vi "Teperature and FIeld Sweep_1022D.vi"() -> ()   [LabVIEW 2022 SP3]
uses:
  <vilib>/Analysis/baseanly.llb/Mean (DBL).vi
  <vilib>/Utility/file.llb/Write Delimited Spreadsheet (DBL).vi
  <vilib>/Analysis/NI_AALBase.lvlib
panel:
  out "Ri_2 phase":cluster{dbl[], dbl[]}(graph)={[0.09999999999999998, 0.12, 0.14, 0.16000000000000003, 0.17999999999999994, 0.19999999999999996, 0.21999999999999997, 0.24, 0.26, 0.28, 0.29999999999999993, 0.31999999999999995, 0.33999999999999997, 0.36, 0.38, 0.4, 0.42000000000000004, 0.43999999999999995, 0.45999999999999996, 0.48, 0.5, 0.52, 0.54, 0.56, 0.5800000000000001, 0.6, 0.62, 0.64, 0.6599999999999999, 0.6799999999999999, 0.7, 0.72, 0.74, 0.76, 0.78, 0.8, 0.8200000000000001, 0.84, 0.86, 0.88, 0.9, 0.92, 0.94, 0.96, 0.98, 1.0, 0.98, 0.96, 0.94, 0.92, 0.9, 0.88, 0.86, 0.84, 0.82, 0.8, 0.78, 0.76, 0.74, 0.72, 0.7, 0.6799999999999999, 0.66, 0.64, 0.62, 0.6, 0.58, 0.56, 0.54, 0.52, 0.5, 0.48, 0.45999999999999996, 0.44000000000000006, 0.42000000000000004, 0.4, 0.38, 0.36, 0.33999999999999997, 0.32, 0.30000000000000004, 0.28, 0.26, 0.24000000000000002, 0.22, 0.2, 0.18, 0.16, 0.14, 0.12000000000000001, 0.1, 0.09999999999999998, 0.12, 0.14, 0.16000000000000003, 0.17999999999999994, 0.19999999999999996, 0.21999999999999997, 0.24, 0.26, 0.28, 0.29999999999999993, 0.31999999999999995, 0.33999999999999997, 0.36, 0.38, 0.4, 0.42000000000000004, 0.43999999999999995, 0.45999999999999996, 0.48, 0.5, 0.52, 0.54, 0.56, 0.5800000000000001, 0.6, 0.62, 0.64, 0.6599999999999999, 0.6799999999999999, 0.7, 0.72, 0.74, 0.76, 0.78, 0.8, 0.8200000000000001, 0.84, 0.86, 0.88, 0.9, 0.92, 0.94, 0.96, 0.98, 1.0, 0.98, 0.96, 0.94, 0.92, 0.9, 0.88, 0.86, 0.84, 0.82, 0.8, 0.78, 0.76, 0.74, 0.72, 0.7, 0.6799999999999999, 0.66, 0.64, 0.62, 0.6, 0.58, 0.56, 0.54, 0.52, 0.5, 0.48, 0.45999999999999996, 0.44000000000000006, 0.42000000000000004, 0.4, 0.38, 0.36, 0.33999999999999997, 0.32, 0.30000000000000004, 0.28, 0.26, 0.24000000000000002, 0.22, 0.2, 0.18, 0.16, 0.14, 0.12000000000000001, 0.1], [117.62016846841588, 117.96664882272376, 118.35478696482726, 118.61912016643541, 118.76956664586604, 118.95054910823121, 119.01498123375443, 119.16872489157113, 119.24431424706378, 119.34190104277982, 119.41733225392822, 119.45140264855945, 119.53984114559682, 119.55691764422741, 119.59487520871042, 119.6750795139146, 119.68579169001923, 119.73065237331134, 119.74423324815396, 119.7661994334273, 119.80750346193834, 119.83623494650696, 119.82452268397942, 119.85627567058157, 119.86835371539776, 119.89360726965279, 119.90311700886441, 119.93603473890582, 119.94528450180692, 119.95000862999613, 119.95960465948625, 119.9830178122235, 119.97849406894788, 119.98959200475136, 119.99632464219606, 119.98257095958301, 120.01347012367368, 120.03103870555512, 120.04478039338926, 120.06360222149044, 120.05061637114048, 120.06363439063853, 120.07171311867637, 120.0757793318229, 120.09113199025303, 120.10726896331157, 120.06234962658894, 120.07718932923174, 120.09075423852748, 120.08476253619433, 120.05873660804704, 120.07529089338618, 120.07073006886651, 120.06602997484751, 120.06644594382928, 120.05437893498467, 120.0559832066358, 120.05241197254445, 120.03496471192462, 120.04190874507303, 120.04592984925304, 120.02590122679835, 120.02106762290221, 120.0170754772018, 120.01717601945583, 119.99024830583144, 119.98050754517847, 119.98548510957906, 119.96626810243879, 119.94421874372571, 119.91496186190318, 119.90254071057821, 119.89802448935203, 119.86225587700838, 119.84782030921231, 119.76071599522875, 119.78171218684165, 119.52712081973637, 119.68947818038498, 119.64888776868774, 119.54538024283588, 119.49187757183782, 119.40373568864177, 119.34094898550048, 119.25703379849283, 119.03268380413638, 118.93848534047406, 118.66368000738926, 118.3703709122756, 118.00894457485364, 117.8022869674905, 117.83191820734878, 118.35839994290589, 118.74306406859516, 118.97978381368443, 119.0832443256442, 119.22408053378842, 119.3756798875886, 119.42654507577663, 119.54312088447948, 119.65528936579355, 119.68067384348709, 119.73888591320637, 119.7746550722424, 119.83575660206921, 119.87436287491752, 119.92090575023776, 119.96360858392154, 119.97618916031327, 120.0270490763764, 120.03660757353578, 120.04594971613244, 120.07374861282088, 120.08502945701846, 120.11904718233538, 120.12373738373853, 120.13187955586031, 120.15078785675374, 120.16051712055169, 120.18138633972099, 120.18855573342282, 120.20283710115059, 120.21752926335739, 120.2286670939815, 120.25005622275296, 120.26083012867937, 120.26435687292016, 120.25219743715516, 120.27247788976976, 120.27728128431886, 120.30980987455453, 120.3013104315504, 120.30956542774932, 120.32575192936613, 120.32481345899741, 120.34376176879596, 120.32045496743885, 120.31980339045367, 120.31350527912403, 120.31252525198906, 120.3242014431218, 120.34462619894298, 120.32098729633576, 120.3242809008918, 120.31759933903815, 120.34279447419958, 120.29133105012681, 120.2971043007052, 120.2915107827317, 120.30887402170481, 120.3132908103599, 120.29180381456831, 120.29677581115975, 120.25488350003204, 120.25012405536286, 120.24749071884021, 120.20434065293489, 120.23689420155657, 120.20258149493482, 120.19465503125453, 120.16140368284456, 120.17158365673114, 120.12877813062116, 120.10707856478476, 120.07296661494834, 120.03335070293379, 120.02574871514983, 119.97110769112416, 120.18824358128647, 119.87610802993717, 119.85772779265321, 119.77209829112437, 119.73583766352138, 119.65849570448214, 119.57056721383769, 119.43100181965622, 119.2628284467831, 119.0562851102115, 118.80762144883226, 118.56712932086603, 117.71722366335914, 116.41351313841975, 116.41351313841975]}
  out "Ri_1 phase":cluster{dbl[], dbl[]}(graph)={[0.09999999999999998, 0.12, 0.14, 0.16000000000000003, 0.17999999999999994, 0.19999999999999996, 0.21999999999999997, 0.24, 0.26, 0.28, 0.29999999999999993, 0.31999999999999995, 0.33999999999999997, 0.36, 0.38, 0.4, 0.42000000000000004, 0.43999999999999995, 0.45999999999999996, 0.48, 0.5, 0.52, 0.54, 0.56, 0.5800000000000001, 0.6, 0.62, 0.64, 0.6599999999999999, 0.6799999999999999, 0.7, 0.72, 0.74, 0.76, 0.78, 0.8, 0.8200000000000001, 0.84, 0.86, 0.88, 0.9, 0.92, 0.94, 0.96, 0.98, 1.0, 0.98, 0.96, 0.94, 0.92, 0.9, 0.88, 0.86, 0.84, 0.82, 0.8, 0.78, 0.76, 0.74, 0.72, 0.7, 0.6799999999999999, 0.66, 0.64, 0.62, 0.6, 0.58, 0.56, 0.54, 0.52, 0.5, 0.48, 0.45999999999999996, 0.44000000000000006, 0.42000000000000004, 0.4, 0.38, 0.36, 0.33999999999999997, 0.32, 0.30000000000000004, 0.28, 0.26, 0.24000000000000002, 0.22, 0.2, 0.18, 0.16, 0.14, 0.12000000000000001, 0.1, 0.09999999999999998, 0.12, 0.14, 0.16000000000000003, 0.17999999999999994, 0.19999999999999996, 0.21999999999999997, 0.24, 0.26, 0.28, 0.29999999999999993, 0.31999999999999995, 0.33999999999999997, 0.36, 0.38, 0.4, 0.42000000000000004, 0.43999999999999995, 0.45999999999999996, 0.48, 0.5, 0.52, 0.54, 0.56, 0.5800000000000001, 0.6, 0.62, 0.64, 0.6599999999999999, 0.6799999999999999, 0.7, 0.72, 0.74, 0.76, 0.78, 0.8, 0.8200000000000001, 0.84, 0.86, 0.88, 0.9, 0.92, 0.94, 0.96, 0.98, 1.0, 0.98, 0.96, 0.94, 0.92, 0.9, 0.88, 0.86, 0.84, 0.82, 0.8, 0.78, 0.76, 0.74, 0.72, 0.7, 0.6799999999999999, 0.66, 0.64, 0.62, 0.6, 0.58, 0.56, 0.54, 0.52, 0.5, 0.48, 0.45999999999999996, 0.44000000000000006, 0.42000000000000004, 0.4, 0.38, 0.36, 0.33999999999999997, 0.32, 0.30000000000000004, 0.28, 0.26, 0.24000000000000002, 0.22, 0.2, 0.18, 0.16, 0.14, 0.12000000000000001, 0.1], [-151.82022434949218, -151.31250474861076, -150.934829382567, -150.48587961112963, -150.35129794100732, -150.20108675684463, -150.07301012387398, -149.85371662190408, -149.80643007097768, -149.6778115966004, -149.70631232196195, -149.3427081876464, -144.00790971737905, -149.75303510022803, -149.67465048111166, -149.61059645892314, -149.5755216627079, -149.56032591732512, -149.56777135196236, -149.53038555798872, -149.4837567137922, -149.46653630858634, -149.4555130589029, -149.44977309701568, -149.46602213201024, -149.42050625632652, -149.44267585686146, -149.44000832559337, -149.42583379539636, -149.39692572431568, -149.40442155131146, -149.40915566881102, -149.38050614114596, -149.38240574949845, -149.3953243906204, -149.3899047221218, -149.38685008550175, -149.37072119411883, -149.37324923858517, -149.36914979835484, -149.37390639605138, -149.3980165878626, -149.38623806135408, -149.35518531108906, -149.37819742529774, -149.37025076997705, -149.37797439572273, -149.4274062049048, -149.39553532551332, -149.39989159256442, -149.40788326839706, -149.4035269042052, -149.42173829217444, -149.42516481564763, -149.4219167404996, -149.46356168834444, -149.4516805103338, -149.45047160544362, -149.45716135037998, -149.47450752769095, -149.4832252279336, -149.49183740199788, -149.51226639630787, -149.525555046651, -149.5573781565128, -149.5590093788641, -149.5858478680793, -149.5557150450339, -149.61888489114702, -149.65084954099694, -149.65437010384474, -149.69488018826033, -149.69116543387327, -149.7564704385459, -149.77576215560174, -149.78827998741025, -150.21783070990878, -156.94726445856756, -149.75208834187845, -149.79358735688876, -149.81920487838278, -149.97644416993913, -150.0531791626578, -150.16748042818656, -150.30076394633943, -150.44483707228213, -150.66626270081673, -151.04929447184827, -151.43411807203063, -151.97278023054187, -152.18821211537258, -152.14623356637654, -151.4719825276092, -150.96302427747355, -150.84756504567386, -150.5037700822142, -150.3245640418613, -150.17713325364664, -150.1036649225191, -149.99036753477975, -149.85697295444248, -149.8501754093205, -149.56080314237312, -146.67158122655187, -149.96749106410877, -149.93190810259412, -149.9232306144384, -149.8834345316244, -149.82170489643204, -149.7789775276986, -149.77872756893103, -149.7707527140453, -149.75157225999848, -149.7012296966859, -149.71638923850873, -149.69938903054089, -149.67312320269653, -149.69041977164406, -149.6838198853977, -149.66161778220618, -149.6546278866485, -149.640923821836, -149.6728863842432, -149.66791865505627, -149.62858582517933, -149.64183587402476, -149.6484558455101, -149.6427424788427, -149.6296817347956, -149.63395082883616, -149.62713187401155, -149.6182616601406, -149.65041315650092, -149.62494744989198, -149.61909696518853, -149.6175044512262, -149.6371509732279, -149.66137383135944, -149.63515614075328, -149.6451064613961, -149.65811060587708, -149.64909805431552, -149.6696824809014, -149.66829454461902, -149.65211834334818, -149.6792564836343, -149.69346020858046, -149.7169451406854, -149.71160254963883, -149.72665337378038, -149.73853617494782, -149.73020826238755, -149.75385526179556, -149.7724664962522, -149.77034769159013, -149.80481526391884, -149.81816596924764, -149.87205062927146, -149.86012342940273, -149.90891882509268, -149.92420949696478, -149.94160073513336, -149.98031714888242, -149.98297286567293, -150.01739729399605, -150.0978801191893, -150.09675943096, -149.9722562160305, -148.8947110005267, -150.0746278787694, -150.12829367372765, -150.21097166683603, -150.2349660580826, -150.3575760488762, -150.49529547074826, -150.72432289368865, -150.81632873807234, -151.05780214090098, -151.3722097867961, -151.68469888569936, -152.04933901054727, -152.04933901054727]}
  out "Ri_2":cluster{dbl[], dbl[]}(graph)={[0.09999999999999998, 0.12, 0.14, 0.16000000000000003, 0.17999999999999994, 0.19999999999999996, 0.21999999999999997, 0.24, 0.26, 0.28, 0.29999999999999993, 0.31999999999999995, 0.33999999999999997, 0.36, 0.38, 0.4, 0.42000000000000004, 0.43999999999999995, 0.45999999999999996, 0.48, 0.5, 0.52, 0.54, 0.56, 0.5800000000000001, 0.6, 0.62, 0.64, 0.6599999999999999, 0.6799999999999999, 0.7, 0.72, 0.74, 0.76, 0.78, 0.8, 0.8200000000000001, 0.84, 0.86, 0.88, 0.9, 0.92, 0.94, 0.96, 0.98, 1.0, 0.98, 0.96, 0.94, 0.92, 0.9, 0.88, 0.86, 0.84, 0.82, 0.8, 0.78, 0.76, 0.74, 0.72, 0.7, 0.6799999999999999, 0.66, 0.64, 0.62, 0.6, 0.58, 0.56, 0.54, 0.52, 0.5, 0.48, 0.45999999999999996, 0.44000000000000006, 0.42000000000000004, 0.4, 0.38, 0.36, 0.33999999999999997, 0.32, 0.30000000000000004, 0.28, 0.26, 0.24000000000000002, 0.22, 0.2, 0.18, 0.16, 0.14, 0.12000000000000001, 0.1, 0.09999999999999998, 0.12, 0.14, 0.16000000000000003, 0.17999999999999994, 0.19999999999999996, 0.21999999999999997, 0.24, 0.26, 0.28, 0.29999999999999993, 0.31999999999999995, 0.33999999999999997, 0.36, 0.38, 0.4, 0.42000000000000004, 0.43999999999999995, 0.45999999999999996, 0.48, 0.5, 0.52, 0.54, 0.56, 0.5800000000000001, 0.6, 0.62, 0.64, 0.6599999999999999, 0.6799999999999999, 0.7, 0.72, 0.74, 0.76, 0.78, 0.8, 0.8200000000000001, 0.84, 0.86, 0.88, 0.9, 0.92, 0.94, 0.96, 0.98, 1.0, 0.98, 0.96, 0.94, 0.92, 0.9, 0.88, 0.86, 0.84, 0.82, 0.8, 0.78, 0.76, 0.74, 0.72, 0.7, 0.6799999999999999, 0.66, 0.64, 0.62, 0.6, 0.58, 0.56, 0.54, 0.52, 0.5, 0.48, 0.45999999999999996, 0.44000000000000006, 0.42000000000000004, 0.4, 0.38, 0.36, 0.33999999999999997, 0.32, 0.30000000000000004, 0.28, 0.26, 0.24000000000000002, 0.22, 0.2, 0.18, 0.16, 0.14, 0.12000000000000001, 0.1], [12.205176752147196, 12.33738736524411, 12.436814472113113, 12.543061919618381, 12.591177109870843, 12.63204488402351, 12.633074379656962, 12.678587031476285, 12.702366812156168, 12.734766256641889, 12.764822745445459, 12.798115074151369, 12.56005416503157, 12.811022273559901, 12.805614848037402, 12.822742652741233, 12.833360063934796, 12.844414076677566, 12.853037374725659, 12.863749846343488, 12.873727971040198, 12.87545677652524, 12.884395543563812, 12.901595012846315, 12.91020558633629, 12.91700210310611, 12.916182386400777, 12.932745625307929, 12.929132177243485, 12.939245398543807, 12.945904132779514, 12.979271768015096, 12.951619927398129, 12.963100847085817, 12.961454764152798, 12.968676853276186, 13.035314574413999, 12.968769140450755, 12.976857768700619, 12.982937075765706, 12.987156955464599, 12.987225357622929, 12.990469558247861, 13.001074140628084, 13.015805070701896, 13.213316441028162, 13.212674850256546, 13.214497097772925, 13.213097914485022, 13.212520778890907, 13.217287379489568, 13.224571659209413, 13.221461422183241, 13.21249046212996, 13.231625931101464, 13.219596872719654, 13.230780717880945, 13.231496283261466, 13.228879184378412, 13.236537684484286, 13.2442021665191, 13.245327395573094, 13.239075527873267, 13.250459225400578, 13.254010022147359, 13.263592058540043, 13.278201777756056, 13.271280645160415, 13.28286228675346, 13.287261154844275, 13.290082368268422, 13.30492697157085, 13.325287026560359, 13.337097306813405, 13.334459335710374, 13.36121908059594, 13.349781951942722, 13.590657500379482, 13.420711749521754, 13.427055186068772, 13.476488972924022, 13.504746276159453, 13.521802810703734, 13.585085247505193, 13.63738342595085, 13.703337851038048, 13.791442558469074, 13.849252925446702, 13.98837153260088, 14.058767459755813, 13.057484778983863, 12.424975150602982, 12.341214474536581, 12.597671651852279, 12.547100753140823, 12.603242737801498, 12.610091337495355, 12.662729976248402, 12.683644441406994, 12.707706571670649, 12.74751634316906, 12.764099115085513, 12.803871979165852, 12.693242845243883, 12.809727121728208, 12.817180050708686, 12.831651755770647, 12.839364718018068, 12.860298160932963, 12.896827552552299, 12.864701328486037, 12.883685199780242, 12.884793998467885, 12.902011985965638, 12.898401964032054, 12.906219259474547, 12.914228868687658, 12.911587003388147, 12.958793693981802, 12.933506906195795, 12.933859306721546, 12.94206688909155, 12.946106387292451, 12.954120795402451, 12.95420497189929, 12.961692049093307, 12.970243175218398, 12.966251377610806, 12.971030269555348, 12.980713661496962, 12.983816343381182, 12.98792173316417, 12.995117688102317, 13.000724459135895, 13.003773018187172, 13.013804312695264, 13.221409487304983, 13.213732944734987, 13.219930146403511, 13.2160660705417, 13.220288758106749, 13.225356431589839, 13.221627768983318, 13.192042140412925, 13.225457206093656, 13.224404733921627, 13.226943621029603, 13.22188486286242, 13.239906219746997, 13.23627215525837, 13.23780083001927, 13.24191338088606, 13.243188029364342, 13.248586751116793, 13.24553444444596, 13.263702564618967, 13.263180218458823, 13.265510887371871, 13.27580985473867, 13.285902114226138, 13.285290341366075, 13.292004389335341, 13.320520276023231, 13.32468083832859, 13.320587416172566, 13.3596713753944, 13.351640175534053, 13.311511157505569, 13.749204463952886, 13.417895997650705, 13.439008654275602, 13.464312581366862, 13.491545253041302, 13.546146393015691, 13.560171412898399, 13.584913714835219, 13.647701856221694, 13.605003489243288, 13.892818025978201, 13.94644999851722, 14.42599048649726, 102.36268705136854, 102.36268705136854]}
  out "Ri_1":cluster{dbl[], dbl[]}(graph)={[0.09999999999999998, 0.12, 0.14, 0.16000000000000003, 0.17999999999999994, 0.19999999999999996, 0.21999999999999997, 0.24, 0.26, 0.28, 0.29999999999999993, 0.31999999999999995, 0.33999999999999997, 0.36, 0.38, 0.4, 0.42000000000000004, 0.43999999999999995, 0.45999999999999996, 0.48, 0.5, 0.52, 0.54, 0.56, 0.5800000000000001, 0.6, 0.62, 0.64, 0.6599999999999999, 0.6799999999999999, 0.7, 0.72, 0.74, 0.76, 0.78, 0.8, 0.8200000000000001, 0.84, 0.86, 0.88, 0.9, 0.92, 0.94, 0.96, 0.98, 1.0, 0.98, 0.96, 0.94, 0.92, 0.9, 0.88, 0.86, 0.84, 0.82, 0.8, 0.78, 0.76, 0.74, 0.72, 0.7, 0.6799999999999999, 0.66, 0.64, 0.62, 0.6, 0.58, 0.56, 0.54, 0.52, 0.5, 0.48, 0.45999999999999996, 0.44000000000000006, 0.42000000000000004, 0.4, 0.38, 0.36, 0.33999999999999997, 0.32, 0.30000000000000004, 0.28, 0.26, 0.24000000000000002, 0.22, 0.2, 0.18, 0.16, 0.14, 0.12000000000000001, 0.1, 0.09999999999999998, 0.12, 0.14, 0.16000000000000003, 0.17999999999999994, 0.19999999999999996, 0.21999999999999997, 0.24, 0.26, 0.28, 0.29999999999999993, 0.31999999999999995, 0.33999999999999997, 0.36, 0.38, 0.4, 0.42000000000000004, 0.43999999999999995, 0.45999999999999996, 0.48, 0.5, 0.52, 0.54, 0.56, 0.5800000000000001, 0.6, 0.62, 0.64, 0.6599999999999999, 0.6799999999999999, 0.7, 0.72, 0.74, 0.76, 0.78, 0.8, 0.8200000000000001, 0.84, 0.86, 0.88, 0.9, 0.92, 0.94, 0.96, 0.98, 1.0, 0.98, 0.96, 0.94, 0.92, 0.9, 0.88, 0.86, 0.84, 0.82, 0.8, 0.78, 0.76, 0.74, 0.72, 0.7, 0.6799999999999999, 0.66, 0.64, 0.62, 0.6, 0.58, 0.56, 0.54, 0.52, 0.5, 0.48, 0.45999999999999996, 0.44000000000000006, 0.42000000000000004, 0.4, 0.38, 0.36, 0.33999999999999997, 0.32, 0.30000000000000004, 0.28, 0.26, 0.24000000000000002, 0.22, 0.2, 0.18, 0.16, 0.14, 0.12000000000000001, 0.1], [2087.542522514706, 2143.3806726181297, 2192.1505680332307, 2224.5398110134415, 2254.2076727564463, 2283.219391571736, 2295.5351896243988, 2312.274969759326, 2321.1906487058636, 2258.618428233254, 2439.815278150036, 2363.114732601407, 2569.2987357483867, 2366.69462809311, 2370.3526096767628, 2370.7532832147513, 2369.446453774161, 2372.3479615014453, 2373.7967150363133, 2373.3912011059742, 2374.3898629584414, 2373.19922105906, 2374.08711510194, 2374.3447992304204, 2372.719181172187, 2372.5831623830313, 2368.606666524962, 2368.1271954116123, 2368.1587157781582, 2368.364263936688, 2363.1239774166042, 2363.4322755470225, 2359.5286066627255, 2362.2730811990377, 2355.540999658394, 2354.6901938211345, 2338.3987997031136, 2348.956030561271, 2348.6720464600826, 2345.47931492513, 2343.641628918994, 2322.579102266805, 2357.7528780540633, 2337.9624461876765, 2337.035655864342, 2390.13340514578, 2393.333076080936, 2397.194891434832, 2400.4646152722025, 2404.1840381335187, 2406.4647119031993, 2411.655350773428, 2414.452737749684, 2416.491207784975, 2422.152414810807, 2426.43445652573, 2430.4661399145198, 2472.9095612064084, 2401.2074203638863, 2442.381915486605, 2447.39053615182, 2448.9505311169605, 2454.873847352734, 2458.903517524707, 2461.995925756737, 2467.061840825975, 2470.520942891029, 2474.931087852616, 2483.997180170197, 2486.4806066909064, 2489.8094006815363, 2495.4829515630936, 2496.5109281850623, 2499.717712613259, 2508.0628602511415, 2587.583625405099, 2446.457085912187, 2744.1467541037973, 2527.145831911331, 2528.3781519262234, 2531.0945072462814, 2536.7135748602786, 2544.038687449601, 2544.827299932163, 2546.39588450735, 2552.3831526464273, 2560.7487646591876, 2557.6068386083666, 2541.8036010528517, 2556.5211525031086, 2275.4515181505535, 2236.3211050589766, 2137.0989873521185, 2148.4934229155265, 2226.3795783020046, 2259.8236048661397, 2277.518588977397, 2298.2309636749364, 2311.745843167506, 2328.4510173480307, 2336.560722824512, 2344.24126014681, 2362.7311144000346, 2627.003456834187, 2364.144130172327, 2369.8717620699094, 2373.0451002371196, 2373.971931289017, 2377.1037991880976, 2381.4533155017552, 2376.2465418035545, 2376.4643282086604, 2373.1094722464964, 2373.683408097068, 2373.6902390420423, 2372.436584742077, 2372.7068819175765, 2370.444178339574, 2369.7303118006134, 2368.9013786355426, 2364.66910807676, 2363.1277468576277, 2362.1693752579, 2359.8572707523836, 2358.3637082703754, 2356.2088803095526, 2354.2381091107436, 2352.2504633571566, 2349.807036392201, 2348.000550307495, 2345.2605399911095, 2343.048947126772, 2342.138893566093, 2338.647207375316, 2337.823575605664, 2336.4325858086618, 2391.3050818760403, 2393.854078139158, 2397.3144621611436, 2400.183701016868, 2404.559873121706, 2408.113986664911, 2411.3881576090257, 2422.2503149813315, 2418.4477629937755, 2423.424584031643, 2427.359469208306, 2429.5536317154106, 2435.189541439222, 2439.3273653599067, 2443.6532125172207, 2446.4799477219917, 2450.5183688798943, 2455.1086830020786, 2469.17017360265, 2463.7910814680667, 2466.142256138314, 2475.164122601692, 2480.58039686262, 2485.3434347885513, 2489.254932267259, 2490.995762828881, 2496.288772114335, 2501.89872487851, 2502.665922214194, 2507.8176213420734, 2510.8951882690485, 2514.6646388029453, 2515.90870103181, 2526.343933365244, 2527.8233287119538, 2535.9588766433053, 2534.614384395244, 2541.4565246972834, 2550.357749348691, 2549.473660870641, 2558.3365999756966, 2604.730472408435, 2561.1991565610233, 2554.929997465301, 2611.611284193903, 2611.611284193903]}
  out "Ri_2(Ohm)":dbl=12.205176752147196
  out "Ri_1(Ohm)":dbl=2087.542522514706
  in  "R2 Sensitivity":u16(ring)=26 items=["1 nV/fA", "2 nV/fA", "5 nV/fA", "10 nV/fA", "20 nV/fA", "50 nV/fA", "100 nV/fA", "200 nV/fA", "500 nV/fA", "1 uV/pA", "2 uV/pA", "5 uV/pA", "10 uV/pA", "20 uV/pA", "50 uV/pA", "100 uV/pA", "200 uV/pA", "500 uV/pA", "1 mV/nA", "2 mV/nA", "5 mV/nA", "10 mV/nA", "20 mV/nA", "50 mV/nA", "100 mV/nA", "200 mV/nA", "500 mV/nA", "1 V/uA"]
  in  "R2 Current T Constant":u8(ring)=9 items=["10 us", "30 us", "100 us", "300 us", "1 ms", "3 ms", "10 ms", "30 ms", "100 ms", "300 ms", "1 s", "3 s", "10 s", "30 s", "100 s", "300 s", "1 ks", "3 ks"]
  in  "R1 Current T Constant":u8(ring)=9 items=["10 us", "30 us", "100 us", "300 us", "1 ms", "3 ms", "10 ms", "30 ms", "100 ms", "300 ms", "1 s", "3 s", "10 s", "30 s", "100 s", "300 s", "1 ks", "3 ks"]
  in  "R1 Current sensitivity":u16(ring)=26 items=["1 nV/fA", "2 nV/fA", "5 nV/fA", "10 nV/fA", "20 nV/fA", "50 nV/fA", "100 nV/fA", "200 nV/fA", "500 nV/fA", "1 uV/pA", "2 uV/pA", "5 uV/pA", "10 uV/pA", "20 uV/pA", "50 uV/pA", "100 uV/pA", "200 uV/pA", "500 uV/pA", "1 mV/nA", "2 mV/nA", "5 mV/nA", "10 mV/nA", "20 mV/nA", "50 mV/nA", "100 mV/nA", "200 mV/nA", "500 mV/nA", "1 V/uA"]
  in  "LOCKIN3 address":refnum<visa-resource-name>="COM5"
  in  "Current measurement?":bool=TRUE
  in  "R2(Kohm)":dbl=1.9997 format="%#_13g"
  in  "R1(Kohm)":dbl=2.0265 format="%#_13g"
  out "Device 1 phase":dbl=-151.82022434949218 format="%.3p"
  out "Device 2 phase":dbl=117.62016846841588 format="%.3p"
  out "Device1 Current(mA)":dbl=0.0003122594054162884
  out "Device2 Current(mA)":dbl=0.015138421665849215
  in  "Sine Output Amplitude (V)":sgl=0.5
  out "Vab_1_F 2w":cluster{dbl[], dbl[]}(graph)
  out "Phase Vab_1_F 2w":cluster{dbl[], dbl[]}(graph)
  out "Vab_1_F (uV) 2w":dbl format="%.3p"
  out "Phase Vab_1_F 2w":dbl format="%.3p"
  in  "Phase 1B 3":u16(ring)=9 items=["X", "Y", "R", "Theta", "Frequency", "Noise", "Xh1", "Yh1", "Rh1", "Theta h1", "Xh2", "Yh2", "Rh2", "Theta h2"]
  in  "Parameter 1B 3":u16(ring)=8 items=["X", "Y", "R", "Theta", "Frequency", "Noise", "Xh1", "Yh1", "Rh1", "Theta h1", "Xh2", "Yh2", "Rh2", "Theta h2"]
  out "Vab_2_F  2w":cluster{dbl[], dbl[]}(graph)
  out "Phase Vab_2_F 2w":cluster{dbl[], dbl[]}(graph)
  out "Vab_2_F (uV) 2w":dbl format="%.3p"
  out "Phase Vab_2_F 2w":dbl format="%.6g"
  in  "Phase 2B 3":u16(ring)=9 items=["X", "Y", "R", "Theta", "Frequency", "Noise", "Xh1", "Yh1", "Rh1", "Theta h1", "Xh2", "Yh2", "Rh2", "Theta h2"]
  in  "Parameter 2B 3":u16(ring)=8 items=["X", "Y", "R", "Theta", "Frequency", "Noise", "Xh1", "Yh1", "Rh1", "Theta h1", "Xh2", "Yh2", "Rh2", "Theta h2"]
  in  "Starting Point (Oe)":dbl
  out "phase Vaa_2_F":cluster{dbl[], dbl[]}(graph)={[0.1], [0.0]}
  out "Vaa_2_F":cluster{dbl[], dbl[]}(graph)={[0.1], [0.0]}
  out "phase Vab_2_F 1w":cluster{dbl[], dbl[]}(graph)
  out "Vab_2_F 1w":cluster{dbl[], dbl[]}(graph)={[0.1], [0.0]}
  out "phase Vab_2_F 1w":dbl
  in  "Phase 2B 2":u16(ring)=3 items=["X", "Y", "R", "Theta", "Frequency", "Noise", "Xh1", "Yh1", "Rh1", "Theta h1", "Xh2", "Yh2", "Rh2", "Theta h2"]
  out "phase Vaa_2_F":dbl
  in  "Phase 2A  2":u16(ring)=3 items=["X", "Y", "R", "Theta", "Frequency", "Noise", "Xh1", "Yh1", "Rh1", "Theta h1", "Xh2", "Yh2", "Rh2", "Theta h2"]
  out "Vaa_2_F (mV)":dbl
  in  "F Clear Plot 2A":bool
  in  "Parameter 2A 2":u16(ring)=2 items=["X", "Y", "R", "Theta", "Frequency", "Noise", "Xh1", "Yh1", "Rh1", "Theta h1", "Xh2", "Yh2", "Rh2", "Theta h2"]
  out "Vab_2_F (uV) 1w":dbl
  in  "F Clear Plot 2B":bool
  in  "Parameter 2B 2":u16(ring)=2 items=["X", "Y", "R", "Theta", "Frequency", "Noise", "Xh1", "Yh1", "Rh1", "Theta h1", "Xh2", "Yh2", "Rh2", "Theta h2"]
  in  "path2 (folder + filename)":string="G:\\My Drive\\Opticool\\Measurement\\TF dependence\\TaI28_A1215_B1211"
  out "XY Graph 8":cluster{dbl[], dbl[]}(graph)={[0.1], [0.0]}
  out "XY Graph 7":cluster{dbl[], dbl[]}(graph)={[0.1], [0.0]}
  out "XY Graph 6":cluster{dbl[], dbl[]}(graph)
  out "XY Graph 5":cluster{dbl[], dbl[]}(graph)={[0.1], [0.0]}
  out "phase 2B":dbl
  in  "Phase 2B":u16(ring)=3 items=["X", "Y", "R", "Theta", "Frequency", "Noise", "Xh1", "Yh1", "Rh1", "Theta h1", "Xh2", "Yh2", "Rh2", "Theta h2"]
  out "phase 2A":dbl
  in  "Phase 2A":u16(ring)=3 items=["X", "Y", "R", "Theta", "Frequency", "Noise", "Xh1", "Yh1", "Rh1", "Theta h1", "Xh2", "Yh2", "Rh2", "Theta h2"]
  out "para2A Measurement":dbl
  in  "T Clear Plot 2A":bool
  in  "Parameter 2A":u16(ring)=2 items=["X", "Y", "R", "Theta", "Frequency", "Noise", "Xh1", "Yh1", "Rh1", "Theta h1", "Xh2", "Yh2", "Rh2", "Theta h2"]
  out "para2B Measurement":dbl
  in  "T Clear Plot 2B":bool
  in  "Parameter 2B":u16(ring)=2 items=["X", "Y", "R", "Theta", "Frequency", "Noise", "Xh1", "Yh1", "Rh1", "Theta h1", "Xh2", "Yh2", "Rh2", "Theta h2"]
  in  "2B frequency 2":dbl=17.7 format="%#_13g"
  in  "2B Input Connection (0: Single-Ended)":u16(ring)=1 items=["Single-Ended Voltage", "Differential Voltage", "1 MOhm Current Gain", "100 MOhm Current Gain"]
  in  "2B harmonic 1":u8=2
  in  "2B harmonic 2":u8=3
  in  "2B reference Manual Phase":dbl
  in  "auto phase 2B":bool=TRUE
  in  "2B Sample time (s)":dbl=0.001 min=0.001 max=100.0 step=0.001
  in  "2B Sensitivity":u16(ring)=26 items=["1 nV/fA", "2 nV/fA", "5 nV/fA", "10 nV/fA", "20 nV/fA", "50 nV/fA", "100 nV/fA", "200 nV/fA", "500 nV/fA", "1 uV/pA", "2 uV/pA", "5 uV/pA", "10 uV/pA", "20 uV/pA", "50 uV/pA", "100 uV/pA", "200 uV/pA", "500 uV/pA", "1 mV/nA", "2 mV/nA", "5 mV/nA", "10 mV/nA", "20 mV/nA", "50 mV/nA", "100 mV/nA", "200 mV/nA", "500 mV/nA", "1 V/uA"]
  in  "Enable Sync Filter 2B (when f<200Hz)":bool
  in  "2B Time Constant":u8(ring)=9 items=["10 us", "30 us", "100 us", "300 us", "1 ms", "3 ms", "10 ms", "30 ms", "100 ms", "300 ms", "1 s", "3 s", "10 s", "30 s", "100 s", "300 s", "1 ks", "3 ks"]
  in  "2B Reference Source":u8(ring) items=["External", "Internal", "Internal Sweep", "Channel-A"]
  in  "2B Low Pass Filter Slope":u8(ring)=2 items=["6 dB/oct", "12 dB/oct", "18 db/oct", "24 dB/oct"]
  in  "2A frequency":dbl=17.7 format="%#_13g"
  in  "2A Input Connection (0: Single-Ended)":u16(ring)=1 items=["Single-Ended Voltage", "Differential Voltage", "1 MOhm Current Gain", "100 MOhm Current Gain"]
  in  "2A harmonic 2":u8=2
  in  "2A harmonic":u8=3
  in  "2A reference Manual Phase":dbl
  in  "auto phase 2A":bool=TRUE
  in  "2A Reference Source":u8(ring) items=["External", "Internal", "Internal Sweep"]
  in  "2A Sample time (s)":dbl=0.001 min=0.001 max=100.0 step=0.001
  in  "2A Time Constant":u8(ring)=9 items=["10 us", "30 us", "100 us", "300 us", "1 ms", "3 ms", "10 ms", "30 ms", "100 ms", "300 ms", "1 s", "3 s", "10 s", "30 s", "100 s", "300 s", "1 ks", "3 ks"]
  in  "Enable Sync Filter 2A (when f<200Hz)":bool
  in  "2A Sensitivity":u16(ring)=26 items=["1 nV/fA", "2 nV/fA", "5 nV/fA", "10 nV/fA", "20 nV/fA", "50 nV/fA", "100 nV/fA", "200 nV/fA", "500 nV/fA", "1 uV/pA", "2 uV/pA", "5 uV/pA", "10 uV/pA", "20 uV/pA", "50 uV/pA", "100 uV/pA", "200 uV/pA", "500 uV/pA", "1 mV/nA", "2 mV/nA", "5 mV/nA", "10 mV/nA", "20 mV/nA", "50 mV/nA", "100 mV/nA", "200 mV/nA", "500 mV/nA", "1 V/uA"]
  in  "2A Low Pass Filter Slope":u8(ring)=2 items=["6 dB/oct", "12 dB/oct", "18 db/oct", "24 dB/oct"]
  in  "Two Lock-in ?":bool=TRUE
  in  "LOCKIN2 address":refnum<visa-resource-name>="COM4"
  in  "?":bool
  out "Temperature Status":i32(ring)=1 items=["TemperatureUnknown"=0, "Stable"=1, "Tracking"=2, "Near"=5, "Chasing"=6, "Filling"=7, "Standby"=10, "Disabled"=13, "ImpedanceNotFunction"=14, "TempFailure"=15]
  out "Field Status":i32(ring)=4 items=["MagnetUnknown"=0, "StablePersistent"=1, "WarmingSwitch"=2, "CoolingSwitch"=3, "StableDriven"=4, "Iterating"=5, "Charging"=6, "Discharging"=7, "CurrentError"=8, "MagnetFailure"=15]
  out "Field":dbl=0.10076643899083138
  out "Temperature":dbl=2.0469605207443236
  in  "Initialize":bool
  in  "System Stablization (s)":dbl=0.5 format="%#_13g"
  in  "Low Value (Oe)":dbl=-66000.0
  in  "High Value (Oe)":dbl=66000.0
  in  "Sweep Field Approach":i32(ring) items=["Linear", "NoOvershoot", "Oscillate"]
  in  "Sweep F Rate (Oe/s)":dbl=200.0 format="%#_13g"
  in  "Sweep F mode":i32(ring) items=["Persistent", "Driven"]
  in  "Set Fixed T":dbl=2.0
  in  "Fixed Temp Approach":i32(ring)=1 items=["FastSettle", "NoOvershoot"]
  in  "FIxed T  Rate (K/min)":dbl=20.0
  out "phase Vaa_1_F":cluster{dbl[], dbl[]}(graph)
  out "Vaa_1_F":cluster{dbl[], dbl[]}(graph)
  out "phase Vab_1_F 1w":cluster{dbl[], dbl[]}(graph)
  out "Vab_1_F 1w":cluster{dbl[], dbl[]}(graph)
  out "phase Vab_1_F 1w":dbl
  in  "Phase 1B 2":u16(ring)=3 items=["X", "Y", "R", "Theta", "Frequency", "Noise", "Xh1", "Yh1", "Rh1", "Theta h1", "Xh2", "Yh2", "Rh2", "Theta h2"]
  out "phase Vaa_1_F":dbl
  in  "Phase 1A 2":u16(ring)=3 items=["X", "Y", "R", "Theta", "Frequency", "Noise", "Xh1", "Yh1", "Rh1", "Theta h1", "Xh2", "Yh2", "Rh2", "Theta h2"]
  out "Vaa_1_F (mV)":dbl=1.49013e-07
  in  "F Clear Plot 1A":bool
  in  "Parameter 1A 2":u16(ring)=2 items=["X", "Y", "R", "Theta", "Frequency", "Noise", "Xh1", "Yh1", "Rh1", "Theta h1", "Xh2", "Yh2", "Rh2", "Theta h2"]
  out "Vab_1_F (uV) 1w":dbl=1.49013e-07
  in  "F Clear Plot 1B":bool
  in  "Parameter 1B 2":u16(ring)=2 items=["X", "Y", "R", "Theta", "Frequency", "Noise", "Xh1", "Yh1", "Rh1", "Theta h1", "Xh2", "Yh2", "Rh2", "Theta h2"]
  out "Field Setting":dbl format="%#_13g"
  out "Fixed Temp":dbl
  out "Measured Field":dbl
  out "Field Status":i32(ring) items=["MagnetUnknown"=0, "StablePersistent"=1, "WarmingSwitch"=2, "CoolingSwitch"=3, "StableDriven"=4, "Iterating"=5, "Charging"=6, "Discharging"=7, "CurrentError"=8, "MagnetFailure"=15]
  out "Temp Status":i32(ring) items=["TemperatureUnknown"=0, "Stable"=1, "Tracking"=2, "Near"=5, "Chasing"=6, "Filling"=7, "Standby"=10, "Disabled"=13, "ImpedanceNotFunction"=14, "TempFailure"=15]
  out "Measuring F":bool
  in  "Step(Oe)":i32=2000
  out "F loop run":i32=1
  out "Temp Status":i32(ring) items=["TemperatureUnknown"=0, "Stable"=1, "Tracking"=2, "Near"=5, "Chasing"=6, "Filling"=7, "Standby"=10, "Disabled"=13, "ImpedanceNotFunction"=14, "TempFailure"=15]
  out "Field Status":i32(ring) items=["MagnetUnknown"=0, "StablePersistent"=1, "WarmingSwitch"=2, "CoolingSwitch"=3, "StableDriven"=4, "Iterating"=5, "Charging"=6, "Discharging"=7, "CurrentError"=8, "MagnetFailure"=15]
  out "Fixed Field":dbl
  out "Measured Temp":dbl
  in  "Delay(T/F)":dbl=5.0
  in  "Set FIxed F (Oe)":dbl format="%#_13g"
  in  "Fixed Field Approach":i32(ring) items=["Linear", "NoOvershoot", "Oscillate"]
  in  "FIxed F Rate (Oe/s)":dbl=100.0 format="%#_13g"
  in  "Fixed F mode":i32(ring) items=["Persistent", "Driven"]
  in  "Sweep Temperature Approach":i32(ring)=1 items=["FastSettle", "NoOvershoot"]
  in  "Sweep T  Rate (K/min)":dbl=10.0
  in  "Sweep T/F":bool
  in  "Remote":bool=TRUE
  in  "IP Address":string="169.254.170.239"
  out "Measuring T":bool
  in  "path1 (folder + filename)":string="G:\\My Drive\\Opticool\\Measurement\\TF dependence\\TaI27_A34_B38"
  in  "LOCKIN1 address":refnum<visa-resource-name>="COM3"
  out "Phase1A-T":cluster{dbl[], dbl[]}(graph)
  out "P1A-T":cluster{dbl[], dbl[]}(graph)
  out "Phase1B-T":cluster{dbl[], dbl[]}(graph)
  out "P1B-T":cluster{dbl[], dbl[]}(graph)
  out "phase 1B":dbl
  in  "Phase 1B":u16(ring)=3 items=["X", "Y", "R", "Theta", "Frequency", "Noise", "Xh1", "Yh1", "Rh1", "Theta h1", "Xh2", "Yh2", "Rh2", "Theta h2"]
  out "phase 1A":dbl
  in  "Phase 1A":u16(ring)=3 items=["X", "Y", "R", "Theta", "Frequency", "Noise", "Xh1", "Yh1", "Rh1", "Theta h1", "Xh2", "Yh2", "Rh2", "Theta h2"]
  out "para1A Measurement (mV)":dbl=1.49013e-07
  in  "T Clear Plot 1A":bool
  in  "Parameter 1A":u16(ring)=2 items=["X", "Y", "R", "Theta", "Frequency", "Noise", "Xh1", "Yh1", "Rh1", "Theta h1", "Xh2", "Yh2", "Rh2", "Theta h2"]
  out "para1B Measurement (uV)":dbl=1.49013e-07
  in  "T Clear Plot 1B":bool
  in  "Parameter 1B":u16(ring)=2 items=["X", "Y", "R", "Theta", "Frequency", "Noise", "Xh1", "Yh1", "Rh1", "Theta h1", "Xh2", "Yh2", "Rh2", "Theta h2"]
  out "Temp Setting":dbl format="%#_13g"
  in  "Save data or not":bool=TRUE
  in  "Step(K)":i32=10
  out "T loop run":i32
  in  "1B frequency":dbl=17.7 format="%#_13g"
  in  "1B Input Connection (0: Single-Ended)":u16(ring)=1 items=["Single-Ended Voltage", "Differential Voltage", "1 MOhm Current Gain", "100 MOhm Current Gain"]
  in  "1B harmonic 1":u8=2
  in  "1B harmonic 2":u8=3
  in  "1B reference Manual Phase":dbl
  in  "auto phase B":bool=TRUE
  in  "1B Sample time (s)":dbl=0.001 min=0.001 max=100.0 step=0.001
  in  "1B Sensitivity":u16(ring)=26 items=["1 nV/fA", "2 nV/fA", "5 nV/fA", "10 nV/fA", "20 nV/fA", "50 nV/fA", "100 nV/fA", "200 nV/fA", "500 nV/fA", "1 uV/pA", "2 uV/pA", "5 uV/pA", "10 uV/pA", "20 uV/pA", "50 uV/pA", "100 uV/pA", "200 uV/pA", "500 uV/pA", "1 mV/nA", "2 mV/nA", "5 mV/nA", "10 mV/nA", "20 mV/nA", "50 mV/nA", "100 mV/nA", "200 mV/nA", "500 mV/nA", "1 V/uA"]
  in  "Enable Sync Filter 1B (when f<200Hz)":bool
  in  "1B Time Constant":u8(ring)=9 items=["10 us", "30 us", "100 us", "300 us", "1 ms", "3 ms", "10 ms", "30 ms", "100 ms", "300 ms", "1 s", "3 s", "10 s", "30 s", "100 s", "300 s", "1 ks", "3 ks"]
  in  "1B Reference Source":u8(ring)=3 items=["External", "Internal", "Internal Sweep", "Channel-A"]
  in  "1B Low Pass Filter Slope":u8(ring)=2 items=["6 dB/oct", "12 dB/oct", "18 db/oct", "24 dB/oct"]
  in  "1A frequency":dbl=17.7 format="%#_13g"
  in  "1A Input Connection (0: Single-Ended)":u16(ring)=1 items=["Single-Ended Voltage", "Differential Voltage", "1 MOhm Current Gain", "100 MOhm Current Gain"]
  in  "1A harmonic 1":u8=2
  in  "1A harmonic 2":u8=3
  in  "1A reference Manual Phase":dbl
  in  "auto phase 1A":bool=TRUE
  in  "1A Reference Source":u8(ring)=1 items=["External", "Internal", "Internal Sweep"]
  in  "1A Sample time (s)":dbl=0.001 min=0.001 max=100.0 step=0.001
  in  "1A Time Constant":u8(ring)=9 items=["10 us", "30 us", "100 us", "300 us", "1 ms", "3 ms", "10 ms", "30 ms", "100 ms", "300 ms", "1 s", "3 s", "10 s", "30 s", "100 s", "300 s", "1 ks", "3 ks"]
  in  "Enable Sync Filter 1A (when f<200Hz)":bool
  in  "1A Sensitivity":u16(ring)=26 items=["1 nV/fA", "2 nV/fA", "5 nV/fA", "10 nV/fA", "20 nV/fA", "50 nV/fA", "100 nV/fA", "200 nV/fA", "500 nV/fA", "1 uV/pA", "2 uV/pA", "5 uV/pA", "10 uV/pA", "20 uV/pA", "50 uV/pA", "100 uV/pA", "200 uV/pA", "500 uV/pA", "1 mV/nA", "2 mV/nA", "5 mV/nA", "10 mV/nA", "20 mV/nA", "50 mV/nA", "100 mV/nA", "200 mV/nA", "500 mV/nA", "1 V/uA"]
  in  "1A Low Pass Filter Slope":u8(ring)=2 items=["6 dB/oct", "12 dB/oct", "18 db/oct", "24 dB/oct"]
  in  "High Value (K)":dbl=300.0
  in  "Low Value (K)":dbl=2.0
  in  "loop #":i32=1
  # "Mesurement 1T"
  # "Mesurement 1F"
  # "Lock-in 1 Setting"
  # "Lock-in 2 Setting"
  # "Statue"
  # "Channel 1A"
  # "Channel 2A"
  # "Current Measurement"
  # "Channel 2B"
  # "Channel 1B"
  # "Mesurement 2T"
  # "Mesurement 2F"
  # "Sweep F Mesurement 1"
  # "Temprature and Field Setting"
  # "Sweep T Mesurement 1"
  # "Sweep F"
  # "Sweep T"
  # "Sweep T Mesurement 2"
  # "Sweep F Mesurement 2"
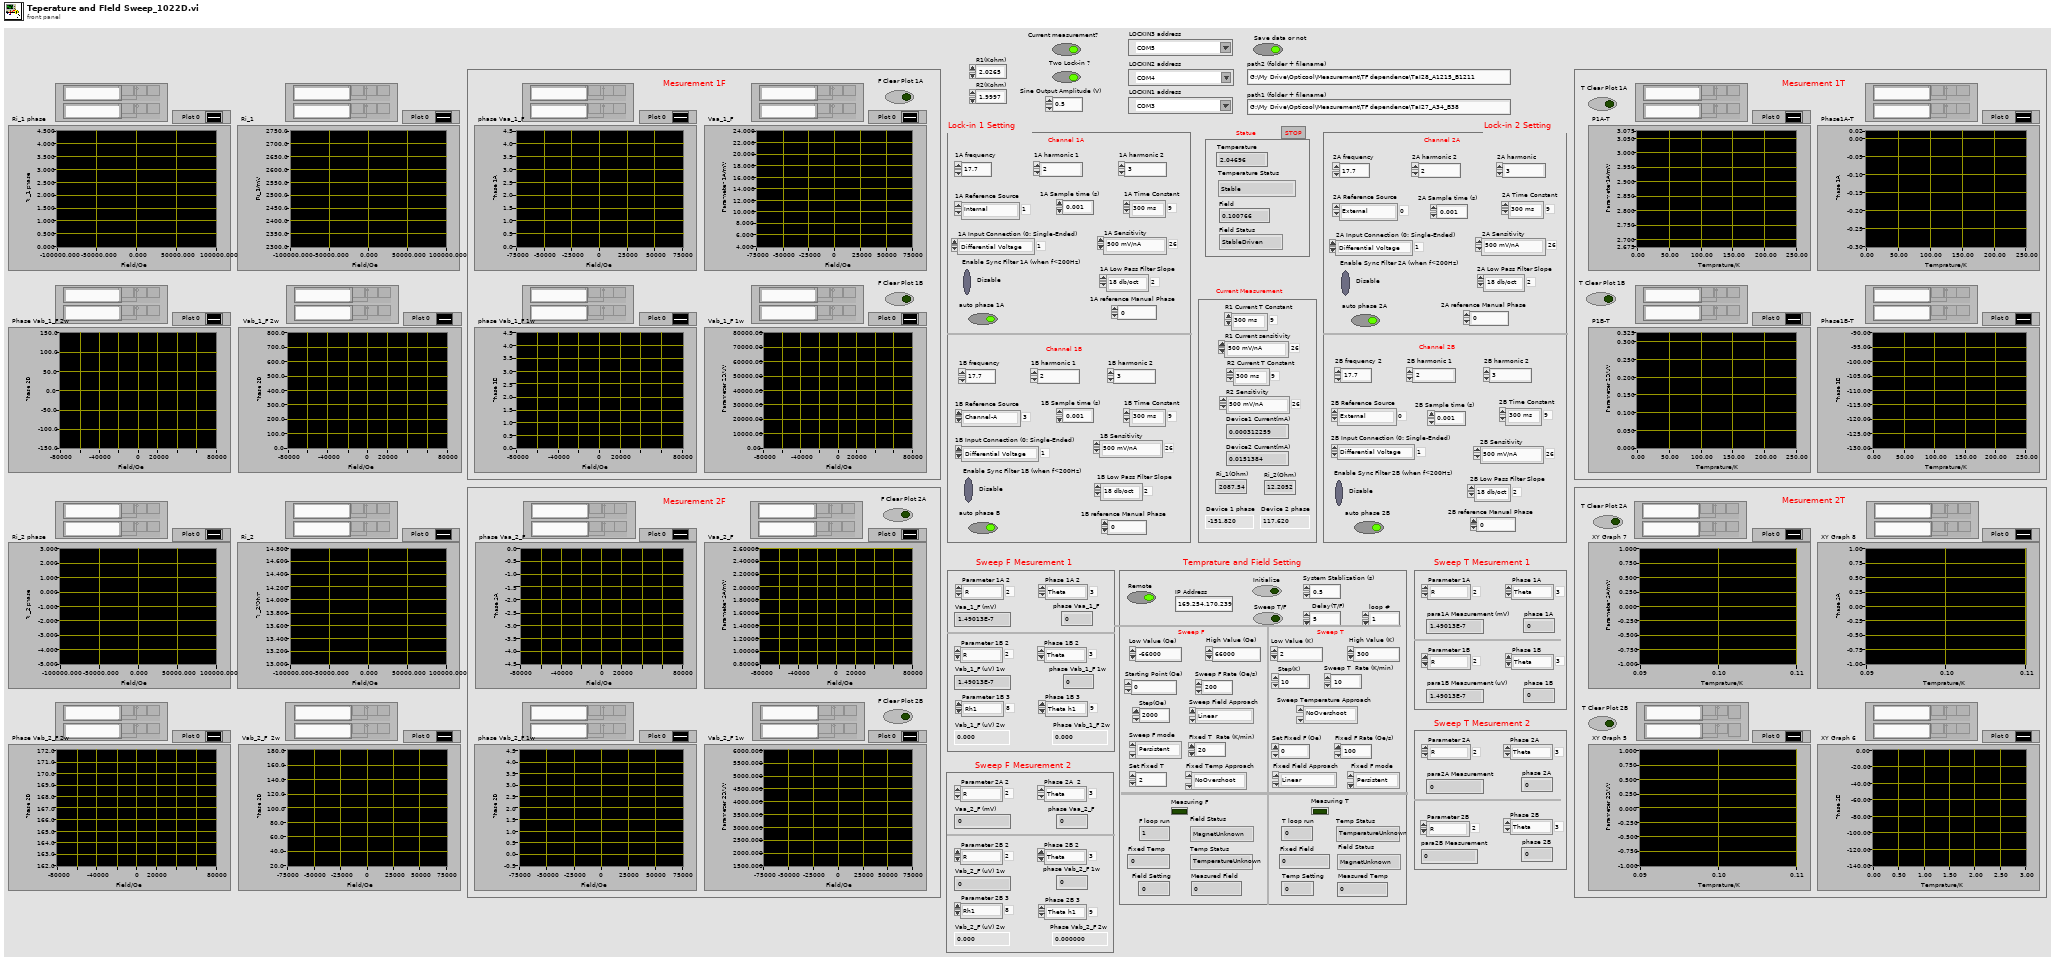
[diagram p1: front panel]
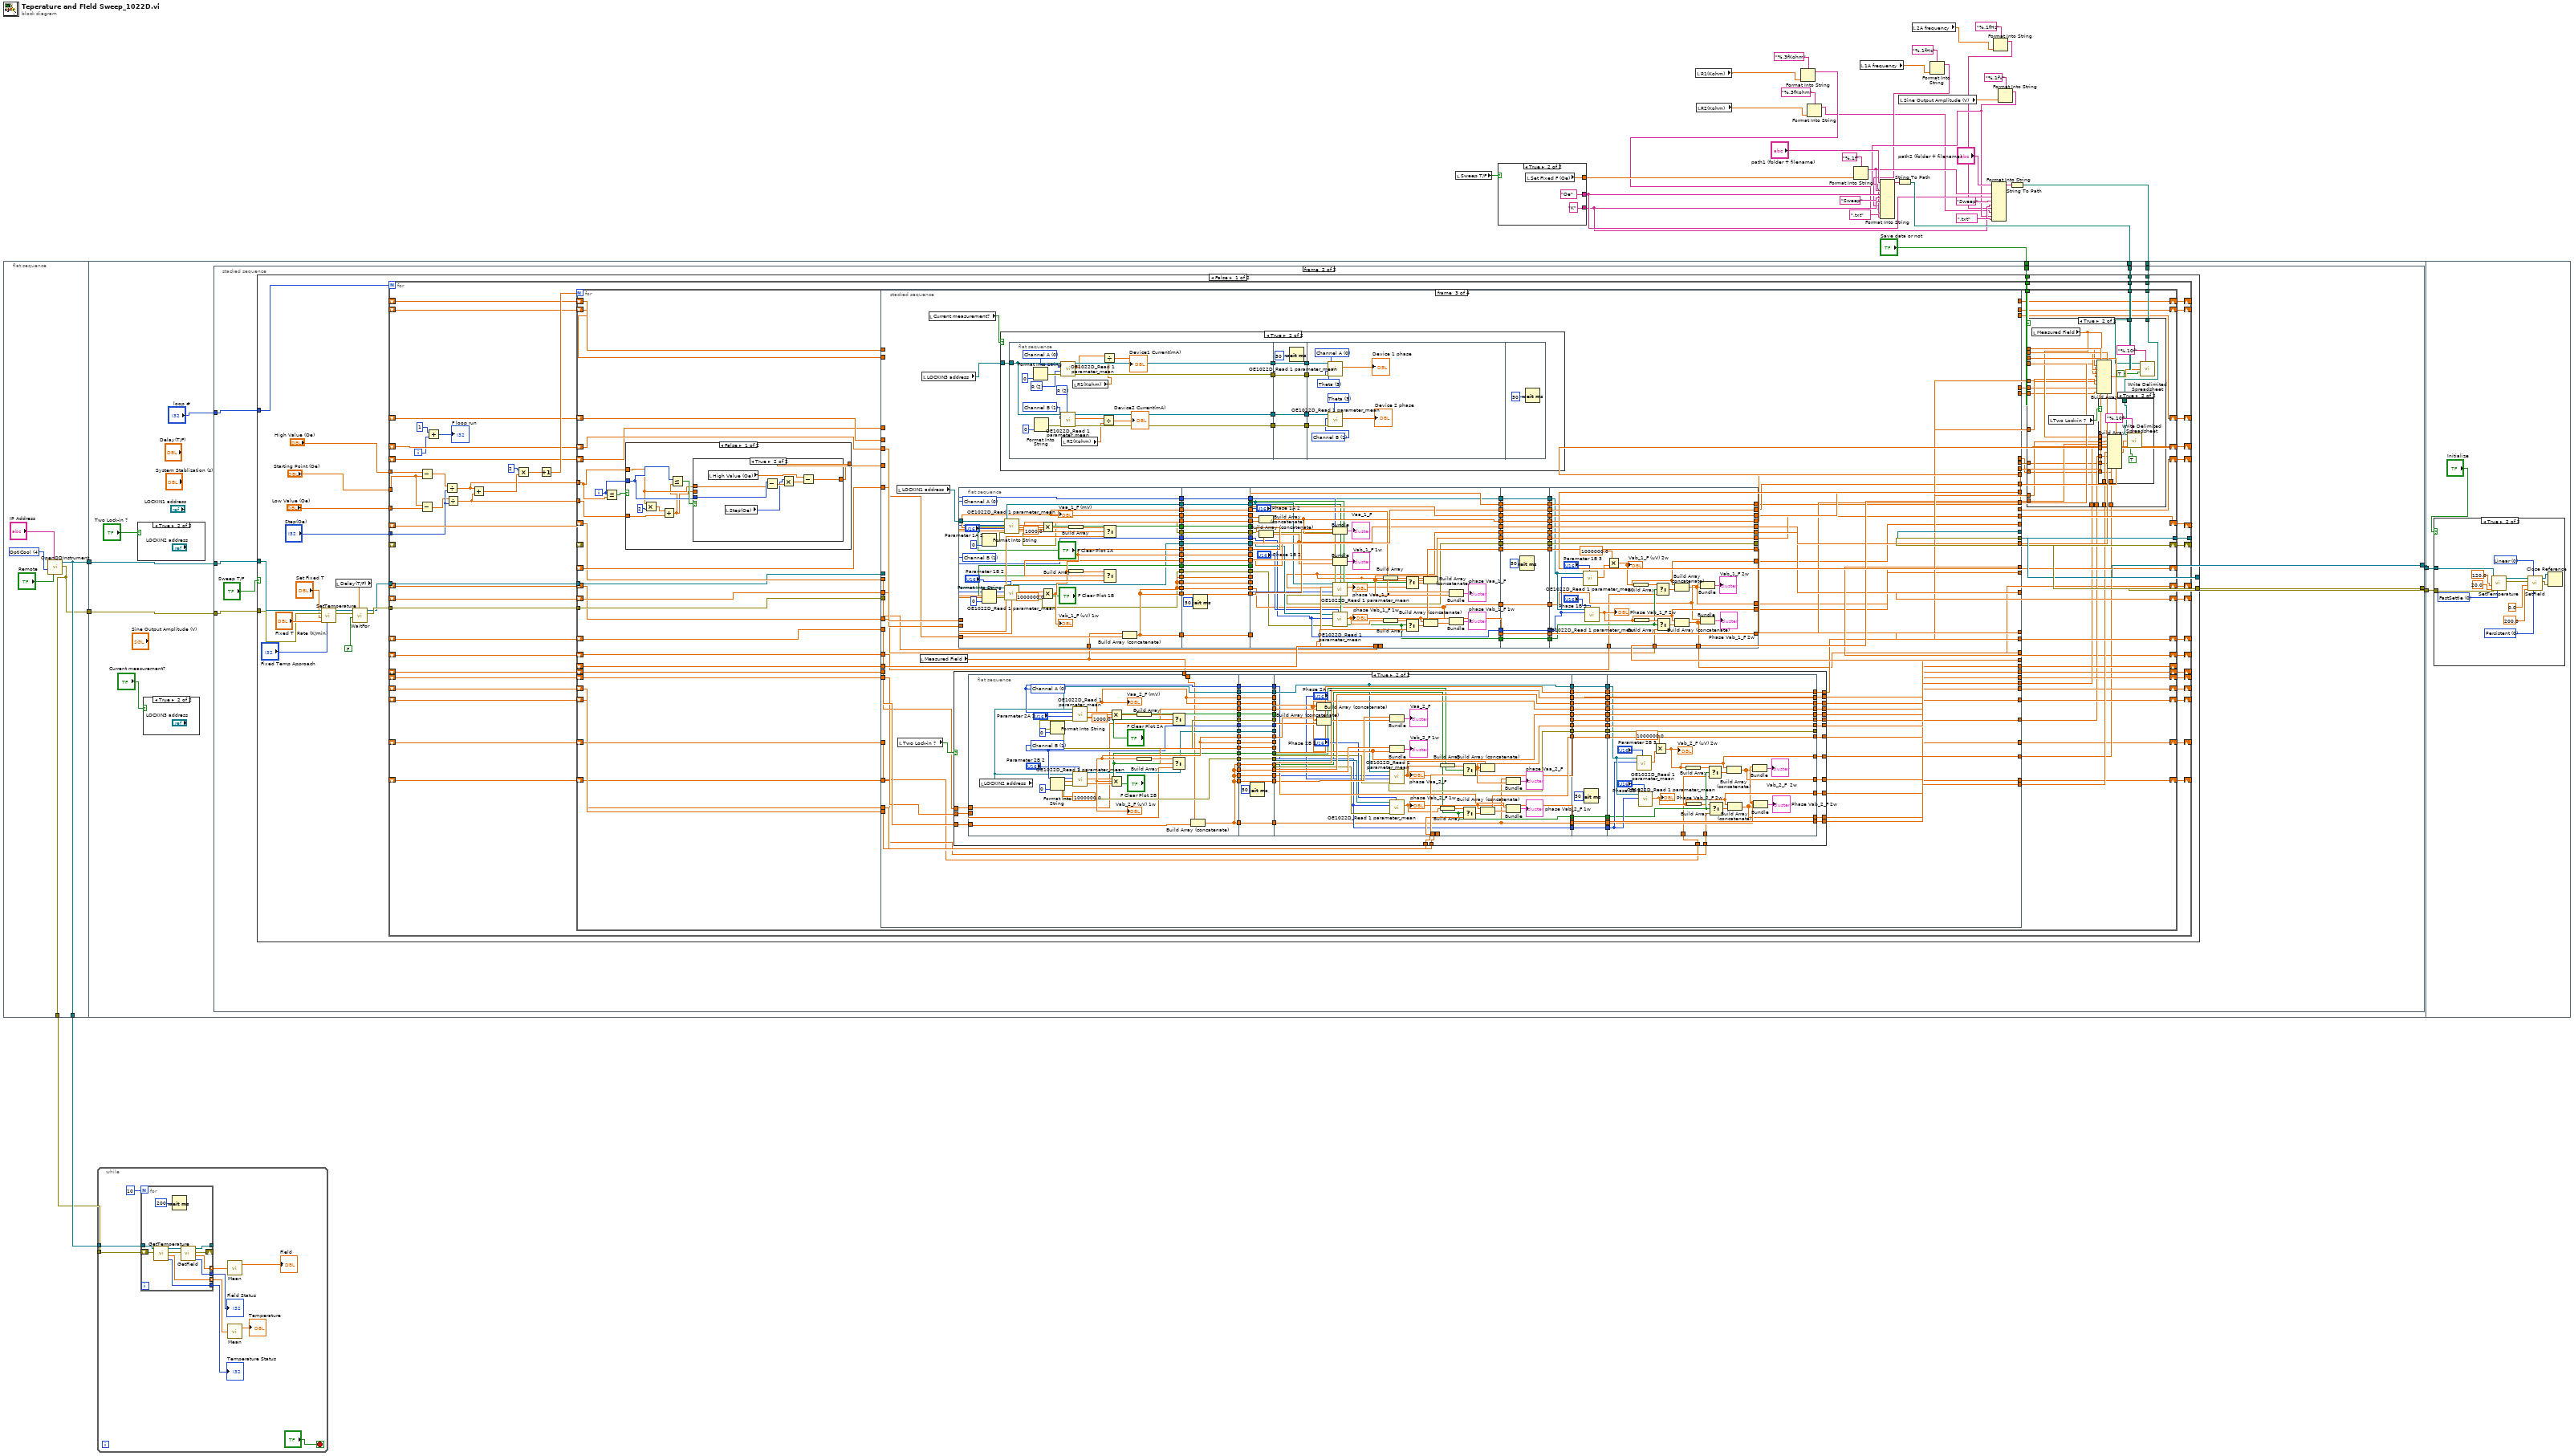
[diagram p0: block diagram]
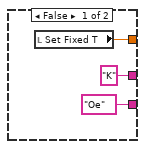
[diagram p2: hidden frame]
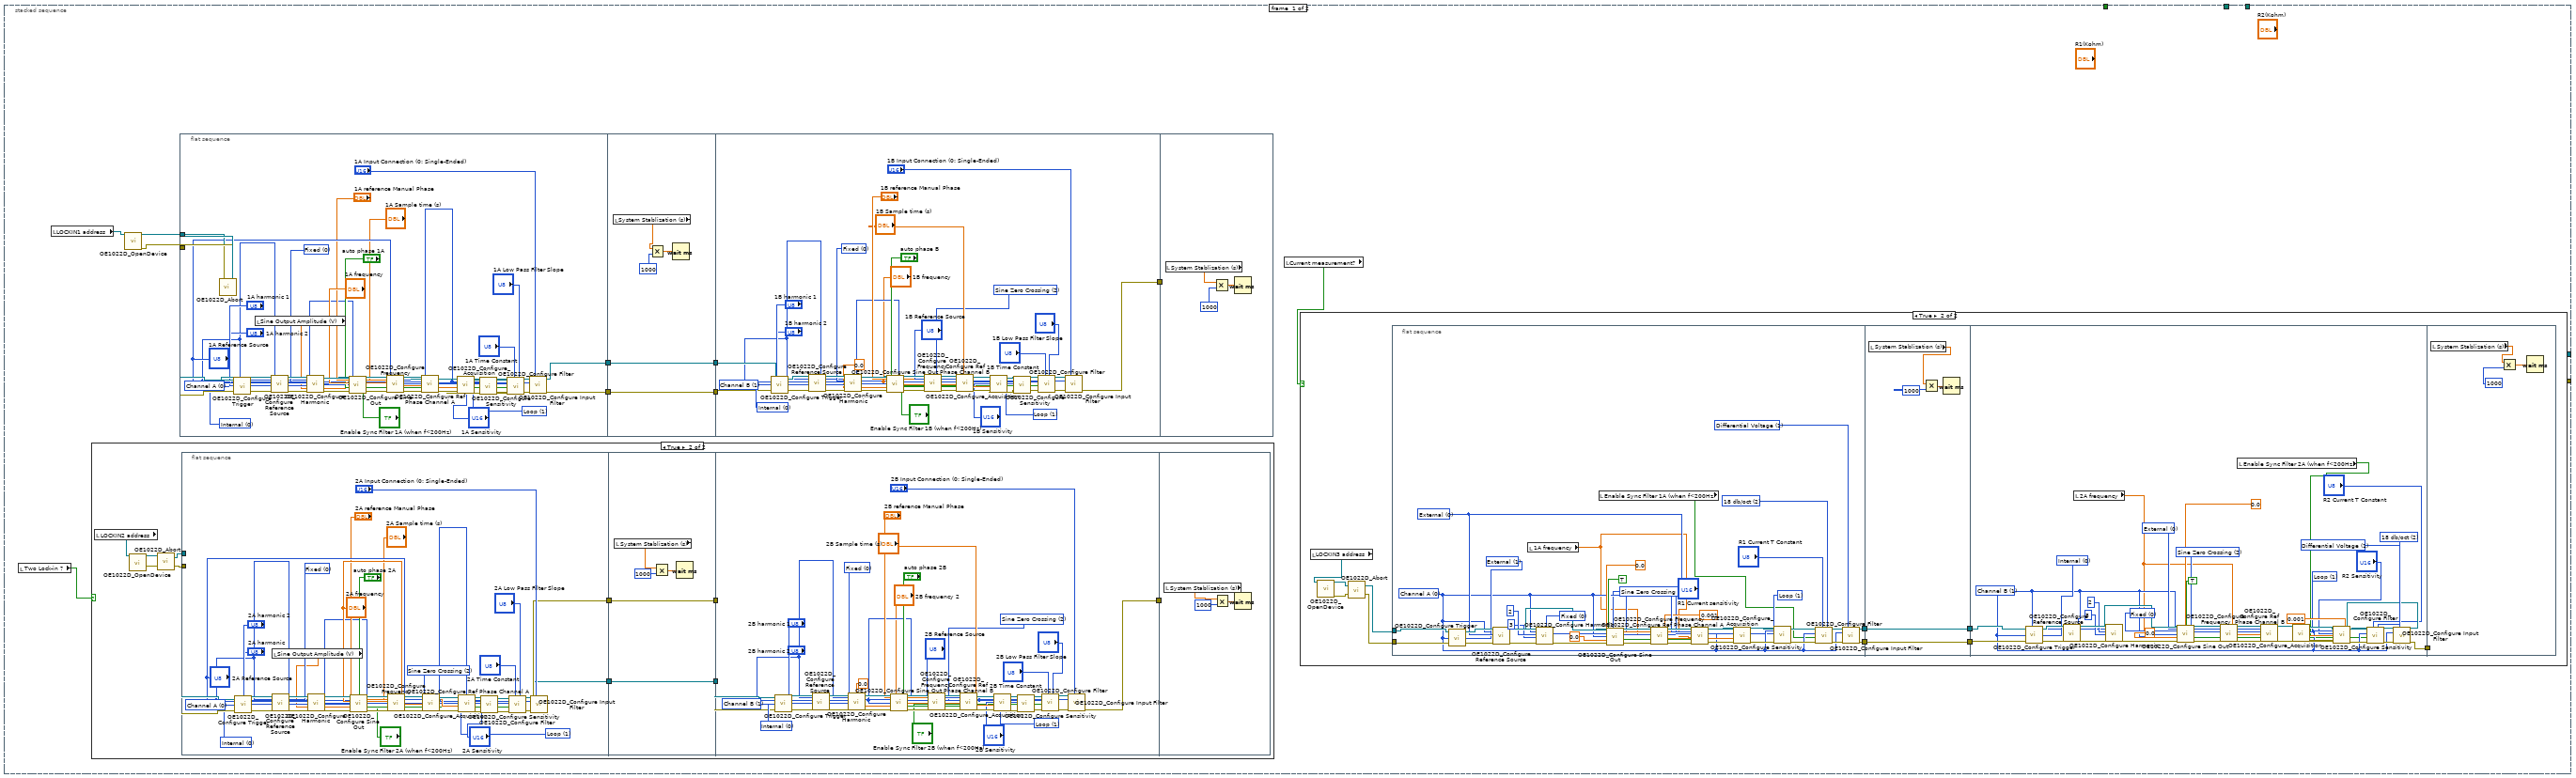
[diagram p5: hidden frame]
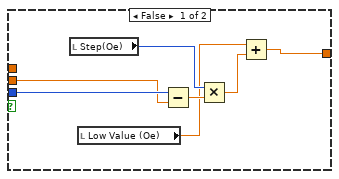
[diagram p10: hidden frame]
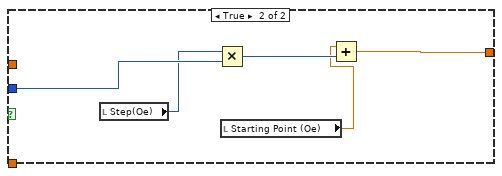
[diagram p11: hidden frame]
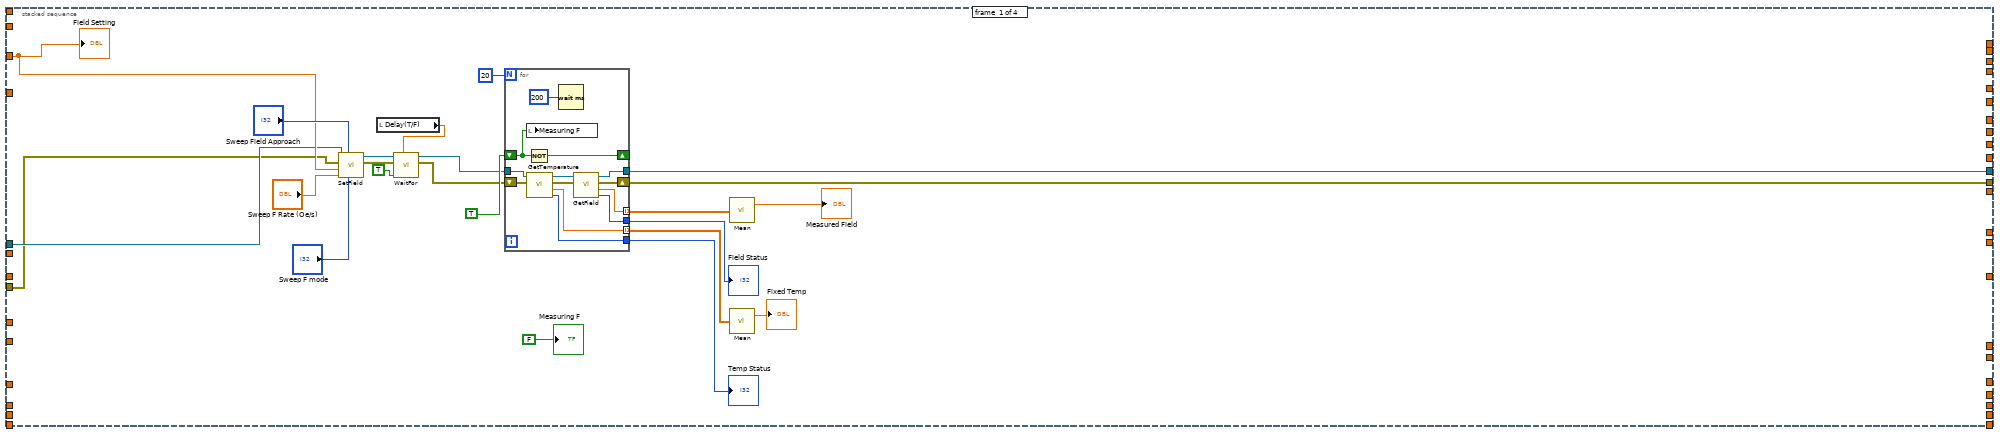
[diagram p12: hidden frame]
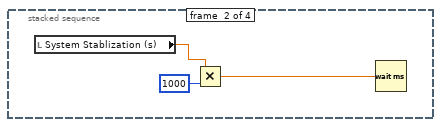
[diagram p13: hidden frame]
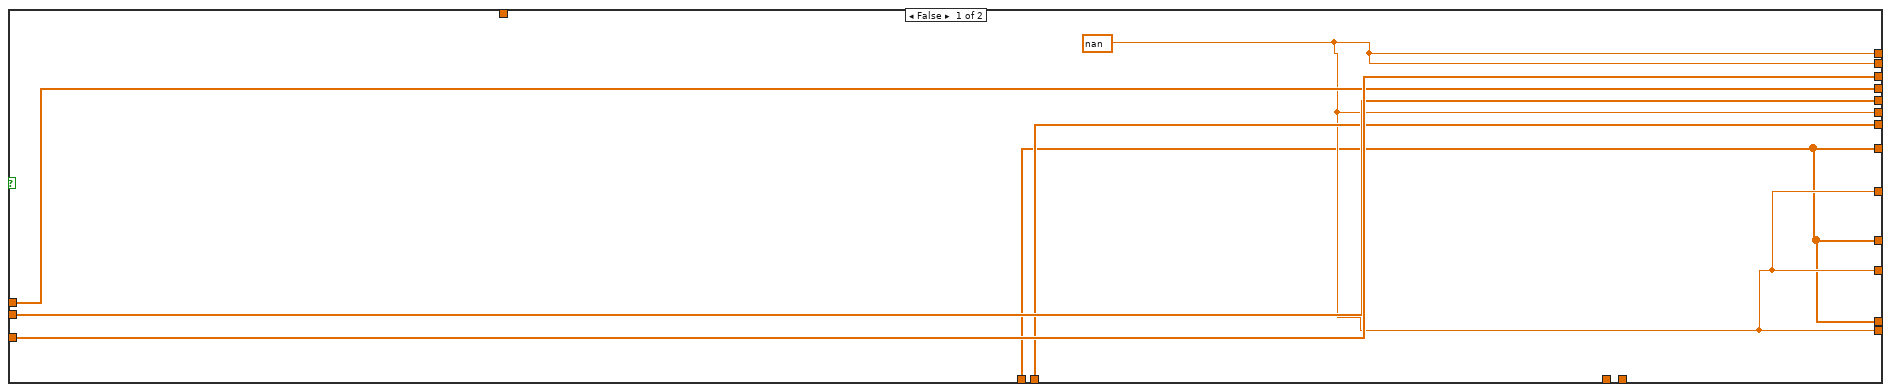
[diagram p15: hidden frame]
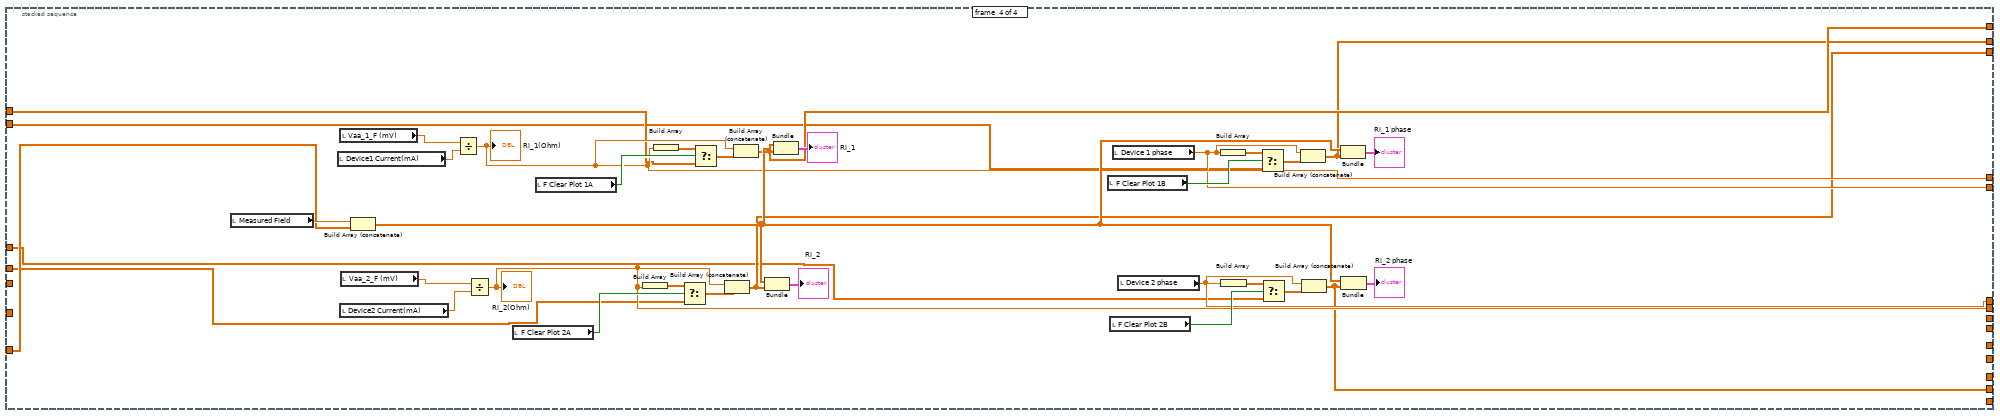
[diagram p16: hidden frame]
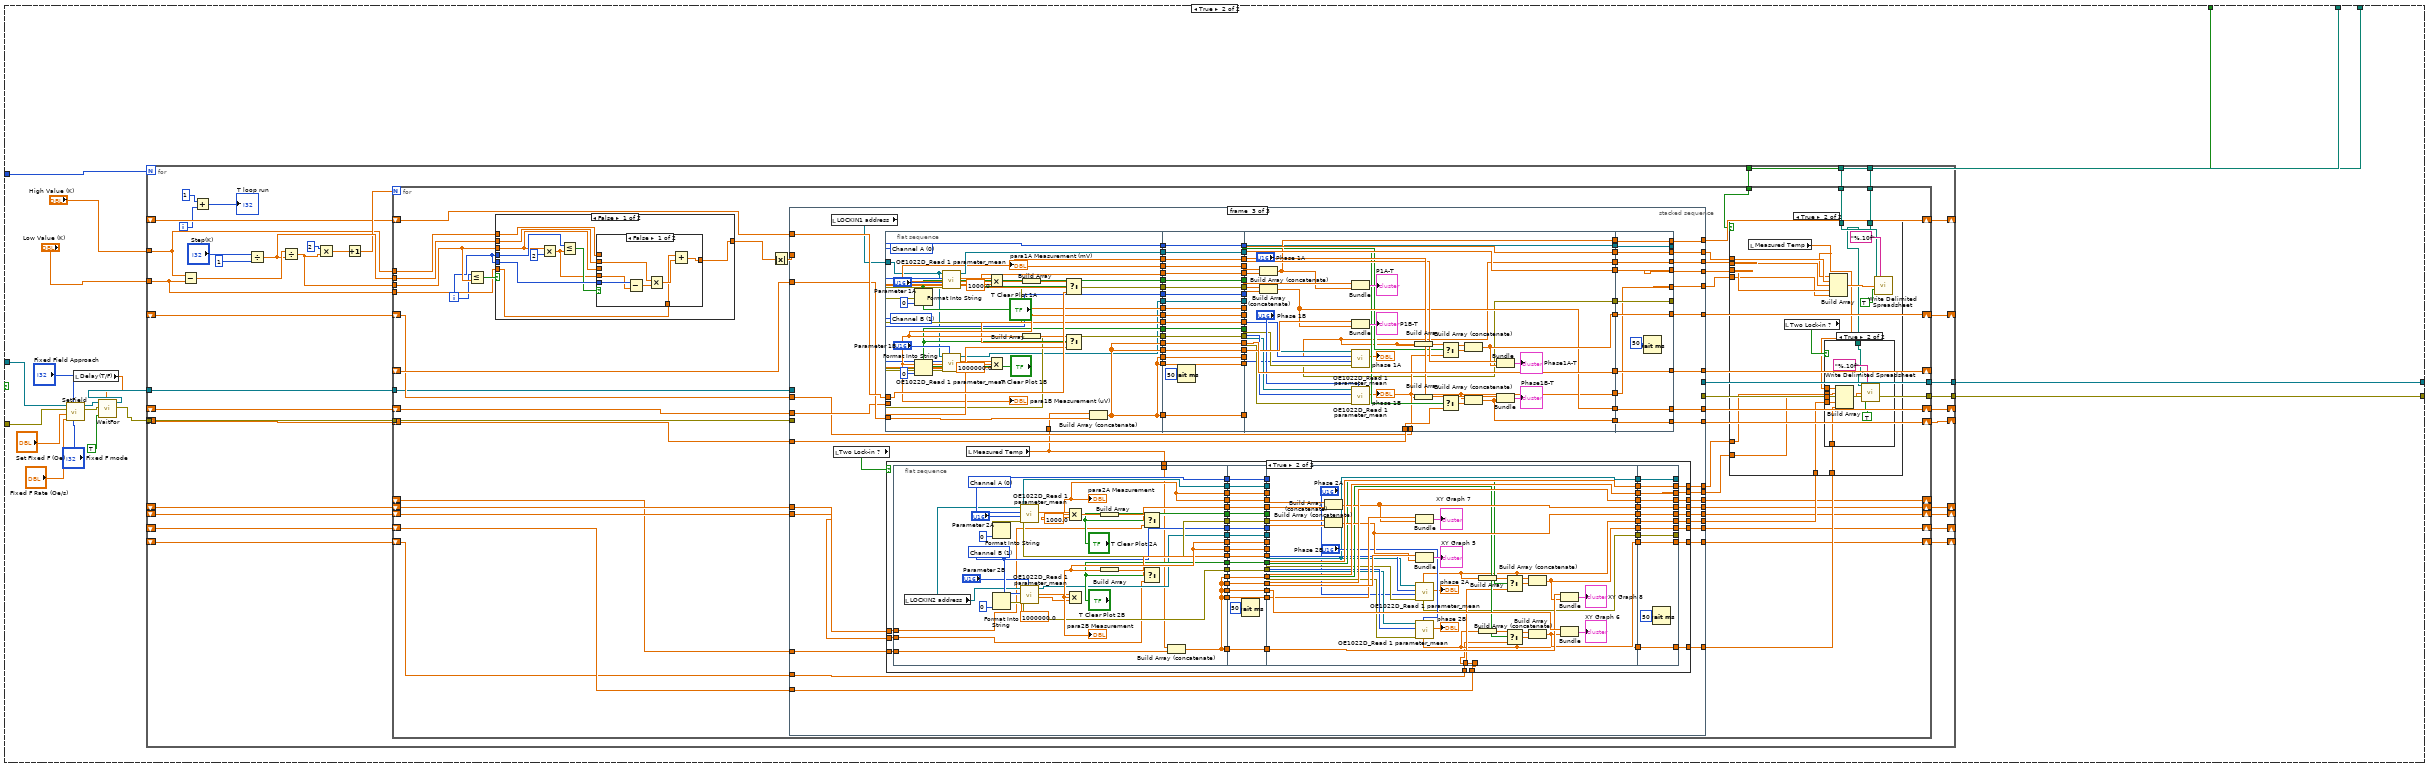
[diagram p17: hidden frame]
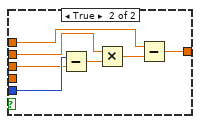
[diagram p20: hidden frame]
diagram:
  n1 = flat-sequence {
    tunnel: [w40] -> w38
    tunnel: [w39] -> w37
    tunnel: [w40] -> w34
    tunnel: [w39] -> w33
    tunnel: w38 -> [w52]
    tunnel: w37 -> [w51]
    tunnel: [w50] -> w36
    tunnel: [w49] -> w35
    tunnel: w26 -> [w48]
    tunnel: "Save data or not" -> [w47]
    tunnel: w19 -> [w45]
    tunnel: w36 -> [w1687]
    tunnel: w35 -> [w1686]
    frame #0 {
      w41 = 4 items=["PPMS", "VersaLab", "DynaCool", "SVSM", "OptiCool"] ("InstrumentType")
      n2 = call "OpenQDInstrument.vi"("Remote"="Remote", "IP Address"="IP Address", "InstrumentType"=w41) -> ("error out"=w39:errorcluster, "Instrument Ref"=w40:refnum<k24>)  [unwired: 5 in]
    }
    frame #1 {
      n3 = case shown="True" "Two Lock-in ?" {
        frame False {
        }
        frame True {
        }
      }
      n4 = case shown="True" "Current measurement?" {
        frame False {
        }
        frame True {
        }
      }
      n5 = stacked-sequence {
        tunnel: "loop #" -> [_ w354]
        tunnel: w52 -> [_ w352]
        tunnel: w51 -> [_ w351]
        tunnel: [_ w350] -> w50
        tunnel: [_ w349] -> w49
        tunnel: w48 -> [_ w348]
        tunnel: w47 -> [_ w347]
        tunnel: w45 -> [_ w346]
        frame #0 {
          n6 = local read "Two Lock-in ?"() -> (w55:bool)
          n7 = local read "LOCKIN1 address"() -> (w56:refnum<visa-resource-name>)
          n8 = case shown="True" w55 {
            frame False {
            }
            frame True {
              n9 = local read "LOCKIN2 address"() -> (w163:refnum<visa-resource-name>)
              n10 = call "OE1022D_OpenDevice.vi"("VISA resource name"=w163) -> ("VISA资源名称输出"=w166:refnum<visa-resource-name>, "错误输出"=w167:errorcluster)  [unwired: 17 in]
              n11 = call "OE1022D_Abort.vi"("error in (no error)"=w167, "VISA resource name"=w166) -> ("error out"=w164:errorcluster, "VISA resource name out"=w165:refnum<visa-resource-name>)
              n12 = flat-sequence {
                tunnel: w165 -> [w212]
                tunnel: [w201] -> w172
                tunnel: w164 -> [w211]
                tunnel: [w189] -> w171
                tunnel: w172 -> [w217]
                tunnel: [w217] -> w170
                tunnel: w171 -> [w216]
                tunnel: [w216] -> w169
                tunnel: w170 -> [w239]
                tunnel: [w238] -> w168
                tunnel: w169 -> [w237]
                tunnel: w168 -> [_]
                frame #0 {
                  w174 = u8 2 items=["TTL Pos", "TTL Neg", "Sine Zero Crossing"] ("External Ref Trigger")
                  w175 = u8 1 items=["Single", "Loop"] ("Sample Mode (Single/Loop)")
                  w188 = u8 0 items=["Fixed", "Linear", "Log"] ("SineOut Mode")
                  w190 = u16 0 items=["Internal", "External"] ("Trigger Source (0: Internal)")
                  w179 = u8 0 items=["Channel A", "Channel B"] ("OE1022D A/B")
                  n13 = call "OE1022D_Configure Trigger.vi"("Trigger Source (0: Internal)"=w190, "error in (no error)   2"=w211, "OE1022D A/B"=w179, "VISA resource name   2"=w212) -> ("error out   2"=w206:errorcluster, "VISA resource name out   2"=w207:refnum<visa-resource-name>)
                  n14 = local read "Sine Output Amplitude (V)"() -> (w173:sgl)
                  n15 = call "OE1022D_Configure Reference Source.vi"("VISA resource name"=w207, "OE1022D A/B"=w179, "Reference Source"="2A Reference Source", "error in (no error)"=w206) -> ("VISA resource name out"=w205:refnum<visa-resource-name>, "error out"=w203:errorcluster)  [unwired: 14 in]
                  n16 = call "OE1022D_Configure Harmonic.vi"("VISA resource name"=w205, "OE1022D A/B"=w179, "Harmonic 1"="2A harmonic 2", "Harmonic 2"="2A harmonic", "error in (no error)"=w203) -> ("VISA resource name out"=w204:refnum<visa-resource-name>, "error out"=w202:errorcluster)  [unwired: 13 in]
                  n17 = call "OE1022D_Configure Sine Out.vi"("VISA resource name"=w204, "SineOut Mode"=w188, "OE1022D A/B"=w179, "Sine Output Amplitude (V)"=w173, "error in (no error)"=w202) -> ("VISA resource name out"=w209:refnum<visa-resource-name>, "error out"=w208:errorcluster)  [unwired: 9 in]
                  n18 = call "OE1022D_Configure Frequency.vi"("VISA resource name"=w209, "OE1022D A/B"=w179, "Internal Frequency(Hz)"="2A frequency", "error in (no error)"=w208) -> ("VISA resource name out"=w200:refnum<visa-resource-name>, "error out"=w197:errorcluster)  [unwired: 14 in]
                  n19 = call "OE1022D_Configure Ref Phase Channel A.vi"("VISA resource name"=w200, "Reference Source"="2A Reference Source", "External Ref Trigger"=w174, "Internal Frequency(Hz)"="2A frequency", "Auto Phase (T: Enabled)"="auto phase 2A", "error in (no error)"=w197, "Manual Phase  (degree)"="2A reference Manual Phase") -> ("VISA resource name out"=w199:refnum<visa-resource-name>, "error out"=w198:errorcluster)  [unwired: 11 in]
                  n20 = call "OE1022D_Configure_Acquisition.vi"("VISA resource name"=w199, "OE1022D A/B"=w179, "Sample time (s)"="2A Sample time (s)", "error in (no error)"=w198, "Sample Mode (Single/Loop)"=w175) -> ("VISA resource name out"=w182:refnum<visa-resource-name>, "error out"=w181:errorcluster)  [unwired: 3 in]
                  n21 = call "OE1022D_Configure Sensitivity.vi"("VISA resource name"=w182, "OE1022D A/B"=w179, "Sensitivity"="2A Sensitivity", "error in (no error)"=w181) -> ("VISA resource name out"=w186:refnum<visa-resource-name>, "error out"=w185:errorcluster)  [unwired: 14 in]
                  n22 = call "OE1022D_Configure Filter.vi"("Low Pass Filter Slope (1: 12dB/oct)"="2A Low Pass Filter Slope", "Time Constant (8: 100ms)"="2A Time Constant", "error in (no error)"=w185, "Enable Sync Filter (F: Disable)"="Enable Sync Filter 2A (when f<200Hz)", "OE1022D A/B"=w179, "VISA resource name"=w186) -> ("error out"=w183:errorcluster, "VISA resource name out"=w184:refnum<visa-resource-name>)  [unwired: 4 in]
                  n23 = call "OE1022D_Configure Input Filter.vi"("VISA resource name"=w184, "Input Source"="2A Input Connection (0: Single-Ended)", "OE1022D A/B"=w179, "error in (no error)"=w183) -> ("VISA resource name out"=w189:refnum<visa-resource-name>, "error out"=w201:errorcluster)  [unwired: 10 in]
                }
                frame #1 {
                  n24 = local read "System Stablization (s)"() -> (w213:dbl)
                  n25 = Multiply(x=w213, y=1000) -> (x*y=w215:dbl)
                  n26 = Wait (ms)(milliseconds to wait=w215) -> ()  [unwired: 1 out]
                }
                frame #2 {
                  w219 = u8 1 items=["Single", "Loop"] ("Sample Mode (Single/Loop)")
                  w221 = u8 2 items=["TTL Pos", "TTL Neg", "Sine Zero Crossing"] ("External Ref Trigger")
                  w234 = u8 0 items=["Fixed", "Linear", "Log"] ("SineOut Mode")
                  w240 = u16 0 items=["Internal", "External"] ("Trigger Source (0: Internal)")
                  w226 = u8 1 items=["Channel A", "Channel B"] ("OE1022D A/B")
                  n27 = call "OE1022D_Configure Trigger.vi"("Trigger Source (0: Internal)"=w240, "error in (no error)   2"=w239, "OE1022D A/B"=w226, "VISA resource name   2"=w237) -> ("error out   2"=w252:errorcluster, "VISA resource name out   2"=w253:refnum<visa-resource-name>)
                  n28 = call "OE1022D_Configure Reference Source.vi"("VISA resource name"=w253, "OE1022D A/B"=w226, "error in (no error)"=w252) -> ("VISA resource name out"=w251:refnum<visa-resource-name>, "error out"=w249:errorcluster)  [unwired: 15 in]
                  n29 = call "OE1022D_Configure Harmonic.vi"("VISA resource name"=w251, "OE1022D A/B"=w226, "Harmonic 1"="2B harmonic 1", "Harmonic 2"="2B harmonic 2", "error in (no error)"=w249) -> ("VISA resource name out"=w250:refnum<visa-resource-name>, "error out"=w248:errorcluster)  [unwired: 13 in]
                  n30 = call "OE1022D_Configure Sine Out.vi"("VISA resource name"=w250, "SineOut Mode"=w234, "OE1022D A/B"=w226, "Sine Output Amplitude (V)"=sgl 0.0, "error in (no error)"=w248) -> ("VISA resource name out"=w255:refnum<visa-resource-name>, "error out"=w254:errorcluster)  [unwired: 9 in]
                  n31 = call "OE1022D_Configure Frequency.vi"("VISA resource name"=w255, "OE1022D A/B"=w226, "Internal Frequency(Hz)"="2B frequency 2", "error in (no error)"=w254) -> ("VISA resource name out"=w247:refnum<visa-resource-name>, "error out"=w244:errorcluster)  [unwired: 14 in]
                  n32 = call "OE1022D_Configure Ref Phase Channel B.vi"("VISA resource name"=w247, "Reference Source"="2B Reference Source", "External Ref Trigger"=w221, "Internal Frequency(Hz)"="2B frequency 2", "Auto Phase (T: Enabled)"="auto phase 2B", "error in (no error)"=w244, "Manual Phase  (degree)"="2B reference Manual Phase") -> ("VISA resource name out"=w246:refnum<visa-resource-name>, "error out"=w245:errorcluster)  [unwired: 11 in]
                  n33 = call "OE1022D_Configure_Acquisition.vi"("VISA resource name"=w246, "OE1022D A/B"=w226, "Sample time (s)"="2B Sample time (s)", "error in (no error)"=w245, "Sample Mode (Single/Loop)"=w219) -> ("VISA resource name out"=w227:refnum<visa-resource-name>, "error out"=w228:errorcluster)  [unwired: 3 in]
                  n34 = call "OE1022D_Configure Sensitivity.vi"("VISA resource name"=w227, "OE1022D A/B"=w226, "Sensitivity"="2B Sensitivity", "error in (no error)"=w228) -> ("VISA resource name out"=w231:refnum<visa-resource-name>, "error out"=w230:errorcluster)  [unwired: 14 in]
                  n35 = call "OE1022D_Configure Filter.vi"("Low Pass Filter Slope (1: 12dB/oct)"="2B Low Pass Filter Slope", "Time Constant (8: 100ms)"="2B Time Constant", "error in (no error)"=w230, "Enable Sync Filter (F: Disable)"="Enable Sync Filter 2B (when f<200Hz)", "OE1022D A/B"=w226, "VISA resource name"=w231) -> ("error out"=w229:errorcluster, "VISA resource name out"=w218:refnum<visa-resource-name>)  [unwired: 4 in]
                  n36 = call "OE1022D_Configure Input Filter.vi"("VISA resource name"=w218, "Input Source"="2B Input Connection (0: Single-Ended)", "OE1022D A/B"=w226, "error in (no error)"=w229) -> ("error out"=w238:errorcluster)  [unwired: 10 in, 1 out]
                }
                frame #3 {
                  n37 = local read "System Stablization (s)"() -> (w257:dbl)
                  n38 = Multiply(x=w257, y=1000) -> (x*y=w259:dbl)
                  n39 = Wait (ms)(milliseconds to wait=w259) -> ()  [unwired: 1 out]
                }
              }
            }
          }
          n40 = call "OE1022D_OpenDevice.vi"("VISA resource name"=w56) -> ("VISA资源名称输出"=w57:refnum<visa-resource-name>, "错误输出"=w58:errorcluster)  [unwired: 17 in]
          n41 = flat-sequence {
            tunnel: w64 -> [w298]
            tunnel: [w287] -> w62
            tunnel: w63 -> [w297]
            tunnel: [w275] -> w60
            tunnel: w62 -> [w303]
            tunnel: [w303] -> w61
            tunnel: w60 -> [w302]
            tunnel: [w302] -> w59
            tunnel: w61 -> [w325]
            tunnel: [w324] -> w65
            tunnel: w59 -> [w323]
            tunnel: w65 -> [_]
            frame #0 {
              w261 = u8 1 items=["Single", "Loop"] ("Sample Mode (Single/Loop)")
              w274 = u8 0 items=["Fixed", "Linear", "Log"] ("SineOut Mode")
              w276 = u16 0 items=["Internal", "External"] ("Trigger Source (0: Internal)")
              w265 = u8 0 items=["Channel A", "Channel B"] ("OE1022D A/B")
              n42 = call "OE1022D_Configure Trigger.vi"("Trigger Source (0: Internal)"=w276, "error in (no error)   2"=w297, "OE1022D A/B"=w265, "VISA resource name   2"=w298) -> ("error out   2"=w292:errorcluster, "VISA resource name out   2"=w293:refnum<visa-resource-name>)
              n43 = local read "Sine Output Amplitude (V)"() -> (w260:sgl)
              n44 = call "OE1022D_Configure Reference Source.vi"("VISA resource name"=w293, "OE1022D A/B"=w265, "Reference Source"="1A Reference Source", "error in (no error)"=w292) -> ("VISA resource name out"=w291:refnum<visa-resource-name>, "error out"=w289:errorcluster)  [unwired: 14 in]
              n45 = call "OE1022D_Configure Harmonic.vi"("VISA resource name"=w291, "OE1022D A/B"=w265, "Harmonic 1"="1A harmonic 1", "Harmonic 2"="1A harmonic 2", "error in (no error)"=w289) -> ("VISA resource name out"=w290:refnum<visa-resource-name>, "error out"=w288:errorcluster)  [unwired: 13 in]
              n46 = call "OE1022D_Configure Sine Out.vi"("VISA resource name"=w290, "SineOut Mode"=w274, "OE1022D A/B"=w265, "Sine Output Amplitude (V)"=w260, "error in (no error)"=w288) -> ("VISA resource name out"=w295:refnum<visa-resource-name>, "error out"=w294:errorcluster)  [unwired: 9 in]
              n47 = call "OE1022D_Configure Frequency.vi"("VISA resource name"=w295, "OE1022D A/B"=w265, "Internal Frequency(Hz)"="1A frequency", "error in (no error)"=w294) -> ("VISA resource name out"=w286:refnum<visa-resource-name>, "error out"=w283:errorcluster)  [unwired: 14 in]
              n48 = call "OE1022D_Configure Ref Phase Channel A.vi"("VISA resource name"=w286, "Reference Source"="1A Reference Source", "Internal Frequency(Hz)"="1A frequency", "Auto Phase (T: Enabled)"="auto phase 1A", "error in (no error)"=w283, "Manual Phase  (degree)"="1A reference Manual Phase") -> ("VISA resource name out"=w285:refnum<visa-resource-name>, "error out"=w284:errorcluster)  [unwired: 12 in]
              n49 = call "OE1022D_Configure_Acquisition.vi"("VISA resource name"=w285, "OE1022D A/B"=w265, "Sample time (s)"="1A Sample time (s)", "error in (no error)"=w284, "Sample Mode (Single/Loop)"=w261) -> ("VISA resource name out"=w268:refnum<visa-resource-name>, "error out"=w267:errorcluster)  [unwired: 3 in]
              n50 = call "OE1022D_Configure Sensitivity.vi"("VISA resource name"=w268, "OE1022D A/B"=w265, "Sensitivity"="1A Sensitivity", "error in (no error)"=w267) -> ("VISA resource name out"=w272:refnum<visa-resource-name>, "error out"=w271:errorcluster)  [unwired: 14 in]
              n51 = call "OE1022D_Configure Filter.vi"("Low Pass Filter Slope (1: 12dB/oct)"="1A Low Pass Filter Slope", "Time Constant (8: 100ms)"="1A Time Constant", "error in (no error)"=w271, "Enable Sync Filter (F: Disable)"="Enable Sync Filter 1A (when f<200Hz)", "OE1022D A/B"=w265, "VISA resource name"=w272) -> ("error out"=w269:errorcluster, "VISA resource name out"=w270:refnum<visa-resource-name>)  [unwired: 4 in]
              n52 = call "OE1022D_Configure Input Filter.vi"("VISA resource name"=w270, "Input Source"="1A Input Connection (0: Single-Ended)", "OE1022D A/B"=w265, "error in (no error)"=w269) -> ("VISA resource name out"=w275:refnum<visa-resource-name>, "error out"=w287:errorcluster)  [unwired: 10 in]
            }
            frame #1 {
              n53 = local read "System Stablization (s)"() -> (w299:dbl)
              n54 = Multiply(x=w299, y=1000) -> (x*y=w301:dbl)
              n55 = Wait (ms)(milliseconds to wait=w301) -> ()  [unwired: 1 out]
            }
            frame #2 {
              w305 = u8 1 items=["Single", "Loop"] ("Sample Mode (Single/Loop)")
              w307 = u8 2 items=["TTL Pos", "TTL Neg", "Sine Zero Crossing"] ("External Ref Trigger")
              w320 = u8 0 items=["Fixed", "Linear", "Log"] ("SineOut Mode")
              w326 = u16 0 items=["Internal", "External"] ("Trigger Source (0: Internal)")
              w312 = u8 1 items=["Channel A", "Channel B"] ("OE1022D A/B")
              n56 = call "OE1022D_Configure Trigger.vi"("Trigger Source (0: Internal)"=w326, "error in (no error)   2"=w325, "OE1022D A/B"=w312, "VISA resource name   2"=w323) -> ("error out   2"=w338:errorcluster, "VISA resource name out   2"=w339:refnum<visa-resource-name>)
              n57 = call "OE1022D_Configure Reference Source.vi"("VISA resource name"=w339, "OE1022D A/B"=w312, "error in (no error)"=w338) -> ("VISA resource name out"=w337:refnum<visa-resource-name>, "error out"=w335:errorcluster)  [unwired: 15 in]
              n58 = call "OE1022D_Configure Harmonic.vi"("VISA resource name"=w337, "OE1022D A/B"=w312, "Harmonic 1"="1B harmonic 1", "Harmonic 2"="1B harmonic 2", "error in (no error)"=w335) -> ("VISA resource name out"=w336:refnum<visa-resource-name>, "error out"=w334:errorcluster)  [unwired: 13 in]
              n59 = call "OE1022D_Configure Sine Out.vi"("VISA resource name"=w336, "SineOut Mode"=w320, "OE1022D A/B"=w312, "Sine Output Amplitude (V)"=sgl 0.0, "error in (no error)"=w334) -> ("VISA resource name out"=w341:refnum<visa-resource-name>, "error out"=w340:errorcluster)  [unwired: 9 in]
              n60 = call "OE1022D_Configure Frequency.vi"("VISA resource name"=w341, "OE1022D A/B"=w312, "Internal Frequency(Hz)"="1B frequency", "error in (no error)"=w340) -> ("VISA resource name out"=w333:refnum<visa-resource-name>, "error out"=w330:errorcluster)  [unwired: 14 in]
              n61 = call "OE1022D_Configure Ref Phase Channel B.vi"("VISA resource name"=w333, "Reference Source"="1B Reference Source", "External Ref Trigger"=w307, "Internal Frequency(Hz)"="1B frequency", "Auto Phase (T: Enabled)"="auto phase B", "error in (no error)"=w330, "Manual Phase  (degree)"="1B reference Manual Phase") -> ("VISA resource name out"=w332:refnum<visa-resource-name>, "error out"=w331:errorcluster)  [unwired: 11 in]
              n62 = call "OE1022D_Configure_Acquisition.vi"("VISA resource name"=w332, "OE1022D A/B"=w312, "Sample time (s)"="1B Sample time (s)", "error in (no error)"=w331, "Sample Mode (Single/Loop)"=w305) -> ("VISA resource name out"=w313:refnum<visa-resource-name>, "error out"=w314:errorcluster)  [unwired: 3 in]
              n63 = call "OE1022D_Configure Sensitivity.vi"("VISA resource name"=w313, "OE1022D A/B"=w312, "Sensitivity"="1B Sensitivity", "error in (no error)"=w314) -> ("VISA resource name out"=w317:refnum<visa-resource-name>, "error out"=w316:errorcluster)  [unwired: 14 in]
              n64 = call "OE1022D_Configure Filter.vi"("Low Pass Filter Slope (1: 12dB/oct)"="1B Low Pass Filter Slope", "Time Constant (8: 100ms)"="1B Time Constant", "error in (no error)"=w316, "Enable Sync Filter (F: Disable)"="Enable Sync Filter 1B (when f<200Hz)", "OE1022D A/B"=w312, "VISA resource name"=w317) -> ("error out"=w315:errorcluster, "VISA resource name out"=w304:refnum<visa-resource-name>)  [unwired: 4 in]
              n65 = call "OE1022D_Configure Input Filter.vi"("VISA resource name"=w304, "Input Source"="1B Input Connection (0: Single-Ended)", "OE1022D A/B"=w312, "error in (no error)"=w315) -> ("error out"=w324:errorcluster)  [unwired: 10 in, 1 out]
            }
            frame #3 {
              n66 = local read "System Stablization (s)"() -> (w343:dbl)
              n67 = Multiply(x=w343, y=1000) -> (x*y=w345:dbl)
              n68 = Wait (ms)(milliseconds to wait=w345) -> ()  [unwired: 1 out]
            }
          }
          n69 = call "OE1022D_Abort.vi"("error in (no error)"=w58, "VISA resource name"=w57) -> ("error out"=w63:errorcluster, "VISA resource name out"=w64:refnum<visa-resource-name>)
          n70 = local read "Current measurement?"() -> (w54:bool)
          n71 = case shown="True" w54 {
            frame False {
            }
            frame True {
              n72 = local read "LOCKIN3 address"() -> (w66:refnum<visa-resource-name>)
              n73 = call "OE1022D_OpenDevice.vi"("VISA resource name"=w66) -> ("VISA资源名称输出"=w69:refnum<visa-resource-name>, "错误输出"=w70:errorcluster)  [unwired: 17 in]
              n74 = call "OE1022D_Abort.vi"("error in (no error)"=w70, "VISA resource name"=w69) -> ("error out"=w67:errorcluster, "VISA resource name out"=w68:refnum<visa-resource-name>)
              n75 = flat-sequence {
                tunnel: w68 -> [w115]
                tunnel: [w103] -> w75
                tunnel: w67 -> [w114]
                tunnel: [w92] -> w74
                tunnel: w75 -> [w120]
                tunnel: [w120] -> w73
                tunnel: w74 -> [w119]
                tunnel: [w119] -> w72
                tunnel: w73 -> [w142]
                tunnel: [w141] -> w71
                tunnel: w72 -> [w140]
                tunnel: w71 -> [_]
                frame #0 {
                  w113 = u16 1 items=["Single-Ended Voltage", "Differential Voltage", "1 MOhm Current Gain", "100 MOhm Current Gain"] ("2A Input Connection (0: Single-Ended)  2")
                  w80 = u8 2 items=["6 dB/oct", "12 dB/oct", "18 db/oct", "24 dB/oct"] ("2A Low Pass Filter Slope 2")
                  w98 = u8 0 items=["External", "Internal", "Internal Sweep"] ("2A Reference Source 2")
                  w93 = u16 1 items=["Internal", "External"] ("Trigger Source (0: Internal)")
                  w78 = u8 2 items=["TTL Pos", "TTL Neg", "Sine Zero Crossing"] ("External Ref Trigger")
                  w79 = u8 1 items=["Single", "Loop"] ("Sample Mode (Single/Loop)")
                  w91 = u8 0 items=["Fixed", "Linear", "Log"] ("SineOut Mode")
                  w82 = u8 0 items=["Channel A", "Channel B"] ("OE1022D A/B")
                  n76 = call "OE1022D_Configure Trigger.vi"("Trigger Source (0: Internal)"=w93, "error in (no error)   2"=w114, "OE1022D A/B"=w82, "VISA resource name   2"=w115) -> ("error out   2"=w108:errorcluster, "VISA resource name out   2"=w109:refnum<visa-resource-name>)
                  n77 = call "OE1022D_Configure Reference Source.vi"("VISA resource name"=w109, "OE1022D A/B"=w82, "Reference Source"=w98, "error in (no error)"=w108) -> ("VISA resource name out"=w107:refnum<visa-resource-name>, "error out"=w105:errorcluster)  [unwired: 14 in]
                  n78 = local read "1A frequency"() -> (w77:dbl)
                  n79 = call "OE1022D_Configure Harmonic.vi"("VISA resource name"=w107, "OE1022D A/B"=w82, "Harmonic 1"=u8 2 ("2A harmonic 4"), "Harmonic 2"=u8 3 ("2A harmonic 3"), "error in (no error)"=w105) -> ("VISA resource name out"=w106:refnum<visa-resource-name>, "error out"=w104:errorcluster)  [unwired: 13 in]
                  n80 = local read "Enable Sync Filter 1A (when f<200Hz)"() -> (w76:bool)
                  n81 = call "OE1022D_Configure Sine Out.vi"("VISA resource name"=w106, "SineOut Mode"=w91, "OE1022D A/B"=w82, "Sine Output Amplitude (V)"=sgl 0.0, "error in (no error)"=w104) -> ("VISA resource name out"=w112:refnum<visa-resource-name>, "error out"=w111:errorcluster)  [unwired: 9 in]
                  n82 = call "OE1022D_Configure Frequency.vi"("VISA resource name"=w112, "OE1022D A/B"=w82, "Internal Frequency(Hz)"=w77, "error in (no error)"=w111) -> ("VISA resource name out"=w102:refnum<visa-resource-name>, "error out"=w99:errorcluster)  [unwired: 14 in]
                  n83 = call "OE1022D_Configure Ref Phase Channel A.vi"("VISA resource name"=w102, "Reference Source"=w98, "External Ref Trigger"=w78, "Internal Frequency(Hz)"=w77, "Auto Phase (T: Enabled)"=TRUE ("auto phase 2A 2"), "error in (no error)"=w99, "Manual Phase  (degree)"=0.0 ("2A reference Manual Phase 2")) -> ("VISA resource name out"=w101:refnum<visa-resource-name>, "error out"=w100:errorcluster)  [unwired: 11 in]
                  n84 = call "OE1022D_Configure_Acquisition.vi"("VISA resource name"=w101, "OE1022D A/B"=w82, "Sample time (s)"=0.001 ("2A Sample time (s) 2"), "error in (no error)"=w100, "Sample Mode (Single/Loop)"=w79) -> ("VISA resource name out"=w85:refnum<visa-resource-name>, "error out"=w84:errorcluster)  [unwired: 3 in]
                  n85 = call "OE1022D_Configure Sensitivity.vi"("VISA resource name"=w85, "OE1022D A/B"=w82, "Sensitivity"="R1 Current sensitivity", "error in (no error)"=w84) -> ("VISA resource name out"=w89:refnum<visa-resource-name>, "error out"=w88:errorcluster)  [unwired: 14 in]
                  n86 = call "OE1022D_Configure Filter.vi"("Low Pass Filter Slope (1: 12dB/oct)"=w80, "Time Constant (8: 100ms)"="R1 Current T Constant", "error in (no error)"=w88, "Enable Sync Filter (F: Disable)"=w76, "OE1022D A/B"=w82, "VISA resource name"=w89) -> ("error out"=w86:errorcluster, "VISA resource name out"=w87:refnum<visa-resource-name>)  [unwired: 4 in]
                  n87 = call "OE1022D_Configure Input Filter.vi"("VISA resource name"=w87, "Input Source"=w113, "OE1022D A/B"=w82, "error in (no error)"=w86) -> ("VISA resource name out"=w92:refnum<visa-resource-name>, "error out"=w103:errorcluster)  [unwired: 10 in]
                }
                frame #1 {
                  n88 = local read "System Stablization (s)"() -> (w116:dbl)
                  n89 = Multiply(x=w116, y=1000) -> (x*y=w118:dbl)
                  n90 = Wait (ms)(milliseconds to wait=w118) -> ()  [unwired: 1 out]
                }
                frame #2 {
                  w125 = u8 2 items=["6 dB/oct", "12 dB/oct", "18 db/oct", "24 dB/oct"] ("2B Low Pass Filter Slope 2")
                  w159 = u16 1 items=["Single-Ended Voltage", "Differential Voltage", "1 MOhm Current Gain", "100 MOhm Current Gain"] ("2B Input Connection (0: Single-Ended) 2")
                  w146 = u8 0 items=["External", "Internal", "Internal Sweep", "Channel-A"] ("2B Reference Source 2")
                  w124 = u8 1 items=["Single", "Loop"] ("Sample Mode (Single/Loop)")
                  w126 = u8 2 items=["TTL Pos", "TTL Neg", "Sine Zero Crossing"] ("External Ref Trigger")
                  w137 = u8 0 items=["Fixed", "Linear", "Log"] ("SineOut Mode")
                  w143 = u16 0 items=["Internal", "External"] ("Trigger Source (0: Internal)")
                  w129 = u8 1 items=["Channel A", "Channel B"] ("OE1022D A/B")
                  n91 = call "OE1022D_Configure Trigger.vi"("Trigger Source (0: Internal)"=w143, "error in (no error)   2"=w142, "OE1022D A/B"=w129, "VISA resource name   2"=w140) -> ("error out   2"=w155:errorcluster, "VISA resource name out   2"=w156:refnum<visa-resource-name>)
                  n92 = call "OE1022D_Configure Reference Source.vi"("VISA resource name"=w156, "OE1022D A/B"=w129, "error in (no error)"=w155) -> ("VISA resource name out"=w154:refnum<visa-resource-name>, "error out"=w152:errorcluster)  [unwired: 15 in]
                  n93 = local read "2A frequency"() -> (w122:dbl)
                  n94 = call "OE1022D_Configure Harmonic.vi"("VISA resource name"=w154, "OE1022D A/B"=w129, "Harmonic 1"=u8 2 ("2B harmonic 4"), "Harmonic 2"=u8 3 ("2B harmonic 3"), "error in (no error)"=w152) -> ("VISA resource name out"=w153:refnum<visa-resource-name>, "error out"=w151:errorcluster)  [unwired: 13 in]
                  n95 = call "OE1022D_Configure Sine Out.vi"("VISA resource name"=w153, "SineOut Mode"=w137, "OE1022D A/B"=w129, "Sine Output Amplitude (V)"=sgl 0.0, "error in (no error)"=w151) -> ("VISA resource name out"=w158:refnum<visa-resource-name>, "error out"=w157:errorcluster)  [unwired: 9 in]
                  n96 = call "OE1022D_Configure Frequency.vi"("VISA resource name"=w158, "OE1022D A/B"=w129, "Internal Frequency(Hz)"=w122, "error in (no error)"=w157) -> ("VISA resource name out"=w150:refnum<visa-resource-name>, "error out"=w147:errorcluster)  [unwired: 14 in]
                  n97 = local read "Enable Sync Filter 2A (when f<200Hz)"() -> (w121:bool)
                  n98 = call "OE1022D_Configure Ref Phase Channel B.vi"("VISA resource name"=w150, "Reference Source"=w146, "External Ref Trigger"=w126, "Internal Frequency(Hz)"=w122, "Auto Phase (T: Enabled)"=TRUE ("auto phase 2B 2"), "error in (no error)"=w147, "Manual Phase  (degree)"=0.0 ("2B reference Manual Phase 2")) -> ("VISA resource name out"=w149:refnum<visa-resource-name>, "error out"=w148:errorcluster)  [unwired: 11 in]
                  n99 = call "OE1022D_Configure_Acquisition.vi"("VISA resource name"=w149, "OE1022D A/B"=w129, "Sample time (s)"=0.001 ("2B Sample time (s) 2"), "error in (no error)"=w148, "Sample Mode (Single/Loop)"=w124) -> ("VISA resource name out"=w130:refnum<visa-resource-name>, "error out"=w131:errorcluster)  [unwired: 3 in]
                  n100 = call "OE1022D_Configure Sensitivity.vi"("VISA resource name"=w130, "OE1022D A/B"=w129, "Sensitivity"="R2 Sensitivity", "error in (no error)"=w131) -> ("VISA resource name out"=w134:refnum<visa-resource-name>, "error out"=w133:errorcluster)  [unwired: 14 in]
                  n101 = call "OE1022D_Configure Filter.vi"("Low Pass Filter Slope (1: 12dB/oct)"=w125, "Time Constant (8: 100ms)"="R2 Current T Constant", "error in (no error)"=w133, "Enable Sync Filter (F: Disable)"=w121, "OE1022D A/B"=w129, "VISA resource name"=w134) -> ("error out"=w132:errorcluster, "VISA resource name out"=w123:refnum<visa-resource-name>)  [unwired: 4 in]
                  n102 = call "OE1022D_Configure Input Filter.vi"("VISA resource name"=w123, "Input Source"=w159, "OE1022D A/B"=w129, "error in (no error)"=w132) -> ("error out"=w141:errorcluster)  [unwired: 10 in, 1 out]
                }
                frame #3 {
                  n103 = local read "System Stablization (s)"() -> (w160:dbl)
                  n104 = Multiply(x=w160, y=1000) -> (x*y=w162:dbl)
                  n105 = Wait (ms)(milliseconds to wait=w162) -> ()  [unwired: 1 out]
                }
              }
            }
          }
        }
        frame #1 {
          n106 = case shown="False" "Sweep T/F" {
            tunnel: w354 -> [w375 w1164]
            tunnel: w352 -> [w368 w1160]
            tunnel: w351 -> [w369 w1159]
            tunnel: [w362 w1150] -> w350
            tunnel: [w361 w1149] -> w349
            tunnel: w348 -> [w359 w1147]
            tunnel: w347 -> [w358 w1146]
            tunnel: w346 -> [w357 w1145]
            frame False {
              n107 = call "SetTemperature.vi"("Approach"="Fixed Temp Approach", "Rate"="FIxed T  Rate (K/min)", "Temperature"="Set Fixed T", "error in (no error)"=w369, "Instrument Ref In"=w368) -> ("error out"=w370:errorcluster, "Instrument Ref Out"=w371:refnum<k24>)  [unwired: 2 in, 1 out]
              n108 = local read "Delay(T/F)"() -> (w360:dbl)
              n109 = call "WaitFor.vi"("Delay"=w360, "Wait For Temperature"=FALSE ("WaitForTemperature"), "error in (no error)"=w370, "Instrument Ref In"=w371) -> ("error out"=w367:errorcluster, "Instrument Ref Out"=w366:refnum<k24>)  [unwired: 6 in]
              n110 = for {
                N: w375 -> [_]
                tunnel: "Low Value (Oe)" -> [w399]
                tunnel: "High Value (Oe)" -> [w421]
                shift-right: [w426] -> _
                shift-left: _ -> [w425]
                shift-right: [w420] -> _
                shift-left: _ -> [w419]
                shift-right: [w418] -> _
                shift-left: _ -> [w417]
                shift-right: [w416] -> _
                shift-left: _ -> [w415]
                tunnel: w366 -> [w414]
                tunnel: w367 -> [w413]
                shift-right: [w412] -> w362
                shift-left: _ -> [_]
                tunnel: [w411] -> w361
                tunnel: w359 -> [w410]
                tunnel: w358 -> [w409]
                tunnel: w357 -> [w408]
                shift-right: [w407] -> _
                shift-left: _ -> [w403]
                shift-right: [w406] -> _
                shift-left: _ -> [w402]
                shift-right: [w405] -> _
                shift-left: _ -> [w401]
                shift-right: [w404] -> _
                shift-left: _ -> [w400]
                tunnel: "Starting Point (Oe)" -> [w398]
                tunnel: "Step(Oe)" -> [w396]
                shift-right: [w390] -> _
                shift-left: _ -> [w389]
                shift-right: [w391] -> _
                shift-left: _ -> [w388]
                shift-right: [w386] -> _
                shift-left: _ -> [w384]
                shift-right: [w387] -> _
                shift-left: _ -> [w385]
                shift-right: [w383] -> _
                shift-left: _ -> [w382]
                shift-right: [w381] -> _
                shift-left: _ -> [w380]
                shift-right: [w379] -> _
                shift-left: _ -> [w378]
                shift-right: [w377] -> _
                shift-left: _ -> [w376]
                i -> [w423]
                n111 = Subtract(x=w421, y=w398) -> (x-y=w397:dbl)
                n112 = Subtract(x=w398, y=w399) -> (x-y=w395:dbl)
                n113 = Add(x=1, y=w423) -> (x+y=→"F loop run":i32)
                n114 = Divide(x=w397, y=w396) -> (x/y=w392:dbl)
                n115 = Divide(x=w395, y=w396) -> (x/y=w393:dbl)
                n116 = Add(x=w392, y=w393) -> (x+y=w394:dbl)
                n117 = Multiply(x=2, y=w394) -> (x*y=w428:dbl)
                n118 = Increment(x=w428) -> (x+1=w427:dbl)
                n119 = for {
                  N: w427 -> [_]
                  shift-right: [w486] -> w426
                  shift-left: w425 -> [w493]
                  shift-right: [w485] -> _
                  shift-left: _ -> [w489]
                  shift-right: [w488] -> w420
                  shift-left: w419 -> [w487]
                  shift-right: [w484] -> w418
                  shift-left: w417 -> [w483]
                  shift-right: [w482] -> w416
                  shift-left: w415 -> [w481]
                  tunnel: w414 -> [w480]
                  tunnel: w413 -> [w479]
                  shift-right: [w478] -> w412
                  shift-left: _ -> [_]
                  tunnel: [w477] -> w411
                  tunnel: w410 -> [w472]
                  tunnel: w409 -> [w471]
                  tunnel: w408 -> [w470]
                  shift-right: [w465] -> _
                  shift-left: _ -> [w460]
                  shift-right: [w464] -> w407
                  shift-left: w403 -> [w459]
                  shift-right: [w463] -> w406
                  shift-left: w402 -> [w458]
                  shift-right: [w462] -> w405
                  shift-left: w401 -> [w457]
                  shift-right: [w461] -> w404
                  shift-left: w400 -> [w456]
                  tunnel: w393 -> [w454]
                  tunnel: w392 -> [w455]
                  shift-right: [w450] -> w390
                  shift-left: w389 -> [w449]
                  shift-right: [w451] -> w391
                  shift-left: w388 -> [w448]
                  shift-right: [w444] -> w386
                  shift-left: w384 -> [w443]
                  shift-right: [w445] -> w387
                  shift-left: w385 -> [w442]
                  shift-right: [w437] -> w383
                  shift-left: w382 -> [w436]
                  shift-right: [w435] -> w381
                  shift-left: w380 -> [w434]
                  shift-right: [w433] -> w379
                  shift-left: w378 -> [w432]
                  shift-right: [w431] -> w377
                  shift-left: w376 -> [w430]
                  i -> [w491]
                  n120 = Less Or Equal?(x=w491, y=w455) -> (x <= y?=w492:bool)
                  n121 = case shown="False" w492 {
                    tunnel: w491 -> [w534 w556]
                    tunnel: [w537 w554] -> w490
                    tunnel: w455 -> [w531 _]
                    tunnel: w454 -> [w532 _]
                    frame False {
                      n122 = Multiply(x=w531, y=2) -> (x*y=w533:dbl)
                      n123 = Add(x=w533, y=w532) -> (x+y=w530:dbl)
                      n124 = Less Or Equal?(x=w534, y=w530) -> (x <= y?=w535:bool)
                      n125 = case shown="True" w535 {
                        tunnel: w534 -> [w544 w551]
                        tunnel: [w541 w548] -> w537
                        tunnel: w531 -> [_ w547]
                        tunnel: w530 -> [w540 _]
                        frame False {
                          n126 = local read "Step(Oe)"() -> (w539:i32)
                          n127 = local read "Low Value (Oe)"() -> (w538:dbl)
                          n128 = Subtract(x=w544, y=w540) -> (x-y=w543:dbl)
                          n129 = Multiply(x=w539, y=w543) -> (x*y=w542:dbl)
                          n130 = Add(x=w538, y=w542) -> (x+y=w541:dbl)
                        }
                        frame True {
                          n131 = local read "High Value (Oe)"() -> (w545:dbl)
                          n132 = local read "Step(Oe)"() -> (w546:i32)
                          n133 = Subtract(x=w551, y=w547) -> (x-y=w550:dbl)
                          n134 = Multiply(x=w546, y=w550) -> (x*y=w549:dbl)
                          n135 = Subtract(x=w545, y=w549) -> (x-y=w548:dbl)
                        }
                      }
                    }
                    frame True {
                      n136 = local read "Step(Oe)"() -> (w552:i32)
                      n137 = Multiply(x=w552, y=w556) -> (x*y=w555:i32)
                      n138 = local read "Starting Point (Oe)"() -> (w553:dbl)
                      n139 = Add(x=w553, y=w555) -> (x+y=w554:dbl)
                    }
                  }
                  n140 = stacked-sequence {
                    tunnel: w490 -> [w562 _ _ _]
                    tunnel: w493 -> [_ _ w706 _]
                    tunnel: [_ _ w705 _] -> w486
                    tunnel: [_ _ w644 _] -> w476
                    tunnel: [_ _ w704 _] -> w485
                    tunnel: w489 -> [_ _ w703 w1116]
                    tunnel: [_ _ w702 _] -> w475
                    tunnel: [_ _ w701 _] -> w488
                    tunnel: w487 -> [_ _ w694 _]
                    tunnel: [_ _ w700 _] -> w484
                    tunnel: w483 -> [_ _ w695 _]
                    tunnel: [_ _ w699 _] -> w482
                    tunnel: w481 -> [_ _ w698 _]
                    tunnel: [_ _ w697 _] -> w473
                    tunnel: [_ _ w696 _] -> w474
                    tunnel: w480 -> [w561 _ _ _]
                    tunnel: w479 -> [w560 _ _ _]
                    tunnel: [w559 _ _ _] -> w478
                    tunnel: [w558 _ _ _] -> w477
                    tunnel: [_ _ w640 _] -> w469
                    tunnel: [_ _ w639 _] -> w468
                    tunnel: [_ _ w638 _] -> w467
                    tunnel: [_ _ w637 _] -> w466
                    tunnel: [_ _ w636 _] -> w465
                    tunnel: [_ _ w635 _] -> w464
                    tunnel: [_ _ w634 _] -> w463
                    tunnel: [_ _ w633 _] -> w462
                    tunnel: [_ _ w632 _] -> w461
                    tunnel: w460 -> [_ _ w631 _]
                    tunnel: w459 -> [_ _ w630 _]
                    tunnel: w458 -> [_ _ w629 _]
                    tunnel: w457 -> [_ _ w628 _]
                    tunnel: w456 -> [_ _ w627 _]
                    tunnel: [_ _ w613 _] -> w453
                    tunnel: [_ _ w612 _] -> w452
                    tunnel: [_ _ w611 _] -> w451
                    tunnel: [_ _ w610 _] -> w450
                    tunnel: w449 -> [_ _ w608 _]
                    tunnel: w448 -> [_ _ w609 _]
                    tunnel: [_ _ w607 _] -> w447
                    tunnel: [_ _ w604 _] -> w446
                    tunnel: [_ _ w601 _] -> w445
                    tunnel: [_ _ w600 _] -> w444
                    tunnel: w443 -> [_ _ w599 _]
                    tunnel: w442 -> [_ _ w598 _]
                    tunnel: [_ _ _ w1122] -> w441
                    tunnel: [_ _ _ w1121] -> w440
                    tunnel: [_ _ _ w1120] -> w439
                    tunnel: [_ _ _ w1119] -> w438
                    tunnel: [_ _ _ w1118] -> w437
                    tunnel: w436 -> [_ _ _ w1117]
                    tunnel: [_ _ _ w1115] -> w435
                    tunnel: w434 -> [_ _ _ w1114]
                    tunnel: [_ _ _ w1113] -> w433
                    tunnel: w432 -> [_ _ _ w1112]
                    tunnel: [_ _ _ w1111] -> w431
                    tunnel: w430 -> [_ _ _ w1110]
                    frame #0 {
                      n141 = call "SetField.vi"("Mode"="Sweep F mode", "Approach"="Sweep Field Approach", "Rate"="Sweep F Rate (Oe/s)", "Field"=w562, "error in (no error)"=w560, "Instrument Ref In"=w561) -> ("error out"=w566:errorcluster, "Instrument Ref Out"=w567:refnum<k24>)  [unwired: 1 in, 1 out]
                      n142 = local read "Delay(T/F)"() -> (w557:dbl)
                      n143 = call "WaitFor.vi"("Delay"=w557, "Wait For Field"=TRUE, "error in (no error)"=w566, "Instrument Ref In"=w567) -> ("error out"=w564:errorcluster, "Instrument Ref Out"=w563:refnum<k24>)  [unwired: 6 in]
                      n144 = for {
                        N: 20 -> [_]
                        shift-right: [w592] -> _
                        shift-left: TRUE -> [w590]
                        shift-right: [w587] -> w559
                        shift-left: w564 -> [w589]
                        tunnel: w563 -> [w586]
                        tunnel: [w584] -> w558
                        tunnel: [w581] -> w577
                        tunnel: [w580] -> w576
                        tunnel: [w582] -> w574 mode=indexing
                        tunnel: [w583] -> w575 mode=indexing
                        n145 = local write "Measuring F"(w590) -> ()
                        n146 = Not(x=w590) -> (.not. x?=w592:bool)
                        n147 = call "GetTemperature.vi"("error in (no error)"=w589, "Instrument Ref In"=w586) -> ("Temperature\nStatus"=w580:i32, "Temperature"=w583:dbl, "error out"=w588:errorcluster, "Instrument Ref Out"=w585:refnum<k24>)  [unwired: 3 in, 1 out]
                        n148 = Wait (ms)(milliseconds to wait=u32 200) -> ()  [unwired: 1 out]
                        n149 = call "GetField.vi"("error in (no error)"=w588, "Instrument Ref In"=w585) -> ("Field\nStatus"=w581:i32, "Field"=w582:dbl, "error out"=w587:errorcluster, "Instrument Ref Out"=w584:refnum<k24>)  [unwired: 3 in, 1 out]
                      }
                      "Field Status" <- w577
                      "Temp Status" <- w576
                      n150 = call-poly <vilib>:"Mean.vi"("X"=w574) -> ("mean"=→"Measured Field":dbl)  [unwired: 1 out]
                      n151 = call-poly <vilib>:"Mean.vi"("X"=w575) -> ("mean"=→"Fixed Temp":dbl)  [unwired: 1 out]
                      "Field Setting" <- w562
                      "Measuring F" <- FALSE
                    }
                    frame #1 {
                      n152 = local read "System Stablization (s)"() -> (w593:dbl)
                      n153 = Multiply(x=w593, y=1000) -> (x*y=w595:dbl)
                      n154 = Wait (ms)(milliseconds to wait=w595) -> ()  [unwired: 1 out]
                    }
                    frame #2 {
                      n155 = local read "LOCKIN1 address"() -> (w643:refnum<visa-resource-name>)
                      n156 = local read "Two Lock-in ?"() -> (w641:bool)
                      n157 = local read "Measured Field"() -> (w642:dbl)
                      n158 = local read "LOCKIN3 address"() -> (w597:refnum<visa-resource-name>)
                      n159 = local read "Current measurement?"() -> (w596:bool)
                      n160 = case shown="True" w641 {
                        tunnel: [w752 w794] -> w638
                        tunnel: [w752 w793] -> w637
                        tunnel: [w752 w792] -> w639
                        tunnel: [w752 w791] -> w640
                        tunnel: [w751 w790] -> w632
                        tunnel: [w756 w789] -> w636
                        tunnel: w631 -> [w756 w788]
                        tunnel: w627 -> [w751 w785]
                        tunnel: [w755 w787] -> w635
                        tunnel: w630 -> [w755 w786]
                        tunnel: [w754 w784] -> w634
                        tunnel: w629 -> [w754 w783]
                        tunnel: [w753 w782] -> w633
                        tunnel: w628 -> [w753 w781]
                        tunnel: w642 -> [_ w780]
                        tunnel: [w752 w764] -> w613
                        tunnel: [w752 w763] -> w612
                        tunnel: [w751 w760] -> w611
                        tunnel: [w751 w759] -> w610
                        tunnel: w609 -> [_ w758]
                        tunnel: w608 -> [_ w757]
                        frame False {
                          w752 = nan
                        }
                        frame True {
                          n161 = flat-sequence {
                            tunnel: w788 -> [w871]
                            tunnel: [w869] -> w843
                            tunnel: [w862] -> w842
                            tunnel: [w863] -> w841
                            tunnel: [w860] -> w840
                            tunnel: [w863] -> w839
                            tunnel: [w863] -> w838
                            tunnel: [w863] -> w837
                            tunnel: [w863] -> w836
                            tunnel: [w862] -> w835
                            tunnel: [w861] -> w834
                            tunnel: [w860] -> w833
                            tunnel: [w859] -> w832
                            tunnel: ["F Clear Plot 2B"] -> w831
                            tunnel: ["F Clear Plot 2A"] -> w830
                            tunnel: [w850] -> w829
                            tunnel: [w852] -> w828
                            tunnel: [w851] -> w827
                            tunnel: [w856] -> w826
                            tunnel: [w855] -> w825
                            tunnel: w786 -> [w846]
                            tunnel: w783 -> [w845]
                            tunnel: w780 -> [w844]
                            tunnel: w843 -> [w893]
                            tunnel: [w893] -> w824
                            tunnel: w842 -> [w892]
                            tunnel: [w892] -> w823
                            tunnel: w841 -> [w891]
                            tunnel: [w891] -> w822
                            tunnel: w840 -> [w890]
                            tunnel: [w890] -> w821
                            tunnel: w839 -> [w889]
                            tunnel: [w889] -> w820
                            tunnel: w838 -> [w888]
                            tunnel: [w888] -> w819
                            tunnel: w837 -> [w887]
                            tunnel: [w887] -> w818
                            tunnel: w836 -> [w886]
                            tunnel: [w886] -> w817
                            tunnel: w835 -> [w885]
                            tunnel: [w885] -> w816
                            tunnel: w834 -> [w884]
                            tunnel: [w884] -> w815
                            tunnel: w833 -> [w883]
                            tunnel: [w883] -> w814
                            tunnel: w832 -> [w882]
                            tunnel: [w882] -> w813
                            tunnel: w831 -> [w881]
                            tunnel: [w881] -> w812
                            tunnel: w830 -> [w880]
                            tunnel: [w880] -> w811
                            tunnel: w829 -> [w879]
                            tunnel: [w879] -> w810
                            tunnel: w828 -> [w878]
                            tunnel: [w878] -> w809
                            tunnel: w827 -> [w877]
                            tunnel: [w877] -> w808
                            tunnel: w826 -> [w876]
                            tunnel: [w876] -> w807
                            tunnel: w825 -> [w875]
                            tunnel: [w875] -> w806
                            tunnel: w824 -> [w902]
                            tunnel: w823 -> [w931]
                            tunnel: w822 -> [w930]
                            tunnel: w821 -> [w929]
                            tunnel: w820 -> [w928]
                            tunnel: w819 -> [w926]
                            tunnel: w818 -> [w924]
                            tunnel: w817 -> [w894]
                            tunnel: w816 -> [w920]
                            tunnel: w815 -> [w919]
                            tunnel: w814 -> [w916]
                            tunnel: w813 -> [w915]
                            tunnel: w812 -> [w895]
                            tunnel: w781 -> [w912]
                            tunnel: w811 -> [w911]
                            tunnel: w810 -> [w907]
                            tunnel: w809 -> [w897]
                            tunnel: w808 -> [w906]
                            tunnel: w807 -> [w903]
                            tunnel: w806 -> [w896]
                            tunnel: [w902] -> w805
                            tunnel: [w918] -> w804
                            tunnel: [w931] -> w803
                            tunnel: [w930] -> w802
                            tunnel: [w900] -> w801
                            tunnel: [w901] -> w800
                            tunnel: [w921] -> w799
                            tunnel: [w917] -> w798
                            tunnel: [w914] -> w797
                            tunnel: [w929] -> w796
                            tunnel: [w905] -> w795
                            tunnel: w785 -> [w898]
                            tunnel: [w897] -> w767
                            tunnel: [w895] -> w766
                            tunnel: [w894] -> w761
                            tunnel: w805 -> [w946]
                            tunnel: w804 -> [w945]
                            tunnel: w803 -> [w935]
                            tunnel: w802 -> [w944]
                            tunnel: w801 -> [w943]
                            tunnel: w800 -> [w942]
                            tunnel: w799 -> [w941]
                            tunnel: w798 -> [w940]
                            tunnel: w797 -> [w939]
                            tunnel: w796 -> [w938]
                            tunnel: w795 -> [w937]
                            tunnel: [w946] -> w779
                            tunnel: [w945] -> w778
                            tunnel: [w944] -> w777
                            tunnel: [w943] -> w776
                            tunnel: [w942] -> w775
                            tunnel: [w941] -> w774
                            tunnel: [w940] -> w773
                            tunnel: [w939] -> w772
                            tunnel: [w938] -> w771
                            tunnel: [w937] -> w770
                            tunnel: [w935] -> w769
                            tunnel: [w934] -> w768
                            tunnel: w767 -> [w934]
                            tunnel: w766 -> [w933]
                            tunnel: [w933] -> w765
                            tunnel: [w932] -> w762
                            tunnel: w761 -> [w932]
                            tunnel: [w967] -> w794
                            tunnel: [w968] -> w791
                            tunnel: [w969] -> w793
                            tunnel: [w970] -> w784
                            tunnel: [w971] -> w790
                            tunnel: [w972] -> w782
                            tunnel: [w973] -> _
                            tunnel: [w974] -> w792
                            tunnel: [w975] -> w789
                            tunnel: [w976] -> w787
                            tunnel: w779 -> [w966]
                            tunnel: w778 -> [w976]
                            tunnel: w777 -> [w975]
                            tunnel: w776 -> [w974]
                            tunnel: w775 -> [w973]
                            tunnel: w774 -> [w972]
                            tunnel: w773 -> [w971]
                            tunnel: w772 -> [w970]
                            tunnel: w771 -> [w969]
                            tunnel: w770 -> [w968]
                            tunnel: w769 -> [w967]
                            tunnel: w768 -> [w965]
                            tunnel: w765 -> [w964]
                            tunnel: [w960] -> w764
                            tunnel: [w949] -> w763
                            tunnel: w762 -> [w956]
                            tunnel: [w955] -> w760
                            tunnel: [w954] -> w759
                            tunnel: w758 -> [w953]
                            tunnel: w757 -> [w952]
                            frame #0 {
                              w852 = u8 1 items=["Channel A", "Channel B"] ("Channel A/B for Parameter1")
                              w855 = u8 0 items=["Channel A", "Channel B"] ("Channel A/B for Parameter1")
                              n162 = local read "LOCKIN2 address"() -> (w847:refnum<visa-resource-name>)
                              n163 = Format Into String(0) -> (error out=w870:errorcluster)  [unwired: 3 in, 1 out]
                              n164 = Format Into String(0) -> (error out=w853:errorcluster)  [unwired: 3 in, 1 out]
                              n165 = call "OE1022D_Read 1 parameter_mean.vi"("错误输入（无错误）"=w870, "Parameter"="Parameter 2A 2", "Channel (0: A)"=w855, "VISA resource name"=w847) -> ("error out"=w856:errorcluster, "Measurement"=w864:dbl, "VISA resource name out"=w869:refnum<visa-resource-name>)  [unwired: 5 in]
                              n166 = call "OE1022D_Read 1 parameter_mean.vi"("Parameter 2"="Parameter 2B 2", "错误输入（无错误）"=w853, "Channel (0: A)"=w852, "VISA resource name"=w847) -> ("error out"=w850:errorcluster, "Measurement"=w849:dbl, "VISA resource name out"=w851:refnum<visa-resource-name>)  [unwired: 5 in]
                              n167 = Multiply(x=w864, y=1000.0) -> (x*y=w862:dbl)
                              "Vaa_2_F (mV)" <- w862
                              n168 = Multiply(x=w849, y=1000000.0) -> (x*y=w860:dbl)
                              "Vab_2_F (uV) 1w" <- w860
                              n169 = Build Array(w862) -> (w872:dbl[])
                              n170 = Build Array(w860) -> (w866:dbl[])
                              n171 = Select(t=w872, s="F Clear Plot 2A", f=w846) -> (s? t:f=w861:dbl[])
                              n172 = Select(t=w866, s="F Clear Plot 2B", f=w845) -> (s? t:f=w859:dbl[])
                              n173 = Build Array (concatenate)(w844, w871) -> (w863:dbl[])
                            }
                            frame #1 {
                              n174 = Wait (ms)(milliseconds to wait=u32 50) -> ()  [unwired: 1 out]
                            }
                            frame #2 {
                              n175 = Build Array (concatenate)(w920, w919) -> (w918:dbl[])
                              n176 = Build Array (concatenate)(w916, w915) -> (w914:dbl[])
                              n177 = Bundle(w924, w918) -> (→"Vaa_2_F":cluster{dbl[], dbl[]})  [unwired: 1 in]
                              n178 = Bundle(w926, w914) -> (→"Vab_2_F 1w":cluster{dbl[], dbl[]})  [unwired: 1 in]
                              n179 = call "OE1022D_Read 1 parameter_mean.vi"("错误输入（无错误）"=w903, "Parameter"="Phase 2A  2", "Channel (0: A)"=w896, "VISA resource name"=w902) -> ("error out"=w901:errorcluster, "Measurement"=w900:dbl)  [unwired: 5 in, 1 out]
                              "phase Vaa_2_F" <- w900
                              n180 = call "OE1022D_Read 1 parameter_mean.vi"("Parameter 2"="Phase 2B 2", "错误输入（无错误）"=w907, "Channel (0: A)"=w897, "VISA resource name"=w906) -> ("Measurement"=w905:dbl)  [unwired: 5 in, 2 out]
                              "phase Vab_2_F 1w" <- w905
                              n181 = Build Array(w900) -> (w908:dbl[])
                              n182 = Build Array(w905) -> (w909:dbl[])
                              n183 = Select(t=w908, s=w911, f=w912) -> (s? t:f=w910:dbl[])
                              n184 = Select(t=w909, s=w895, f=w898) -> (s? t:f=w913:dbl[])
                              n185 = Build Array (concatenate)(w900, w910) -> (w921:dbl[])
                              n186 = Build Array (concatenate)(w905, w913) -> (w917:dbl[])
                              n187 = Bundle(w894, w921) -> (→"phase Vaa_2_F":cluster{dbl[], dbl[]})  [unwired: 1 in]
                              n188 = Bundle(w928, w917) -> (→"phase Vab_2_F 1w":cluster{dbl[], dbl[]})  [unwired: 1 in]
                            }
                            frame #3 {
                              n189 = Wait (ms)(milliseconds to wait=u32 50) -> ()  [unwired: 1 out]
                            }
                            frame #4 {
                              n190 = call "OE1022D_Read 1 parameter_mean.vi"("Parameter 2"="Parameter 2B 3", "Channel (0: A)"=w965, "VISA resource name"=w966) -> ("Measurement"=w950:dbl)  [unwired: 6 in, 2 out]
                              n191 = call "OE1022D_Read 1 parameter_mean.vi"("Parameter 2"="Phase 2B 3", "Channel (0: A)"=w965, "VISA resource name"=w966) -> ("Measurement"=w960:dbl)  [unwired: 6 in, 2 out]
                              "Phase Vab_2_F 2w" <- w960
                              n192 = Multiply(x=1000000.0, y=w950) -> (x*y=w949:dbl)
                              "Vab_2_F (uV) 2w" <- w949
                              n193 = Build Array(w949) -> (w962:dbl[])
                              n194 = Build Array(w960) -> (w963:dbl[])
                              n195 = Select(t=w962, s=w964, f=w952) -> (s? t:f=w959:dbl[])
                              n196 = Select(t=w963, s=w964, f=w953) -> (s? t:f=w961:dbl[])
                              n197 = Build Array (concatenate)(w949, w959) -> (w954:dbl[])
                              n198 = Build Array (concatenate)(w960, w961) -> (w955:dbl[])
                              n199 = Bundle(w956, w954) -> (→"Vab_2_F  2w":cluster{dbl[], dbl[]})  [unwired: 1 in]
                              n200 = Bundle(w956, w955) -> (→"Phase Vab_2_F 2w":cluster{dbl[], dbl[]})  [unwired: 1 in]
                            }
                          }
                        }
                      }
                      n201 = flat-sequence {
                        tunnel: w706 -> [w1004]
                        tunnel: w703 -> [w1003]
                        tunnel: w698 -> [w995]
                        tunnel: [w1001] -> w693
                        tunnel: [w989] -> w691
                        tunnel: [w990] -> w689
                        tunnel: [w987] -> w687
                        tunnel: [w990] -> w685
                        tunnel: [w990] -> w683
                        tunnel: [w990] -> w681
                        tunnel: [w990] -> w679
                        tunnel: [w989] -> w677
                        tunnel: [w988] -> w675
                        tunnel: [w987] -> w673
                        tunnel: [w986] -> w671
                        tunnel: ["F Clear Plot 1B"] -> w669
                        tunnel: ["F Clear Plot 1A"] -> w667
                        tunnel: [w983] -> w665
                        tunnel: [w982] -> w663
                        tunnel: [w981] -> w661
                        tunnel: [w980] -> w659
                        tunnel: [w979] -> w657
                        tunnel: w642 -> [w978]
                        tunnel: w643 -> [w977]
                        tunnel: w693 -> [w1026]
                        tunnel: [w1026] -> w692
                        tunnel: w691 -> [w1025]
                        tunnel: [w1025] -> w690
                        tunnel: w689 -> [w1024]
                        tunnel: [w1024] -> w688
                        tunnel: w687 -> [w1023]
                        tunnel: [w1023] -> w686
                        tunnel: w685 -> [w1022]
                        tunnel: [w1022] -> w684
                        tunnel: w683 -> [w1021]
                        tunnel: [w1021] -> w682
                        tunnel: w681 -> [w1020]
                        tunnel: [w1020] -> w680
                        tunnel: w679 -> [w1019]
                        tunnel: [w1019] -> w678
                        tunnel: w677 -> [w1018]
                        tunnel: [w1018] -> w676
                        tunnel: w675 -> [w1017]
                        tunnel: [w1017] -> w674
                        tunnel: w673 -> [w1016]
                        tunnel: [w1016] -> w672
                        tunnel: w671 -> [w1015]
                        tunnel: [w1015] -> w670
                        tunnel: w669 -> [w1014]
                        tunnel: [w1014] -> w668
                        tunnel: w667 -> [w1013]
                        tunnel: [w1013] -> w666
                        tunnel: w665 -> [w1012]
                        tunnel: [w1012] -> w664
                        tunnel: w663 -> [w1011]
                        tunnel: [w1011] -> w662
                        tunnel: w661 -> [w1010]
                        tunnel: [w1010] -> w660
                        tunnel: w659 -> [w1009]
                        tunnel: [w1009] -> w658
                        tunnel: w657 -> [w1008]
                        tunnel: [w1008] -> w656
                        tunnel: w692 -> [w1034]
                        tunnel: w690 -> [w1064]
                        tunnel: w688 -> [w1063]
                        tunnel: w686 -> [w1062]
                        tunnel: w684 -> [w1028]
                        tunnel: w682 -> [w1060]
                        tunnel: w680 -> [w1058]
                        tunnel: w678 -> [w1056]
                        tunnel: w676 -> [w1053]
                        tunnel: w674 -> [w1052]
                        tunnel: w672 -> [w1049]
                        tunnel: w670 -> [w1048]
                        tunnel: w695 -> [w1046]
                        tunnel: w668 -> [w1029]
                        tunnel: w694 -> [w1044]
                        tunnel: w666 -> [w1043]
                        tunnel: w664 -> [w1027]
                        tunnel: w662 -> [w1030]
                        tunnel: w660 -> [w1039]
                        tunnel: w658 -> [w1036]
                        tunnel: w656 -> [w1035]
                        tunnel: [w1034] -> w655
                        tunnel: [w1051] -> w654
                        tunnel: [w1064] -> w653
                        tunnel: [w1063] -> w652
                        tunnel: [w1032] -> w651
                        tunnel: [w1033] -> w650
                        tunnel: [w1054] -> w649
                        tunnel: [w1050] -> w648
                        tunnel: [w1047] -> w647
                        tunnel: [w1062] -> w646
                        tunnel: [w1038] -> w645
                        tunnel: [w1030] -> w615
                        tunnel: [w1029] -> w606
                        tunnel: [w1028] -> w602
                        tunnel: w655 -> [w1065]
                        tunnel: w654 -> [w1079]
                        tunnel: w653 -> [w1078]
                        tunnel: w652 -> [w1077]
                        tunnel: w651 -> [w1076]
                        tunnel: w650 -> [w1075]
                        tunnel: w649 -> [w1074]
                        tunnel: w648 -> [w1073]
                        tunnel: w647 -> [w1072]
                        tunnel: w646 -> [w1071]
                        tunnel: w645 -> [w1070]
                        tunnel: [w1079] -> w626
                        tunnel: [w1078] -> w625
                        tunnel: [w1077] -> w624
                        tunnel: [w1076] -> w623
                        tunnel: [w1075] -> w622
                        tunnel: [w1074] -> w621
                        tunnel: [w1073] -> w620
                        tunnel: [w1072] -> w619
                        tunnel: [w1071] -> w618
                        tunnel: [w1070] -> w617
                        tunnel: [w1065] -> w616
                        tunnel: w615 -> [w1068]
                        tunnel: [w1068] -> w614
                        tunnel: w606 -> [w1067]
                        tunnel: [w1067] -> w605
                        tunnel: [w1066] -> w603
                        tunnel: w602 -> [w1066]
                        tunnel: [w1100] -> w696
                        tunnel: [w1101] -> w697
                        tunnel: [w1102] -> w699
                        tunnel: [w1103] -> w700
                        tunnel: [w1104] -> w701
                        tunnel: [w1105] -> _
                        tunnel: [w1106] -> w702
                        tunnel: [w1107] -> w704
                        tunnel: [w1108] -> w644
                        tunnel: [w1109] -> w705
                        tunnel: w626 -> [w1109]
                        tunnel: w625 -> [w1108]
                        tunnel: w624 -> [w1107]
                        tunnel: w623 -> [w1106]
                        tunnel: w622 -> [w1105]
                        tunnel: w621 -> [w1104]
                        tunnel: w620 -> [w1103]
                        tunnel: w619 -> [w1102]
                        tunnel: w618 -> [w1101]
                        tunnel: w617 -> [w1100]
                        tunnel: w616 -> [w1099]
                        tunnel: w614 -> [w1098]
                        tunnel: [w1091] -> w607
                        tunnel: w605 -> [w1090]
                        tunnel: [w1082] -> w604
                        tunnel: w603 -> [w1089]
                        tunnel: [w1088] -> w601
                        tunnel: [w1087] -> w600
                        tunnel: w599 -> [w1086]
                        tunnel: w598 -> [w1085]
                        frame #0 {
                          w982 = u8 1 items=["Channel A", "Channel B"] ("Channel A/B for Parameter1")
                          w979 = u8 0 items=["Channel A", "Channel B"] ("Channel A/B for Parameter1")
                          n202 = Format Into String(0) -> (error out=w1002:errorcluster)  [unwired: 3 in, 1 out]
                          n203 = Format Into String(0) -> (error out=w997:errorcluster)  [unwired: 3 in, 1 out]
                          n204 = call "OE1022D_Read 1 parameter_mean.vi"("错误输入（无错误）"=w1002, "Parameter"="Parameter 1A 2", "Channel (0: A)"=w979, "VISA resource name"=w977) -> ("error out"=w980:errorcluster, "Measurement"=w992:dbl, "VISA resource name out"=w1001:refnum<visa-resource-name>)  [unwired: 5 in]
                          n205 = call "OE1022D_Read 1 parameter_mean.vi"("Parameter 2"="Parameter 1B 2", "错误输入（无错误）"=w997, "Channel (0: A)"=w982, "VISA resource name"=w977) -> ("error out"=w983:errorcluster, "Measurement"=w991:dbl, "VISA resource name out"=w981:refnum<visa-resource-name>)  [unwired: 5 in]
                          n206 = Multiply(x=w992, y=1000.0) -> (x*y=w989:dbl)
                          "Vaa_1_F (mV)" <- w989
                          n207 = Multiply(x=w991, y=1000000.0) -> (x*y=w987:dbl)
                          "Vab_1_F (uV) 1w" <- w987
                          n208 = Build Array(w989) -> (w1005:dbl[])
                          n209 = Build Array(w987) -> (w998:dbl[])
                          n210 = Select(t=w1005, s="F Clear Plot 1A", f=w1004) -> (s? t:f=w988:dbl[])
                          n211 = Select(t=w998, s="F Clear Plot 1B", f=w995) -> (s? t:f=w986:dbl[])
                          n212 = Build Array (concatenate)(w978, w1003) -> (w990:dbl[])
                        }
                        frame #1 {
                          n213 = Wait (ms)(milliseconds to wait=u32 50) -> ()  [unwired: 1 out]
                        }
                        frame #2 {
                          n214 = Build Array (concatenate)(w1053, w1052) -> (w1051:dbl[])
                          n215 = Build Array (concatenate)(w1049, w1048) -> (w1047:dbl[])
                          n216 = Bundle(w1058, w1051) -> (→"Vaa_1_F":cluster{dbl[], dbl[]})  [unwired: 1 in]
                          n217 = Bundle(w1060, w1047) -> (→"Vab_1_F 1w":cluster{dbl[], dbl[]})  [unwired: 1 in]
                          n218 = call "OE1022D_Read 1 parameter_mean.vi"("错误输入（无错误）"=w1036, "Parameter"="Phase 1A 2", "Channel (0: A)"=w1035, "VISA resource name"=w1034) -> ("error out"=w1033:errorcluster, "Measurement"=w1032:dbl)  [unwired: 5 in, 1 out]
                          "phase Vaa_1_F" <- w1032
                          n219 = call "OE1022D_Read 1 parameter_mean.vi"("Parameter 2"="Phase 1B 2", "错误输入（无错误）"=w1027, "Channel (0: A)"=w1030, "VISA resource name"=w1039) -> ("Measurement"=w1038:dbl)  [unwired: 5 in, 2 out]
                          "phase Vab_1_F 1w" <- w1038
                          n220 = Build Array(w1032) -> (w1040:dbl[])
                          n221 = Build Array(w1038) -> (w1041:dbl[])
                          n222 = Select(t=w1040, s=w1043, f=w1044) -> (s? t:f=w1042:dbl[])
                          n223 = Select(t=w1041, s=w1029, f=w1046) -> (s? t:f=w1045:dbl[])
                          n224 = Build Array (concatenate)(w1032, w1042) -> (w1054:dbl[])
                          n225 = Build Array (concatenate)(w1038, w1045) -> (w1050:dbl[])
                          n226 = Bundle(w1056, w1054) -> (→"phase Vaa_1_F":cluster{dbl[], dbl[]})  [unwired: 1 in]
                          n227 = Bundle(w1028, w1050) -> (→"phase Vab_1_F 1w":cluster{dbl[], dbl[]})  [unwired: 1 in]
                        }
                        frame #3 {
                          n228 = Wait (ms)(milliseconds to wait=u32 50) -> ()  [unwired: 1 out]
                        }
                        frame #4 {
                          n229 = call "OE1022D_Read 1 parameter_mean.vi"("Parameter 2"="Parameter 1B 3", "Channel (0: A)"=w1098, "VISA resource name"=w1099) -> ("Measurement"=w1083:dbl)  [unwired: 6 in, 2 out]
                          n230 = call "OE1022D_Read 1 parameter_mean.vi"("Parameter 2"="Phase 1B 3", "Channel (0: A)"=w1098, "VISA resource name"=w1099) -> ("Measurement"=w1091:dbl)  [unwired: 6 in, 2 out]
                          "Phase Vab_1_F 2w" <- w1091
                          n231 = Multiply(x=1000000.0, y=w1083) -> (x*y=w1082:dbl)
                          "Vab_1_F (uV) 2w" <- w1082
                          n232 = Build Array(w1082) -> (w1094:dbl[])
                          n233 = Build Array(w1091) -> (w1097:dbl[])
                          n234 = Select(t=w1094, s=w1090, f=w1086) -> (s? t:f=w1093:dbl[])
                          n235 = Select(t=w1097, s=w1090, f=w1085) -> (s? t:f=w1096:dbl[])
                          n236 = Build Array (concatenate)(w1082, w1093) -> (w1087:dbl[])
                          n237 = Build Array (concatenate)(w1091, w1096) -> (w1088:dbl[])
                          n238 = Bundle(w1089, w1087) -> (→"Vab_1_F 2w":cluster{dbl[], dbl[]})  [unwired: 1 in]
                          n239 = Bundle(w1089, w1088) -> (→"Phase Vab_1_F 2w":cluster{dbl[], dbl[]})  [unwired: 1 in]
                        }
                      }
                      n240 = case shown="True" w596 {
                        tunnel: w597 -> [_ w715]
                        frame False {
                        }
                        frame True {
                          n241 = flat-sequence {
                            tunnel: w715 -> [w729]
                            tunnel: [w728] -> w713
                            tunnel: [w727] -> w712
                            tunnel: [w726] -> w709
                            tunnel: [w725] -> w707
                            tunnel: [w738] -> w714
                            tunnel: w713 -> [w738]
                            tunnel: w712 -> [w737]
                            tunnel: [w737] -> w711
                            tunnel: [w736] -> w710
                            tunnel: w709 -> [w736]
                            tunnel: [w735] -> w708
                            tunnel: w707 -> [w735]
                            tunnel: w714 -> [w749]
                            tunnel: w711 -> [w748]
                            tunnel: w710 -> [w747]
                            tunnel: w708 -> [w746]
                            frame #0 {
                              w722 = u16 2 items=["X", "Y", "R", "Theta", "Frequency", "Noise", "Xh1", "Yh1", "Rh1", "Theta h1", "Xh2", "Yh2", "Rh2", "Theta h2"] ("Parameter 2")
                              w723 = u16 2 items=["X", "Y", "R", "Theta", "Frequency", "Noise", "Xh1", "Yh1", "Rh1", "Theta h1", "Xh2", "Yh2", "Rh2", "Theta h2"] ("Parameter")
                              w724 = u16 1 items=["Channel A", "Channel B", "ADC"] ("Channel (0: A)")
                              w730 = u16 0 items=["Channel A", "Channel B", "ADC"] ("Channel (0: A)")
                              n242 = Format Into String(0) -> (error out=w732:errorcluster)  [unwired: 3 in, 1 out]
                              n243 = Format Into String(0) -> (error out=w731:errorcluster)  [unwired: 3 in, 1 out]
                              n244 = call "OE1022D_Read 1 parameter_mean.vi"("错误输入（无错误）"=w732, "Parameter"=w723, "Channel (0: A)"=w730, "VISA resource name"=w729) -> ("error out"=w727:errorcluster, "Measurement"=w721:dbl, "VISA resource name out"=w728:refnum<visa-resource-name>)  [unwired: 5 in]
                              n245 = call "OE1022D_Read 1 parameter_mean.vi"("Parameter 2"=w722, "错误输入（无错误）"=w731, "Channel (0: A)"=w724, "VISA resource name"=w729) -> ("error out"=w725:errorcluster, "Measurement"=w716:dbl, "VISA resource name out"=w726:refnum<visa-resource-name>)  [unwired: 5 in]
                              n246 = local read "R2(Kohm)"() -> (w719:dbl)
                              n247 = local read "R1(Kohm)"() -> (w720:dbl)
                              n248 = Divide(x=w716, y=w719) -> (x/y=→"Device2 Current(mA)":dbl)
                              n249 = Divide(x=w721, y=w720) -> (x/y=→"Device1 Current(mA)":dbl)
                            }
                            frame #1 {
                              n250 = Wait (ms)(milliseconds to wait=u32 50) -> ()  [unwired: 1 out]
                            }
                            frame #2 {
                              w742 = u16 3 items=["X", "Y", "R", "Theta", "Frequency", "Noise", "Xh1", "Yh1", "Rh1", "Theta h1", "Xh2", "Yh2", "Rh2", "Theta h2"] ("Parameter 2")
                              w743 = u16 1 items=["Channel A", "Channel B", "ADC"] ("Channel (0: A)")
                              w744 = u16 3 items=["X", "Y", "R", "Theta", "Frequency", "Noise", "Xh1", "Yh1", "Rh1", "Theta h1", "Xh2", "Yh2", "Rh2", "Theta h2"] ("Parameter")
                              w745 = u16 0 items=["Channel A", "Channel B", "ADC"] ("Channel (0: A)")
                              n251 = call "OE1022D_Read 1 parameter_mean.vi"("错误输入（无错误）"=w748, "Parameter"=w744, "Channel (0: A)"=w745, "VISA resource name"=w749) -> ("Measurement"=→"Device 1 phase":dbl)  [unwired: 5 in, 2 out]
                              n252 = call "OE1022D_Read 1 parameter_mean.vi"("Parameter 2"=w742, "错误输入（无错误）"=w746, "Channel (0: A)"=w743, "VISA resource name"=w747) -> ("Measurement"=→"Device 2 phase":dbl)  [unwired: 5 in, 2 out]
                            }
                            frame #3 {
                              n253 = Wait (ms)(milliseconds to wait=u32 50) -> ()  [unwired: 1 out]
                            }
                          }
                        }
                      }
                    }
                    frame #3 {
                      n254 = local read "Measured Field"() -> (w1128:dbl)
                      n255 = local read "Device1 Current(mA)"() -> (w1143:dbl)
                      n256 = local read "Vaa_1_F (mV)"() -> (w1144:dbl)
                      n257 = local read "Device2 Current(mA)"() -> (w1141:dbl)
                      n258 = local read "Vaa_2_F (mV)"() -> (w1142:dbl)
                      n259 = Build Array (concatenate)(w1128, w1116) -> (w1123:dbl[])
                      n260 = Divide(x=w1144, y=w1143) -> (x/y=w1122:dbl)
                      "Ri_1(Ohm)" <- w1122
                      n261 = Divide(x=w1142, y=w1141) -> (x/y=w1120:dbl)
                      "Ri_2(Ohm)" <- w1120
                      n262 = local read "F Clear Plot 2A"() -> (w1125:bool)
                      n263 = local read "F Clear Plot 1A"() -> (w1124:bool)
                      n264 = Build Array(w1120) -> (w1139:dbl[])
                      n265 = Build Array(w1122) -> (w1140:dbl[])
                      n266 = Select(t=w1139, s=w1125, f=w1114) -> (s? t:f=w1129:dbl[])
                      n267 = Select(t=w1140, s=w1124, f=w1117) -> (s? t:f=w1136:dbl[])
                      n268 = Build Array (concatenate)(w1120, w1129) -> (w1115:dbl[])
                      n269 = Build Array (concatenate)(w1122, w1136) -> (w1118:dbl[])
                      n270 = Bundle(w1123, w1115) -> (→"Ri_2":cluster{dbl[], dbl[]})  [unwired: 1 in]
                      n271 = Bundle(w1123, w1118) -> (→"Ri_1":cluster{dbl[], dbl[]})  [unwired: 1 in]
                      n272 = local read "F Clear Plot 1B"() -> (w1127:bool)
                      n273 = local read "F Clear Plot 2B"() -> (w1126:bool)
                      n274 = local read "Device 1 phase"() -> (w1121:dbl)
                      n275 = local read "Device 2 phase"() -> (w1119:dbl)
                      n276 = Build Array(w1121) -> (w1135:dbl[])
                      n277 = Build Array(w1119) -> (w1132:dbl[])
                      n278 = Select(t=w1135, s=w1127, f=w1112) -> (s? t:f=w1133:dbl[])
                      n279 = Select(t=w1132, s=w1126, f=w1110) -> (s? t:f=w1130:dbl[])
                      n280 = Build Array (concatenate)(w1121, w1133) -> (w1113:dbl[])
                      n281 = Build Array (concatenate)(w1119, w1130) -> (w1111:dbl[])
                      n282 = Bundle(w1123, w1113) -> (→"Ri_1 phase":cluster{dbl[], dbl[]})  [unwired: 1 in]
                      n283 = Bundle(w1123, w1111) -> (→"Ri_2 phase":cluster{dbl[], dbl[]})  [unwired: 1 in]
                    }
                  }
                  n284 = case shown="True" w471 {
                    tunnel: w476 -> [_ w512]
                    tunnel: w472 -> [_ w515]
                    tunnel: w475 -> [_ w511]
                    tunnel: w473 -> [_ w510]
                    tunnel: w474 -> [_ w509]
                    tunnel: w470 -> [_ w508]
                    tunnel: w469 -> [_ w505]
                    tunnel: w468 -> [_ w504]
                    tunnel: w467 -> [_ w503]
                    tunnel: w466 -> [_ w502]
                    tunnel: w453 -> [_ w501]
                    tunnel: w452 -> [_ w500]
                    tunnel: w447 -> [_ w499]
                    tunnel: w446 -> [_ w498]
                    tunnel: w441 -> [_ w497]
                    tunnel: w440 -> [_ w496]
                    tunnel: w439 -> [_ w495]
                    tunnel: w438 -> [_ w494]
                    frame False {
                    }
                    frame True {
                      n285 = local read "Measured Field"() -> (w506:dbl)
                      n286 = local read "Two Lock-in ?"() -> (w507:bool)
                      n287 = Build Array(w506, w512, w511, w510, w509, w498, w499, w497, w496) -> (w514:dbl[])
                      n288 = case shown="True" w507 {
                        tunnel: w506 -> [_ w526]
                        tunnel: w503 -> [_ w525]
                        tunnel: w504 -> [_ w524]
                        tunnel: w505 -> [_ w523]
                        tunnel: w502 -> [_ w522]
                        tunnel: w508 -> [_ w521]
                        tunnel: w501 -> [_ w520]
                        tunnel: w500 -> [_ w519]
                        tunnel: w495 -> [_ w518]
                        tunnel: w494 -> [_ w517]
                        frame False {
                        }
                        frame True {
                          n289 = Build Array(w526, w525, w522, w524, w523, w519, w520, w518, w517) -> (w528:dbl[])
                          n290 = call-poly <vilib>:"Write Delimited Spreadsheet.vi"("file path (dialog if empty)"=w521, "format (%.3f)"="%.10f", "1D data"=w528, "append to file? (new file:F)"=TRUE) -> ()  [unwired: 10 in, 2 out]
                        }
                      }
                      n291 = call-poly <vilib>:"Write Delimited Spreadsheet.vi"("file path (dialog if empty)"=w515, "format (%.3f)"="%.10f", "1D data"=w514, "append to file? (new file:F)"=TRUE) -> ()  [unwired: 10 in, 2 out]
                    }
                  }
                }
              }
            }
            frame True {
              n292 = call "SetField.vi"("Mode"="Fixed F mode", "Approach"="Fixed Field Approach", "Rate"="FIxed F Rate (Oe/s)", "Field"="Set FIxed F (Oe)", "error in (no error)"=w1159, "Instrument Ref In"=w1160) -> ("error out"=w1155:errorcluster, "Instrument Ref Out"=w1157:refnum<k24>)  [unwired: 1 in, 1 out]
              n293 = local read "Delay(T/F)"() -> (w1148:dbl)
              n294 = call "WaitFor.vi"("Delay"=w1148, "Wait For Field"=TRUE, "error in (no error)"=w1155, "Instrument Ref In"=w1157) -> ("error out"=w1156:errorcluster, "Instrument Ref Out"=w1158:refnum<k24>)  [unwired: 6 in]
              n295 = for {
                N: w1164 -> [_]
                tunnel: "Low Value (K)" -> [w1195]
                tunnel: "High Value (K)" -> [w1186]
                shift-right: [w1191] -> _
                shift-left: _ -> [w1190]
                shift-right: [w1185] -> _
                shift-left: _ -> [w1184]
                shift-right: [w1183] -> _
                shift-left: _ -> [w1182]
                shift-right: [w1181] -> _
                shift-left: _ -> [w1180]
                tunnel: w1158 -> [w1179]
                tunnel: w1156 -> [w1178]
                tunnel: [w1177] -> w1150
                tunnel: [w1176] -> w1149
                tunnel: w1147 -> [w1175]
                tunnel: w1146 -> [w1174]
                shift-right: [w1173] -> _
                shift-left: _ -> [w1172]
                shift-right: [w1171] -> _
                shift-left: _ -> [w1170]
                shift-right: [w1169] -> _
                shift-left: _ -> [w1168]
                shift-right: [w1167] -> _
                shift-left: _ -> [w1166]
                tunnel: w1145 -> [w1165]
                i -> [w1188]
                n296 = Subtract(x=w1186, y=w1195) -> (x-y=w1197:dbl)
                n297 = Add(x=1, y=w1188) -> (x+y=→"T loop run":i32)
                n298 = Divide(x="Step(K)", y=1) -> (x/y=w1196:dbl)
                n299 = Divide(x=w1197, y=w1196) -> (x/y=w1194:dbl)
                n300 = Multiply(x=2, y=w1194) -> (x*y=w1193:dbl)
                n301 = Increment(x=w1193) -> (x+1=w1192:dbl)
                n302 = for {
                  N: w1192 -> [_]
                  tunnel: w1196 -> [w1240]
                  shift-right: [w1231] -> w1191
                  shift-left: w1190 -> [w1243]
                  tunnel: w1194 -> [w1238]
                  tunnel: w1195 -> [w1241]
                  tunnel: w1186 -> [w1239]
                  shift-right: [w1222] -> _
                  shift-left: _ -> [w1234]
                  shift-right: [w1233] -> w1185
                  shift-left: w1184 -> [w1232]
                  shift-right: [w1230] -> w1183
                  shift-left: w1182 -> [w1229]
                  shift-right: [w1228] -> w1181
                  shift-left: w1180 -> [w1227]
                  tunnel: w1179 -> [w1226]
                  tunnel: w1178 -> [w1225]
                  tunnel: [w1224] -> w1177
                  tunnel: [w1223] -> w1176
                  tunnel: w1175 -> [w1217]
                  tunnel: w1174 -> [w1216]
                  shift-right: [w1211] -> w1173
                  shift-left: w1172 -> [w1210]
                  shift-right: [w1209] -> w1171
                  shift-left: w1170 -> [w1208]
                  shift-right: [w1207] -> w1169
                  shift-left: w1168 -> [w1206]
                  shift-right: [w1205] -> w1167
                  shift-left: w1166 -> [w1202]
                  shift-right: [w1204] -> _
                  shift-left: _ -> [w1203]
                  tunnel: w1165 -> [w1201]
                  i -> [w1237]
                  n303 = Less Or Equal?(x=w1237, y=w1238) -> (x <= y?=w1242:bool)
                  n304 = case shown="False" w1242 {
                    tunnel: w1241 -> [w1268 w1296]
                    tunnel: w1237 -> [w1277 w1295]
                    tunnel: w1240 -> [w1276 w1294]
                    tunnel: [w1274 w1292] -> w1236
                    tunnel: w1239 -> [w1275 _]
                    tunnel: w1238 -> [w1270 _]
                    tunnel: w1237 -> [w1273 _]
                    frame False {
                      n305 = Multiply(x=w1270, y=2) -> (x*y=w1269:dbl)
                      n306 = Less Or Equal?(x=w1273, y=w1269) -> (x <= y?=w1271:bool)
                      n307 = case shown="False" w1271 {
                        tunnel: w1277 -> [w1284 w1291]
                        tunnel: w1276 -> [w1282 w1289]
                        tunnel: w1275 -> [_ w1287]
                        tunnel: [w1280 w1286] -> w1274
                        tunnel: w1270 -> [_ w1285]
                        tunnel: w1269 -> [w1279 _]
                        tunnel: w1268 -> [w1278 _]
                        frame False {
                          n308 = Subtract(x=w1284, y=w1279) -> (x-y=w1283:dbl)
                          n309 = Multiply(x=w1282, y=w1283) -> (x*y=w1281:dbl)
                          n310 = Add(x=w1278, y=w1281) -> (x+y=w1280:dbl)
                        }
                        frame True {
                          n311 = Subtract(x=w1291, y=w1285) -> (x-y=w1290:dbl)
                          n312 = Multiply(x=w1289, y=w1290) -> (x*y=w1288:dbl)
                          n313 = Subtract(x=w1287, y=w1288) -> (x-y=w1286:dbl)
                        }
                      }
                    }
                    frame True {
                      n314 = Multiply(x=w1294, y=w1295) -> (x*y=w1293:dbl)
                      n315 = Add(x=w1296, y=w1293) -> (x+y=w1292:dbl)
                    }
                  }
                  n316 = Absolute Value(x=w1236) -> (abs(x)=w1235:dbl)
                  n317 = stacked-sequence {
                    tunnel: w1235 -> [w1315 _ _]
                    tunnel: w1243 -> [_ _ w1414]
                    tunnel: [_ _ w1413] -> w1231
                    tunnel: [_ _ w1412] -> w1218
                    tunnel: [_ _ w1411] -> w1222
                    tunnel: w1234 -> [_ _ w1410]
                    tunnel: [_ _ w1409] -> w1219
                    tunnel: [_ _ w1408] -> w1233
                    tunnel: w1232 -> [_ _ w1402]
                    tunnel: [_ _ w1407] -> w1230
                    tunnel: w1229 -> [_ _ w1403]
                    tunnel: [_ _ w1406] -> w1228
                    tunnel: w1227 -> [_ _ w1405]
                    tunnel: [_ _ w1352] -> w1220
                    tunnel: [_ _ w1404] -> w1221
                    tunnel: w1226 -> [w1314 _ _]
                    tunnel: w1225 -> [w1313 _ _]
                    tunnel: [w1299 _ _] -> w1224
                    tunnel: [w1298 _ _] -> w1223
                    tunnel: [_ _ w1349] -> w1215
                    tunnel: [_ _ w1348] -> w1214
                    tunnel: [_ _ w1347] -> w1213
                    tunnel: [_ _ w1346] -> w1212
                    tunnel: [_ _ w1345] -> w1211
                    tunnel: w1210 -> [_ _ w1344]
                    tunnel: [_ _ w1343] -> w1209
                    tunnel: w1208 -> [_ _ w1342]
                    tunnel: [_ _ w1341] -> w1207
                    tunnel: w1206 -> [_ _ w1340]
                    tunnel: [_ _ w1339] -> w1205
                    tunnel: [_ _ w1338] -> w1204
                    tunnel: w1203 -> [_ _ w1337]
                    tunnel: w1202 -> [_ _ w1336]
                    frame #0 {
                      n318 = call "SetTemperature.vi"("Approach"="Sweep Temperature Approach", "Rate"="Sweep T  Rate (K/min)", "Temperature"=w1315, "error in (no error)"=w1313, "Instrument Ref In"=w1314) -> ("error out"=w1311:errorcluster, "Instrument Ref Out"=w1312:refnum<k24>)  [unwired: 2 in, 1 out]
                      n319 = local read "Delay(T/F)"() -> (w1297:dbl)
                      n320 = call "WaitFor.vi"("Delay"=w1297, "Wait For Temperature"=TRUE ("WaitForTemperature"), "error in (no error)"=w1311, "Instrument Ref In"=w1312) -> ("error out"=w1302:errorcluster, "Instrument Ref Out"=w1301:refnum<k24>)  [unwired: 6 in]
                      n321 = for {
                        N: 20 -> [_]
                        shift-right: [w1331] -> _
                        shift-left: TRUE -> [w1329]
                        shift-right: [w1326] -> w1299
                        shift-left: w1302 -> [w1328]
                        tunnel: w1301 -> [w1325]
                        tunnel: [w1323] -> w1298
                        tunnel: [w1320] -> w1308
                        tunnel: [w1319] -> w1307
                        tunnel: [w1321] -> w1305 mode=indexing
                        tunnel: [w1322] -> w1306 mode=indexing
                        n322 = local write "Measuring T"(w1329) -> ()
                        n323 = Not(x=w1329) -> (.not. x?=w1331:bool)
                        n324 = call "GetTemperature.vi"("error in (no error)"=w1328, "Instrument Ref In"=w1325) -> ("Temperature\nStatus"=w1319:i32, "Temperature"=w1322:dbl, "error out"=w1327:errorcluster, "Instrument Ref Out"=w1324:refnum<k24>)  [unwired: 3 in, 1 out]
                        n325 = Wait (ms)(milliseconds to wait=u32 200) -> ()  [unwired: 1 out]
                        n326 = call "GetField.vi"("error in (no error)"=w1327, "Instrument Ref In"=w1324) -> ("Field\nStatus"=w1320:i32, "Field"=w1321:dbl, "error out"=w1326:errorcluster, "Instrument Ref Out"=w1323:refnum<k24>)  [unwired: 3 in, 1 out]
                      }
                      "Field Status" <- w1308
                      "Temp Status" <- w1307
                      n327 = call-poly <vilib>:"Mean.vi"("X"=w1305) -> ("mean"=→"Fixed Field":dbl)  [unwired: 1 out]
                      n328 = call-poly <vilib>:"Mean.vi"("X"=w1306) -> ("mean"=→"Measured Temp":dbl)  [unwired: 1 out]
                      "Temp Setting" <- w1315
                      "Measuring T" <- FALSE
                    }
                    frame #1 {
                      n329 = local read "System Stablization (s)"() -> (w1332:dbl)
                      n330 = Multiply(x=w1332, y=1000) -> (x*y=w1334:dbl)
                      n331 = Wait (ms)(milliseconds to wait=w1334) -> ()  [unwired: 1 out]
                    }
                    frame #2 {
                      n332 = local read "LOCKIN1 address"() -> (w1351:refnum<visa-resource-name>)
                      n333 = local read "Two Lock-in ?"() -> (w1350:bool)
                      n334 = flat-sequence {
                        tunnel: w1414 -> [w1612]
                        tunnel: w1351 -> [w1586]
                        tunnel: w1410 -> [w1611]
                        tunnel: w1405 -> [w1603]
                        tunnel: [w1609] -> w1401
                        tunnel: [w1597] -> w1399
                        tunnel: [w1598] -> w1397
                        tunnel: [w1595] -> w1395
                        tunnel: [w1598] -> w1393
                        tunnel: [w1598] -> w1391
                        tunnel: [w1598] -> w1389
                        tunnel: [w1598] -> w1387
                        tunnel: [w1597] -> w1385
                        tunnel: [w1596] -> w1383
                        tunnel: [w1595] -> w1381
                        tunnel: [w1594] -> w1379
                        tunnel: ["T Clear Plot 1B"] -> w1377
                        tunnel: ["T Clear Plot 1A"] -> w1375
                        tunnel: [w1591] -> w1373
                        tunnel: [w1590] -> w1371
                        tunnel: [w1589] -> w1369
                        tunnel: [w1588] -> w1367
                        tunnel: [w1587] -> w1365
                        tunnel: w1335 -> [w1585]
                        tunnel: w1401 -> [w1634]
                        tunnel: [w1634] -> w1400
                        tunnel: w1399 -> [w1633]
                        tunnel: [w1633] -> w1398
                        tunnel: w1397 -> [w1632]
                        tunnel: [w1632] -> w1396
                        tunnel: w1395 -> [w1631]
                        tunnel: [w1631] -> w1394
                        tunnel: w1393 -> [w1630]
                        tunnel: [w1630] -> w1392
                        tunnel: w1391 -> [w1629]
                        tunnel: [w1629] -> w1390
                        tunnel: w1389 -> [w1628]
                        tunnel: [w1628] -> w1388
                        tunnel: w1387 -> [w1627]
                        tunnel: [w1627] -> w1386
                        tunnel: w1385 -> [w1626]
                        tunnel: [w1626] -> w1384
                        tunnel: w1383 -> [w1625]
                        tunnel: [w1625] -> w1382
                        tunnel: w1381 -> [w1624]
                        tunnel: [w1624] -> w1380
                        tunnel: w1379 -> [w1623]
                        tunnel: [w1623] -> w1378
                        tunnel: w1377 -> [w1622]
                        tunnel: [w1622] -> w1376
                        tunnel: w1375 -> [w1621]
                        tunnel: [w1621] -> w1374
                        tunnel: w1373 -> [w1620]
                        tunnel: [w1620] -> w1372
                        tunnel: w1371 -> [w1619]
                        tunnel: [w1619] -> w1370
                        tunnel: w1369 -> [w1618]
                        tunnel: [w1618] -> w1368
                        tunnel: w1367 -> [w1617]
                        tunnel: [w1617] -> w1366
                        tunnel: w1365 -> [w1616]
                        tunnel: [w1616] -> w1364
                        tunnel: w1400 -> [w1638]
                        tunnel: w1398 -> [w1672]
                        tunnel: w1396 -> [w1671]
                        tunnel: w1394 -> [w1670]
                        tunnel: w1392 -> [w1669]
                        tunnel: w1390 -> [w1667]
                        tunnel: w1388 -> [w1665]
                        tunnel: w1386 -> [w1663]
                        tunnel: w1384 -> [w1660]
                        tunnel: w1382 -> [w1659]
                        tunnel: w1380 -> [w1656]
                        tunnel: w1378 -> [w1655]
                        tunnel: w1403 -> [w1653]
                        tunnel: w1376 -> [w1652]
                        tunnel: w1402 -> [w1650]
                        tunnel: w1374 -> [w1649]
                        tunnel: w1372 -> [w1645]
                        tunnel: w1370 -> [w1644]
                        tunnel: w1368 -> [w1643]
                        tunnel: w1366 -> [w1640]
                        tunnel: w1364 -> [w1639]
                        tunnel: [w1638] -> w1363
                        tunnel: [w1658] -> w1362
                        tunnel: [w1672] -> w1361
                        tunnel: [w1671] -> w1360
                        tunnel: [w1636] -> w1359
                        tunnel: [w1637] -> w1358
                        tunnel: [w1661] -> w1357
                        tunnel: [w1657] -> w1356
                        tunnel: [w1654] -> w1355
                        tunnel: [w1670] -> w1354
                        tunnel: [w1642] -> w1353
                        tunnel: [w1676] -> w1404
                        tunnel: [w1677] -> w1352
                        tunnel: [w1674] -> w1406
                        tunnel: [w1678] -> w1407
                        tunnel: [w1679] -> w1408
                        tunnel: [w1680] -> _
                        tunnel: [w1681] -> w1409
                        tunnel: [w1682] -> w1411
                        tunnel: [w1683] -> w1412
                        tunnel: [w1673] -> w1413
                        tunnel: [w1684] -> _
                        tunnel: w1363 -> [w1684]
                        tunnel: w1362 -> [w1673]
                        tunnel: w1361 -> [w1683]
                        tunnel: w1360 -> [w1682]
                        tunnel: w1359 -> [w1681]
                        tunnel: w1358 -> [w1680]
                        tunnel: w1357 -> [w1679]
                        tunnel: w1356 -> [w1678]
                        tunnel: w1355 -> [w1674]
                        tunnel: w1354 -> [w1677]
                        tunnel: w1353 -> [w1676]
                        frame #0 {
                          w1590 = u8 1 items=["Channel A", "Channel B"] ("Channel A/B for Parameter1")
                          w1587 = u8 0 items=["Channel A", "Channel B"] ("Channel A/B for Parameter1")
                          n335 = Format Into String(0) -> (error out=w1610:errorcluster)  [unwired: 3 in, 1 out]
                          n336 = Format Into String(0) -> (error out=w1605:errorcluster)  [unwired: 3 in, 1 out]
                          n337 = call "OE1022D_Read 1 parameter_mean.vi"("错误输入（无错误）"=w1610, "Parameter"="Parameter 1A", "Channel (0: A)"=w1587, "VISA resource name"=w1586) -> ("error out"=w1588:errorcluster, "Measurement"=w1600:dbl, "VISA resource name out"=w1609:refnum<visa-resource-name>)  [unwired: 5 in]
                          n338 = call "OE1022D_Read 1 parameter_mean.vi"("Parameter 2"="Parameter 1B", "错误输入（无错误）"=w1605, "Channel (0: A)"=w1590, "VISA resource name"=w1586) -> ("error out"=w1591:errorcluster, "Measurement"=w1599:dbl, "VISA resource name out"=w1589:refnum<visa-resource-name>)  [unwired: 5 in]
                          n339 = Multiply(x=w1600, y=1000.0) -> (x*y=w1597:dbl)
                          "para1A Measurement (mV)" <- w1597
                          n340 = Multiply(x=w1599, y=1000000.0) -> (x*y=w1595:dbl)
                          "para1B Measurement (uV)" <- w1595
                          n341 = Build Array(w1597) -> (w1613:dbl[])
                          n342 = Build Array(w1595) -> (w1606:dbl[])
                          n343 = Select(t=w1613, s="T Clear Plot 1A", f=w1612) -> (s? t:f=w1596:dbl[])
                          n344 = Select(t=w1606, s="T Clear Plot 1B", f=w1603) -> (s? t:f=w1594:dbl[])
                          n345 = Build Array (concatenate)(w1585, w1611) -> (w1598:dbl[])
                        }
                        frame #1 {
                          n346 = Wait (ms)(milliseconds to wait=u32 50) -> ()  [unwired: 1 out]
                        }
                        frame #2 {
                          n347 = Build Array (concatenate)(w1660, w1659) -> (w1658:dbl[])
                          n348 = Build Array (concatenate)(w1656, w1655) -> (w1654:dbl[])
                          n349 = Bundle(w1665, w1658) -> (→"P1A-T":cluster{dbl[], dbl[]})  [unwired: 1 in]
                          n350 = Bundle(w1667, w1654) -> (→"P1B-T":cluster{dbl[], dbl[]})  [unwired: 1 in]
                          n351 = call "OE1022D_Read 1 parameter_mean.vi"("错误输入（无错误）"=w1640, "Parameter"="Phase 1A", "Channel (0: A)"=w1639, "VISA resource name"=w1638) -> ("error out"=w1637:errorcluster, "Measurement"=w1636:dbl)  [unwired: 5 in, 1 out]
                          "phase 1A" <- w1636
                          n352 = call "OE1022D_Read 1 parameter_mean.vi"("Parameter 2"="Phase 1B", "错误输入（无错误）"=w1645, "Channel (0: A)"=w1644, "VISA resource name"=w1643) -> ("Measurement"=w1642:dbl)  [unwired: 5 in, 2 out]
                          "phase 1B" <- w1642
                          n353 = Build Array(w1636) -> (w1646:dbl[])
                          n354 = Build Array(w1642) -> (w1647:dbl[])
                          n355 = Select(t=w1646, s=w1649, f=w1650) -> (s? t:f=w1648:dbl[])
                          n356 = Select(t=w1647, s=w1652, f=w1653) -> (s? t:f=w1651:dbl[])
                          n357 = Build Array (concatenate)(w1636, w1648) -> (w1661:dbl[])
                          n358 = Build Array (concatenate)(w1642, w1651) -> (w1657:dbl[])
                          n359 = Bundle(w1663, w1661) -> (→"Phase1A-T":cluster{dbl[], dbl[]})  [unwired: 1 in]
                          n360 = Bundle(w1669, w1657) -> (→"Phase1B-T":cluster{dbl[], dbl[]})  [unwired: 1 in]
                        }
                        frame #3 {
                          n361 = Wait (ms)(milliseconds to wait=u32 50) -> ()  [unwired: 1 out]
                        }
                      }
                      n362 = local read "Measured Temp"() -> (w1335:dbl)
                      n363 = case shown="True" w1350 {
                        tunnel: [w1416 w1435] -> w1349
                        tunnel: [w1416 w1434] -> w1348
                        tunnel: [w1416 w1433] -> w1346
                        tunnel: [w1416 w1432] -> w1347
                        tunnel: [w1419 w1431] -> w1339
                        tunnel: [w1415 w1430] -> w1338
                        tunnel: w1337 -> [w1415 w1429]
                        tunnel: w1336 -> [w1419 w1426]
                        tunnel: [w1420 w1428] -> w1345
                        tunnel: w1344 -> [w1420 w1427]
                        tunnel: [w1418 w1425] -> w1343
                        tunnel: w1342 -> [w1418 w1424]
                        tunnel: [w1417 w1423] -> w1341
                        tunnel: w1340 -> [w1417 w1422]
                        tunnel: w1335 -> [_ w1421]
                        frame False {
                          w1416 = nan
                        }
                        frame True {
                          n364 = flat-sequence {
                            tunnel: w1429 -> [w1487]
                            tunnel: [w1511] -> w1484
                            tunnel: [w1505] -> w1483
                            tunnel: [w1486] -> w1482
                            tunnel: [w1503] -> w1481
                            tunnel: [w1486] -> w1480
                            tunnel: [w1486] -> w1479
                            tunnel: [w1486] -> w1478
                            tunnel: [w1486] -> w1477
                            tunnel: [w1505] -> w1476
                            tunnel: [w1504] -> w1475
                            tunnel: [w1503] -> w1474
                            tunnel: [w1502] -> w1473
                            tunnel: ["T Clear Plot 2B"] -> w1472
                            tunnel: ["T Clear Plot 2A"] -> w1471
                            tunnel: [w1493] -> w1470
                            tunnel: [w1495] -> w1469
                            tunnel: [w1494] -> w1468
                            tunnel: [w1499] -> w1467
                            tunnel: [w1498] -> w1466
                            tunnel: w1427 -> [w1489]
                            tunnel: w1424 -> [w1488]
                            tunnel: w1421 -> [w1485]
                            tunnel: w1484 -> [w1534]
                            tunnel: [w1534] -> w1465
                            tunnel: w1483 -> [w1533]
                            tunnel: [w1533] -> w1464
                            tunnel: w1482 -> [w1532]
                            tunnel: [w1532] -> w1463
                            tunnel: w1481 -> [w1531]
                            tunnel: [w1531] -> w1462
                            tunnel: w1480 -> [w1530]
                            tunnel: [w1530] -> w1461
                            tunnel: w1479 -> [w1529]
                            tunnel: [w1529] -> w1460
                            tunnel: w1478 -> [w1528]
                            tunnel: [w1528] -> w1459
                            tunnel: w1477 -> [w1527]
                            tunnel: [w1527] -> w1458
                            tunnel: w1476 -> [w1526]
                            tunnel: [w1526] -> w1457
                            tunnel: w1475 -> [w1525]
                            tunnel: [w1525] -> w1456
                            tunnel: w1474 -> [w1524]
                            tunnel: [w1524] -> w1455
                            tunnel: w1473 -> [w1523]
                            tunnel: [w1523] -> w1454
                            tunnel: w1472 -> [w1522]
                            tunnel: [w1522] -> w1453
                            tunnel: w1471 -> [w1521]
                            tunnel: [w1521] -> w1452
                            tunnel: w1470 -> [w1520]
                            tunnel: [w1520] -> w1451
                            tunnel: w1469 -> [w1519]
                            tunnel: [w1519] -> w1450
                            tunnel: w1468 -> [w1518]
                            tunnel: [w1518] -> w1449
                            tunnel: w1467 -> [w1517]
                            tunnel: [w1517] -> w1448
                            tunnel: w1466 -> [w1516]
                            tunnel: [w1516] -> w1447
                            tunnel: w1465 -> [w1539]
                            tunnel: w1464 -> [w1572]
                            tunnel: w1463 -> [w1571]
                            tunnel: w1462 -> [w1570]
                            tunnel: w1461 -> [w1569]
                            tunnel: w1460 -> [w1567]
                            tunnel: w1459 -> [w1565]
                            tunnel: w1458 -> [w1563]
                            tunnel: w1457 -> [w1560]
                            tunnel: w1456 -> [w1559]
                            tunnel: w1455 -> [w1556]
                            tunnel: w1454 -> [w1555]
                            tunnel: w1453 -> [w1553]
                            tunnel: w1422 -> [w1551]
                            tunnel: w1452 -> [w1550]
                            tunnel: w1451 -> [w1546]
                            tunnel: w1450 -> [w1545]
                            tunnel: w1449 -> [w1544]
                            tunnel: w1448 -> [w1541]
                            tunnel: w1447 -> [w1540]
                            tunnel: [w1539] -> w1446
                            tunnel: [w1558] -> w1445
                            tunnel: [w1572] -> w1444
                            tunnel: [w1571] -> w1443
                            tunnel: [w1537] -> w1442
                            tunnel: [w1538] -> w1441
                            tunnel: [w1561] -> w1440
                            tunnel: [w1557] -> w1439
                            tunnel: [w1554] -> w1438
                            tunnel: [w1570] -> w1437
                            tunnel: [w1543] -> w1436
                            tunnel: w1426 -> [w1535]
                            tunnel: [w1575] -> w1432
                            tunnel: [w1576] -> w1434
                            tunnel: [w1577] -> w1425
                            tunnel: [w1578] -> w1431
                            tunnel: [w1579] -> w1423
                            tunnel: [w1580] -> _
                            tunnel: [w1581] -> w1433
                            tunnel: [w1582] -> w1430
                            tunnel: [w1583] -> w1428
                            tunnel: [w1584] -> _
                            tunnel: w1446 -> [w1584]
                            tunnel: w1445 -> [w1583]
                            tunnel: w1444 -> [w1573]
                            tunnel: w1443 -> [w1582]
                            tunnel: w1442 -> [w1581]
                            tunnel: w1441 -> [w1580]
                            tunnel: w1440 -> [w1579]
                            tunnel: w1439 -> [w1578]
                            tunnel: w1438 -> [w1577]
                            tunnel: w1437 -> [w1576]
                            tunnel: w1436 -> [w1575]
                            tunnel: [w1573] -> w1435
                            frame #0 {
                              w1495 = u8 1 items=["Channel A", "Channel B"] ("Channel A/B for Parameter1")
                              w1498 = u8 0 items=["Channel A", "Channel B"] ("Channel A/B for Parameter1")
                              n365 = local read "LOCKIN2 address"() -> (w1490:refnum<visa-resource-name>)
                              n366 = Format Into String(0) -> (error out=w1512:errorcluster)  [unwired: 3 in, 1 out]
                              n367 = Format Into String(0) -> (error out=w1496:errorcluster)  [unwired: 3 in, 1 out]
                              n368 = call "OE1022D_Read 1 parameter_mean.vi"("错误输入（无错误）"=w1512, "Parameter"="Parameter 2A", "Channel (0: A)"=w1498, "VISA resource name"=w1490) -> ("error out"=w1499:errorcluster, "Measurement"=w1506:dbl, "VISA resource name out"=w1511:refnum<visa-resource-name>)  [unwired: 5 in]
                              n369 = call "OE1022D_Read 1 parameter_mean.vi"("Parameter 2"="Parameter 2B", "错误输入（无错误）"=w1496, "Channel (0: A)"=w1495, "VISA resource name"=w1490) -> ("error out"=w1493:errorcluster, "Measurement"=w1492:dbl, "VISA resource name out"=w1494:refnum<visa-resource-name>)  [unwired: 5 in]
                              n370 = Multiply(x=w1506, y=1000.0) -> (x*y=w1505:dbl)
                              "para2A Measurement" <- w1505
                              n371 = Multiply(x=w1492, y=1000000.0) -> (x*y=w1503:dbl)
                              "para2B Measurement" <- w1503
                              n372 = Build Array(w1505) -> (w1513:dbl[])
                              n373 = Build Array(w1503) -> (w1508:dbl[])
                              n374 = Select(t=w1513, s="T Clear Plot 2A", f=w1489) -> (s? t:f=w1504:dbl[])
                              n375 = Select(t=w1508, s="T Clear Plot 2B", f=w1488) -> (s? t:f=w1502:dbl[])
                              n376 = Build Array (concatenate)(w1485, w1487) -> (w1486:dbl[])
                            }
                            frame #1 {
                              n377 = Wait (ms)(milliseconds to wait=u32 50) -> ()  [unwired: 1 out]
                            }
                            frame #2 {
                              n378 = Build Array (concatenate)(w1560, w1559) -> (w1558:dbl[])
                              n379 = Build Array (concatenate)(w1556, w1555) -> (w1554:dbl[])
                              n380 = Bundle(w1565, w1558) -> (→"XY Graph 7":cluster{dbl[], dbl[]})  [unwired: 1 in]
                              n381 = Bundle(w1567, w1554) -> (→"XY Graph 5":cluster{dbl[], dbl[]})  [unwired: 1 in]
                              n382 = call "OE1022D_Read 1 parameter_mean.vi"("错误输入（无错误）"=w1541, "Parameter"="Phase 2A", "Channel (0: A)"=w1540, "VISA resource name"=w1539) -> ("error out"=w1538:errorcluster, "Measurement"=w1537:dbl)  [unwired: 5 in, 1 out]
                              "phase 2A" <- w1537
                              n383 = call "OE1022D_Read 1 parameter_mean.vi"("Parameter 2"="Phase 2B", "错误输入（无错误）"=w1546, "Channel (0: A)"=w1545, "VISA resource name"=w1544) -> ("Measurement"=w1543:dbl)  [unwired: 5 in, 2 out]
                              "phase 2B" <- w1543
                              n384 = Build Array(w1537) -> (w1547:dbl[])
                              n385 = Build Array(w1543) -> (w1548:dbl[])
                              n386 = Select(t=w1547, s=w1550, f=w1551) -> (s? t:f=w1549:dbl[])
                              n387 = Select(t=w1548, s=w1553, f=w1535) -> (s? t:f=w1552:dbl[])
                              n388 = Build Array (concatenate)(w1537, w1549) -> (w1561:dbl[])
                              n389 = Build Array (concatenate)(w1543, w1552) -> (w1557:dbl[])
                              n390 = Bundle(w1563, w1561) -> (→"XY Graph 8":cluster{dbl[], dbl[]})  [unwired: 1 in]
                              n391 = Bundle(w1569, w1557) -> (→"XY Graph 6":cluster{dbl[], dbl[]})  [unwired: 1 in]
                            }
                            frame #3 {
                              n392 = Wait (ms)(milliseconds to wait=u32 50) -> ()  [unwired: 1 out]
                            }
                          }
                        }
                      }
                    }
                  }
                  n393 = case shown="True" w1216 {
                    tunnel: w1218 -> [_ w1254]
                    tunnel: w1217 -> [_ w1257]
                    tunnel: w1219 -> [_ w1253]
                    tunnel: w1220 -> [_ w1252]
                    tunnel: w1221 -> [_ w1251]
                    tunnel: w1215 -> [_ w1248]
                    tunnel: w1214 -> [_ w1247]
                    tunnel: w1213 -> [_ w1246]
                    tunnel: w1212 -> [_ w1245]
                    tunnel: w1201 -> [_ w1244]
                    frame False {
                    }
                    frame True {
                      n394 = local read "Measured Temp"() -> (w1249:dbl)
                      n395 = local read "Two Lock-in ?"() -> (w1250:bool)
                      n396 = case shown="True" w1250 {
                        tunnel: w1249 -> [_ w1264]
                        tunnel: w1248 -> [_ w1263]
                        tunnel: w1245 -> [_ w1262]
                        tunnel: w1246 -> [_ w1261]
                        tunnel: w1247 -> [_ w1260]
                        tunnel: w1244 -> [_ w1259]
                        frame False {
                        }
                        frame True {
                          n397 = Build Array(w1264, w1263, w1260, w1262, w1261) -> (w1266:dbl[])
                          n398 = call-poly <vilib>:"Write Delimited Spreadsheet.vi"("file path (dialog if empty)"=w1259, "format (%.3f)"="%.10f", "1D data"=w1266, "append to file? (new file:F)"=TRUE) -> ()  [unwired: 10 in, 2 out]
                        }
                      }
                      n399 = Build Array(w1249, w1254, w1253, w1252, w1251) -> (w1256:dbl[])
                      n400 = call-poly <vilib>:"Write Delimited Spreadsheet.vi"("file path (dialog if empty)"=w1257, "format (%.3f)"="%.10f", "1D data"=w1256, "append to file? (new file:F)"=TRUE) -> ()  [unwired: 10 in, 2 out]
                    }
                  }
                }
              }
            }
          }
        }
      }
    }
    frame #2 {
      n401 = case shown="True" "Initialize" {
        tunnel: w1687 -> [w1688 w1691]
        tunnel: w1686 -> [w1689 w1690]
        frame False {
          n402 = Close Reference(reference=w1689, error in (no error)=w1688) -> ()  [unwired: 1 out]
        }
        frame True {
          w1697 = 0 items=["Linear", "NoOvershoot", "Oscillate"] ("Approach")
          w1698 = 0 items=["Persistent", "Driven"] ("Mode")
          w1694 = 0 items=["FastSettle", "NoOvershoot"] ("Approach")
          n403 = call "SetTemperature.vi"("Approach"=w1694, "Rate"=20.0, "Temperature"=120.0, "error in (no error)"=w1691, "Instrument Ref In"=w1690) -> ("error out"=w1702:errorcluster, "Instrument Ref Out"=w1701:refnum<k24>)  [unwired: 2 in, 1 out]
          n404 = call "SetField.vi"("Mode"=w1698, "Approach"=w1697, "Rate"=200.0, "Field"=0.0, "error in (no error)"=w1702, "Instrument Ref In"=w1701) -> ("error out"=w1699:errorcluster, "Instrument Ref Out"=w1700:refnum<k24>)  [unwired: 1 in, 1 out]
          n405 = Close Reference(reference=w1700, error in (no error)=w1699) -> ()  [unwired: 1 out]
        }
      }
    }
  }
  n406 = while {
    tunnel: w34 -> [w1705]
    tunnel: w33 -> [w1704]
    stop <- "?" stop-if-true
    n407 = for {
      N: 10 -> [_]
      shift-right: [w1720] -> _
      shift-left: w1704 -> [w1722]
      tunnel: w1705 -> [w1719]
      tunnel: [w1717] -> _
      tunnel: [w1714] -> w1711
      tunnel: [w1713] -> w1710
      tunnel: [w1715] -> w1708 mode=indexing
      tunnel: [w1716] -> w1709 mode=indexing
      n408 = call "GetTemperature.vi"("error in (no error)"=w1722, "Instrument Ref In"=w1719) -> ("Temperature\nStatus"=w1713:i32, "Temperature"=w1716:dbl, "error out"=w1721:errorcluster, "Instrument Ref Out"=w1718:refnum<k24>)  [unwired: 3 in, 1 out]
      n409 = Wait (ms)(milliseconds to wait=u32 200) -> ()  [unwired: 1 out]
      n410 = call "GetField.vi"("error in (no error)"=w1721, "Instrument Ref In"=w1718) -> ("Field\nStatus"=w1714:i32, "Field"=w1715:dbl, "error out"=w1720:errorcluster, "Instrument Ref Out"=w1717:refnum<k24>)  [unwired: 3 in, 1 out]
    }
    "Field Status" <- w1711
    "Temperature Status" <- w1710
    n411 = call-poly <vilib>:"Mean.vi"("X"=w1708) -> ("mean"=→"Field":dbl)  [unwired: 1 out]
    n412 = call-poly <vilib>:"Mean.vi"("X"=w1709) -> ("mean"=→"Temperature":dbl)  [unwired: 1 out]
  }
  n413 = local read "Sweep T/F"() -> (w30:bool)
  n414 = case shown="True" w30 {
    tunnel: [w1726 w1729] -> w29
    tunnel: ["K" "Oe"] -> w17
    tunnel: ["Oe" "K"] -> w16
    frame False {
      n415 = local read "Set Fixed T"() -> (w1726:dbl)
    }
    frame True {
      n416 = local read "Set FIxed F (Oe)"() -> (w1729:dbl)
    }
  }
  n417 = local read "R1(Kohm)"() -> (w4:dbl)
  n418 = local read "R2(Kohm)"() -> (w3:dbl)
  n419 = Format Into String(format string="%.3fKohm", w4) -> (resulting string=w2:string)  [unwired: 2 in, 1 out]
  n420 = Format Into String(format string="%.3fKohm", w3) -> (resulting string=w1:string)  [unwired: 2 in, 1 out]
  n421 = Format Into String(format string="%.1f", w29) -> (resulting string=w18:string)  [unwired: 2 in, 1 out]
  n422 = local read "1A frequency"() -> (w11:dbl)
  n423 = local read "Sine Output Amplitude (V)"() -> (w15:sgl)
  n424 = local read "2A frequency"() -> (w9:dbl)
  n425 = Format Into String(format string="%.1fHz", w11) -> (resulting string=w8:string)  [unwired: 2 in, 1 out]
  n426 = Format Into String(format string="%.1fHz", w9) -> (resulting string=w7:string)  [unwired: 2 in, 1 out]
  n427 = Format Into String(format string="%.1fV", w15) -> (resulting string=w13:string)  [unwired: 2 in, 1 out]
  n428 = Format Into String(initial string="path1 (folder + filename)", w18, w17, "Sweep", w16, w8, w2, w13, ".txt") -> (resulting string=w32:string)  [unwired: 2 in, 1 out]
  n429 = String To Path(string=w32) -> (path=w26:path)
  n430 = Format Into String(initial string="path2 (folder + filename)", w18, w17, "Sweep", w16, w7, w1, w13, ".txt") -> (resulting string=w20:string)  [unwired: 2 in, 1 out]
  n431 = String To Path(string=w20) -> (path=w19:path)
